vi "Lab Panel V2.9.vi"() -> ()   [LabVIEW 2013]
uses:
  <vilib>/Platform/TimedLoop/XDataNode/timing_clust.ctl
  <vilib>/Platform/TimedLoop/XDataNode/nitl_modes.ctl
  <vilib>/Platform/TimedLoop/XDataNode/wakeup.ctl
  <vilib>/platform/TimedLoop/XDataNode/XDataNode.xnode
  <vilib>/Platform/TimedLoop/XDataNode/XDNodeRunTimeDep.lvlib
panel:
  out "TEMP update":bool
  out "AI update":bool
  in  "stop":bool
  in  "Tab Control 2":T1(tab)
  out "LAB05-2 (SIG)":T2 {"PF" format="%.2f"; "AMPS" format="%.1f"}
  out "LAB05-1 (SIG)":T2 {"PF" format="%.2f"; "AMPS" format="%.1f"}
  out "LAB04-2 (SIG)":T2 {"PF" format="%.2f"; "AMPS" format="%.1f"}
  out "LAB04-1 (SIG)":T2 {"PF" format="%.2f"; "AMPS" format="%.1f"}
  out "LAB03-2 (SIG)":T2 {"PF" format="%.2f"; "AMPS" format="%.1f"}
  out "LAB03-1 (SIG)":T2 {"PF" format="%.2f"; "AMPS" format="%.1f"}
  out "LAB02-2 (SIG)":T2 {"PF" format="%.2f"; "AMPS" format="%.1f"}
  in  "LAB01-1RUN":bool
  in  "LAB05-1 (O/I)":bool
  in  "LAB05-2 (O/I)":bool
  in  "LAB04-1 (O/I)":bool
  in  "LAB04-2 (O/I)":bool
  in  "LAB02-1 (O/I)":bool
  in  "LAB02-2 (O/I)":bool
  in  "LAB01-2 (O/I)":bool
  in  "LAB01-1 (O/I)":bool
  in  "LAB03-1 (O/I)":bool
  in  "LAB05-2 RUN":bool
  in  "LAB05-1 RUN":bool
  in  "LAB04-2 RUN":bool
  in  "LAB04-1 RUN":bool
  in  "LAB03-2 RUN":bool
  in  "LAB03-1 RUN":bool
  in  "LAB02-2 RUN":bool
  in  "LAB02-1 RUN":bool
  in  "LAB01-2 RUN":bool
  in  "LAB05-2 SELECT":T3(radio)
  in  "LAB05-1 SELECT":T3(radio)
  in  "LAB04-2 SELECT":T3(radio)
  in  "LAB04-1 SELECT":T3(radio)
  in  "LAB03-2 SELECT":T3(radio)
  in  "LAB03-1 SELECT":T3(radio)
  in  "LAB02-2 SELECT":T3(radio)
  in  "LAB02-1 SELECT":T3(radio)
  in  "LAB01-2 SELECT":T3(radio)
  in  "LAB01-1 SELECT":T3(radio)
  in  "LAB03-2 (O/I)":bool
  out "LAB01-1 (SIG)":T2 {"PF" format="%.2f"; "AMPS" format="%.1f"}
  out "LAB01-2 (SIG)":T2 {"PF" format="%.2f"; "AMPS" format="%.1f"}
  out "LAB02-1 (SIG)":T2 {"PF" format="%.2f"; "AMPS" format="%.1f"}
  out "LAB05-2 (DISP)":T4 {"MINS" format="%.2g"}
  out "LAB05-1 (DISP)":T4 {"MINS" format="%.2g"}
  out "LAB04-2 (DISP)":T4 {"MINS" format="%.2g"}
  out "LAB04-1 (DISP)":T4 {"MINS" format="%.2g"}
  out "LAB03-2 (DISP)":T4 {"MINS" format="%.2g"}
  out "LAB03-1 (DISP)":T4 {"MINS" format="%.2g"}
  in  "LAB05-2 (SET)":T5
  in  "LAB05-1 (SET)":T5
  in  "LAB04-2 (SET)":T5
  in  "LAB04-1 (SET)":T5
  in  "LAB03-2 (SET)":T5
  in  "LAB03-1 (SET)":T5
  out "LAB02-2 (DISP)":T4 {"MINS" format="%.2g"}
  out "LAB02-1 (DISP)":T4 {"MINS" format="%.2g"}
  in  "LAB02-2 (SET)":T5
  in  "LAB02-1 (SET)":T5
  out "LAB05-2 (RESULT)":bool
  out "LAB05-1 (RESULT)":bool
  out "LAB04-2 (RESULT)":bool
  out "LAB04-1 (RESULT)":bool
  out "LAB03-2 (RESULT)":bool
  out "LAB03-1 (RESULT)":bool
  out "LAB02-2 (RESULT)":bool
  out "LAB02-1 (RESULT)":bool
  out "LAB01-2 (RESULT)":bool
  out "LAB01-1 (RESULT)":bool
  in  "LAB01-1 (SET)":T5
  in  "LAB01-2(SET)":T5
  out "LAB01-1 (DISP)":T4 {"MINS" format="%.2g"}
  out "LAB01-2 (DISP)":T4 {"MINS" format="%.2f"}
  out "LAB05-2 (FAIL)":cluster{"LO":dbl, "HI":dbl}
  out "LAB05-1 (FAIL)":cluster{"LO":dbl, "HI":dbl}
  out "LAB04-2 (FAIL)":cluster{"LO":dbl, "HI":dbl}
  out "LAB04-1 (FAIL)":cluster{"LO":dbl, "HI":dbl}
  out "LAB03-2 (FAIL)":cluster{"LO":dbl, "HI":dbl}
  out "LAB03-1 (FAIL)":cluster{"LO":dbl, "HI":dbl}
  out "LAB02-2 (FAIL)":cluster{"LO":dbl, "HI":dbl}
  out "LAB02-1 (FAIL)":cluster{"LO":dbl, "HI":dbl}
  out "LAB01-2 (FAIL)":cluster{"LO":dbl, "HI":dbl}
  out "LAB01-1 (FAIL)":cluster{"LO":dbl, "HI":dbl}
  out "LAB05-2 (TEMP START)":cluster{"TL":dbl, "TN":dbl}
  out "LAB04-2 (TEMP START)":cluster{"TL":dbl, "TN":dbl}
  out "LAB03-2 (TEMP START)":cluster{"TL":dbl, "TN":dbl}
  out "LAB02-2 (TEMP START)":cluster{"TL":dbl, "TN":dbl}
  out "LAB01-2 (TEMP START)":cluster{"TL":dbl, "TN":dbl}
  out "LAB05-1 (TEMP START)":cluster{"TL":dbl, "TN":dbl}
  out "LAB04-1 (TEMP START)":cluster{"TL":dbl, "TN":dbl}
  out "LAB03-1 (TEMP START)":cluster{"TL":dbl, "TN":dbl}
  out "LAB02-1 (TEMP START)":cluster{"TL":dbl, "TN":dbl}
  out "LAB01-1 (TEMP START)":cluster{"TL":dbl, "TN":dbl}
  in  "JIG ON TIME (S)":dbl=1.0 min=1.0 max=10.0 step=0.5 format="%.1g"
  in  "JIG OFF TIME (S)":dbl=2.0 min=2.0 max=10.0 step=0.5 format="%.1g"
  out "LAB01-1 (JIG)":bool
  out "LAB01-2 (JIG)":bool
  out "LAB02-1 (JIG)":bool
  out "LAB02-2 (JIG)":bool
  out "LAB03-1 (JIG)":bool
  out "LAB03-2 (JIG)":bool
  out "LAB04-1 (JIG)":bool
  out "LAB04-2 (JIG)":bool
  out "LAB05-1 (JIG)":bool
  out "LAB05-2 (JIG)":bool
  out "LAB01 (CAL)":T6 {"2 (TN) cal" min=0.0 step=0.01 format="%.2f"; "2 (TL) cal" min=0.0 step=0.01 format="%.2f"; "2 (PF) cal" min=0.0 step=0.01 format="%.2f"; "2 (V) cal" min=0.0 step=0.01 format="%.2f"; "2 (A) cal" min=0.0 step=0.01 format="%.2f"; "1 (TN) cal" min=0.0 step=0.01 format="%.2f"; "1 (TL) cal" min=0.0 step=0.01 format="%.2f"; "1 (PF) cal" min=0.0 step=0.01 format="%.2f"; "1 (V) cal" min=0.0 step=0.01 format="%.2f"; "1  (A) cal" min=0.0 step=0.01 format="%.2f"}
  out "LAB03 (CAL)":T6 {"2 (TN) cal" min=0.0 step=0.01 format="%.2f"; "2 (TL) cal" min=0.0 step=0.01 format="%.2f"; "2 (PF) cal" min=0.0 step=0.01 format="%.2f"; "2 (V) cal" min=0.0 step=0.01 format="%.2f"; "2 (A) cal" min=0.0 step=0.01 format="%.2f"; "1 (TN) cal" min=0.0 step=0.01 format="%.2f"; "1 (TL) cal" min=0.0 step=0.01 format="%.2f"; "1 (PF) cal" min=0.0 step=0.01 format="%.2f"; "1 (V) cal" min=0.0 step=0.01 format="%.2f"; "1  (A) cal" min=0.0 step=0.01 format="%.2f"}
  out "LAB02 (CAL)":T7 {"2 (TN) cal" min=0.0 step=0.01 format="%.2f"; "2 (TL) cal" min=0.0 step=0.01 format="%.2f"; "2 (PF) cal" min=0.0 step=0.01 format="%.2f"; "2 (V) cal" min=0.0 step=0.01 format="%.2f"; "2 (A) cal" min=0.0 step=0.01 format="%.2f"; "1 (TN) cal" min=0.0 step=0.01 format="%.2f"; "1 (TL) cal" min=0.0 step=0.01 format="%.2f"; "1 (PF) cal" min=0.0 step=0.01 format="%.2f"; "1 (V) cal" min=0.0 step=0.01 format="%.2f"; "1 (A) cal" min=0.0 step=0.01 format="%.2f"}
  out "LAB05 (CAL)":T6 {"2 (TN) cal" min=0.0 step=0.01 format="%.2f"; "2 (TL) cal" min=0.0 step=0.01 format="%.2f"; "2 (PF) cal" min=0.0 step=0.01 format="%.2f"; "2 (V) cal" min=0.0 step=0.01 format="%.2f"; "2 (A) cal" min=0.0 step=0.01 format="%.2f"; "1 (TN) cal" min=0.0 step=0.01 format="%.2f"; "1 (TL) cal" min=0.0 step=0.01 format="%.2f"; "1 (PF) cal" min=0.0 step=0.01 format="%.2f"; "1 (V) cal" min=0.0 step=0.01 format="%.2f"; "1  (A) cal" min=0.0 step=0.01 format="%.2f"}
  out "LAB04 (CAL)":T6 {"2 (TN) cal" min=0.0 step=0.01 format="%.2f"; "2 (TL) cal" min=0.0 step=0.01 format="%.2f"; "2 (PF) cal" min=0.0 step=0.01 format="%.2f"; "2 (V) cal" min=0.0 step=0.01 format="%.2f"; "2 (A) cal" min=0.0 step=0.01 format="%.2f"; "1 (TN) cal" min=0.0 step=0.01 format="%.2f"; "1 (TL) cal" min=0.0 step=0.01 format="%.2f"; "1 (PF) cal" min=0.0 step=0.01 format="%.2f"; "1 (V) cal" min=0.0 step=0.01 format="%.2f"; "1  (A) cal" min=0.0 step=0.01 format="%.2f"}
  out "calibration file error out":errorcluster
  in  "CALIBRATE":bool
  in  "Tab Control":T8(tab)
  out "LAB01-2 (GRAPH)":dynamicdata(graph)
  out "LAB01-1 (GRAPH)":dynamicdata(graph)
  out "LAB02-2 (GRAPH)":dynamicdata(graph)
  out "LAB02-1 (GRAPH)":dynamicdata(graph)
  out "LAB03-2 (GRAPH)":dynamicdata(graph)
  out "LAB03-1 (GRAPH)":dynamicdata(graph)
  out "LAB04-2 (GRAPH)":dynamicdata(graph)
  out "LAB04-1 (GRAPH)":dynamicdata(graph)
  out "LAB05-2 (GRAPH)":dynamicdata(graph)
  out "LAB05-1 (GRAPH)":dynamicdata(graph)
  out "LAB05 TEMP":T9
  out "LAB04 TEMP":T9
  out "LAB02 TEMP":T9
  out "LAB01 TEMP":T9
  out "LAB03 TEMP":T9
  out "Analog Error Array":errorcluster[](array[cluster])
  out "AI loop time":dbl format="%.6g"
  out "loops":dbl
  in  "loop  delay(mS)":dbl
  out "on loops":dbl
  out "off loops":dbl
  out "jig cycle":dbl
  out "LAB01-1 (TDMS)":refnum<k34>
  out "data file error":errorcluster
  out "LAB02-1 (TDMS)":refnum<k34>
  out "LAB01-2 (TDMS)":refnum<k34>
  out "LAB02-2 (TDMS)":refnum<k34>
  out "LAB03-1 (TDMS)":refnum<k34>
  out "LAB03-2 (TDMS)":refnum<k34>
  out "LAB04-1 (TDMS)":refnum<k34>
  out "LAB04-2 (TDMS)":refnum<k34>
  out "LAB05-1 (TDMS)":refnum<k34>
  out "LAB05-2 (TDMS)":refnum<k34>
  # "LAB01"
  # "LAB02"
  # "LAB05"
  # "LAB03"
  # "LAB04"
  # "LAB01"
  # "LAB02"
  # "LAB03"
  # "LAB04"
  # "LAB05"
  # "JIG SET"
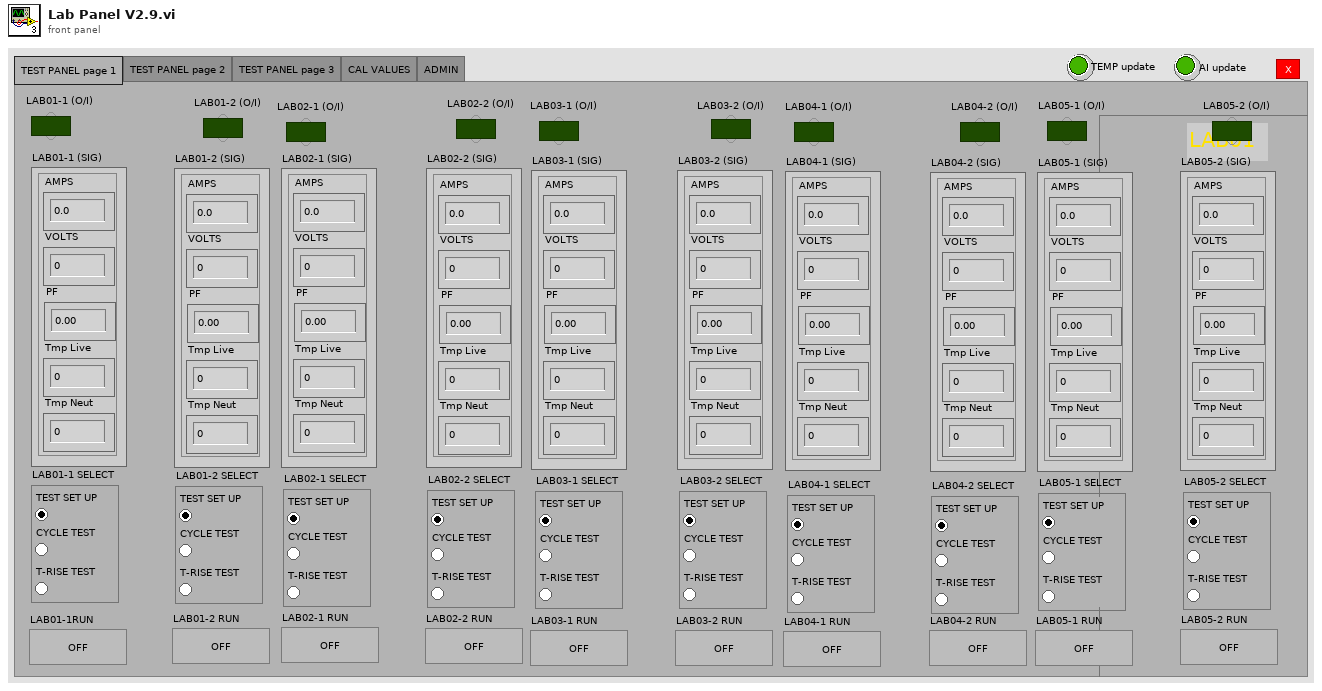
[diagram p1: front panel]
types:
  T1 = enum32{"TEST PANEL page 1", "TEST PANEL page 2", "TEST PANEL page 3", "CAL VALUES", "ADMIN"}
  T2 = cluster{"AMPS":dbl, "VOLTS":dbl, "PF":dbl, "Tmp Live":dbl, "Tmp Neut":dbl}
  T3 = enum32{"TEST SET UP", "CYCLE TEST", "T-RISE TEST"}
  T4 = cluster{"CYCLE":dbl, "MINS":dbl, "STATUS":string}
  T5 = cluster{"NAME":string, "DESCRIPTION":string, "CYCLES":dbl, "T-RISE mins":dbl, "T-RISE deg C":dbl}
  T6 = cluster{"1  (A) cal":dbl, "1 (V) cal":dbl, "1 (PF) cal":dbl, "1 (TL) cal":dbl, "1 (TN) cal":dbl, "2 (A) cal":dbl, "2 (V) cal":dbl, "2 (PF) cal":dbl, "2 (TL) cal":dbl, "2 (TN) cal":dbl}
  T7 = cluster{"1 (A) cal":dbl, "1 (V) cal":dbl, "1 (PF) cal":dbl, "1 (TL) cal":dbl, "1 (TN) cal":dbl, "2 (A) cal":dbl, "2 (V) cal":dbl, "2 (PF) cal":dbl, "2 (TL) cal":dbl, "2 (TN) cal":dbl}
  T8 = enum32{"LAB01", "LAB02", "LAB03", "LAB04", "LAB05", "TEMPERATURE", "ERROR"}
  T9 = cluster{"T1 Live":dbl, "T1 Neut":dbl, "T2 Live":dbl, "T2 Neut":dbl, "ID":dbl, "ER":dbl}
  T10 = enum8{"Enabled", "Disabled", "Disabled and Grayed Out"}
  T11 = typedef "XDNodeRunTimeDep.lvlib/timing_clust.ctl" = cluster{"Expected End [f-1]":u64, "Actual End [f-1]":u64, "Finished Late? [f-1]":bool, "Expected End [i-1]":u64, "Actual End [i-1]":u64, "Finished Late? [i-1]":bool, "Expected Start [i]":u64, "Actual Start [i]":u64, "Expected Start [f]":u64, "Actual Start [f]":u64, "Source Name":string, "Structure Name":string, "Period":i64, "Deadline":i64, "Offset":i64, "Start":i64, "Priority":i32, "Timeout":i32, "Mode":T12, "Wakeup Reason":T13, "Error":errorcluster, "Source Type":string, "Secondary Source Type":string, "Global End Time":u64, "Global Start Time":u64, "Frame Duration":u64, "Iteration Duration":u64, "Assigned CPU":i32, "I/O Scan Engine Mode":u32}
  T12 = typedef "XDNodeRunTimeDep.lvlib/nitl_modes.ctl" = enum32{"No Change", "Process missed periods, maintain original phase", "Discard missed periods, maintain original phase", "Process missed periods, ignore original phase", "Discard missed periods, ignore original phase"}
  T13 = typedef "XDNodeRunTimeDep.lvlib/wakeup.ctl" = enum32{"Normal", "Aborted", "Asynchronous wakeup", "Timing source error", "Timed loop error", "Timeout"}
  T14 = enum16{"open", "open or create", "create or replace", "create", "open (read-only)"}
  T15 = cluster{"T1":dbl, "T2":dbl, "T3":dbl, "T4":dbl, "ID":dbl, "ER":dbl}
  T16 = cluster{"LAB01-1 (A)":dbl, "LAB01-1 (V)":dbl, "LAB01-1 (PF)":dbl, "LAB01-2 (A)":dbl, "LAB01-2 (V)":dbl, "LAB01-2 (PF)":dbl}
  T17 = cluster{"LAB02-1 (A)":dbl, "LAB02-1 (V)":dbl, "LAB02-1 (PF)":dbl, "LAB02-2 (A)":dbl, "LAB02-2 (V)":dbl, "LAB02-2 (PF)":dbl}
  T18 = cluster{"LAB03-1 (A)":dbl, "LAB03-1 (V)":dbl, "LAB03-1 (PF)":dbl, "LAB03-2 (A)":dbl, "LAB03-2 (V)":dbl, "LAB03-2 (PF)":dbl}
  T19 = cluster{"LAB04-1 (A)":dbl, "LAB04-1 (V)":dbl, "LAB04-1 (PF)":dbl, "LAB04-2 (A)":dbl, "LAB04-2 (V)":dbl, "LAB04-2 (PF)":dbl}
  T20 = cluster{"LAB05-1 (A)":dbl, "LAB05-1 (V)":dbl, "LAB05-1 (PF)":dbl, "LAB05-2 (A)":dbl, "LAB05-2 (V)":dbl, "LAB05-2 (PF)":dbl}
  T21 = cluster{"LAB01-1 (FAIL)":cluster{"LO":dbl, "HI":dbl}, "LAB01-1 (SIG)":cluster{"AMPS":dbl, "VOLTS":dbl, "PF":dbl, "Tmp Live":dbl, "Tmp Neut":dbl}, "LAB01-1 (TEMP START)":cluster{"TL":dbl, "TN":dbl}, "LAB01-1 (DISP)":cluster{"CYCLE":dbl, "MINS":dbl, "STATUS":string}, "LAB01-1 (SET)":cluster{"NAME":string, "DESCRIPTION":string, "CYCLES":dbl, "T-RISE mins":dbl, "T-RISE deg C":dbl}, "LAB01-1 (TDMS)":refnum<k34>}
  T22 = cluster{"LAB01-2 (FAIL)":cluster{"LO":dbl, "HI":dbl}, "LAB01-2 (SIG)":cluster{"AMPS":dbl, "VOLTS":dbl, "PF":dbl, "Tmp Live":dbl, "Tmp Neut":dbl}, "LAB01-2 (TEMP START)":cluster{"TL":dbl, "TN":dbl}, "LAB01-2 (DISP)":cluster{"CYCLE":dbl, "MINS":dbl, "STATUS":string}, "LAB01-2(SET)":cluster{"NAME":string, "DESCRIPTION":string, "CYCLES":dbl, "T-RISE mins":dbl, "T-RISE deg C":dbl}, "LAB01-2 (TDMS)":refnum<k34>}
  T23 = cluster{"LAB02-1 (FAIL)":cluster{"LO":dbl, "HI":dbl}, "LAB02-1 (SIG)":cluster{"AMPS":dbl, "VOLTS":dbl, "PF":dbl, "Tmp Live":dbl, "Tmp Neut":dbl}, "LAB02-1 (TEMP START)":cluster{"TL":dbl, "TN":dbl}, "LAB02-1 (DISP)":cluster{"CYCLE":dbl, "MINS":dbl, "STATUS":string}, "LAB02-1 (SET)":cluster{"NAME":string, "DESCRIPTION":string, "CYCLES":dbl, "T-RISE mins":dbl, "T-RISE deg C":dbl}, "LAB02-1 (TDMS)":refnum<k34>}
  T24 = cluster{"LAB02-2 (FAIL)":cluster{"LO":dbl, "HI":dbl}, "LAB02-2 (SIG)":cluster{"AMPS":dbl, "VOLTS":dbl, "PF":dbl, "Tmp Live":dbl, "Tmp Neut":dbl}, "LAB02-2 (TEMP START)":cluster{"TL":dbl, "TN":dbl}, "LAB02-2 (DISP)":cluster{"CYCLE":dbl, "MINS":dbl, "STATUS":string}, "LAB02-2 (SET)":cluster{"NAME":string, "DESCRIPTION":string, "CYCLES":dbl, "T-RISE mins":dbl, "T-RISE deg C":dbl}, "LAB02-2 (TDMS)":refnum<k34>}
  T25 = cluster{"LAB03-1 (FAIL)":cluster{"LO":dbl, "HI":dbl}, "LAB03-1 (SIG)":cluster{"AMPS":dbl, "VOLTS":dbl, "PF":dbl, "Tmp Live":dbl, "Tmp Neut":dbl}, "LAB03-1 (TEMP START)":cluster{"TL":dbl, "TN":dbl}, "LAB03-1 (DISP)":cluster{"CYCLE":dbl, "MINS":dbl, "STATUS":string}, "LAB03-1 (SET)":cluster{"NAME":string, "DESCRIPTION":string, "CYCLES":dbl, "T-RISE mins":dbl, "T-RISE deg C":dbl}, "LAB03-1 (TDMS)":refnum<k34>}
  T26 = cluster{"LAB03-2 (FAIL)":cluster{"LO":dbl, "HI":dbl}, "LAB03-2 (SIG)":cluster{"AMPS":dbl, "VOLTS":dbl, "PF":dbl, "Tmp Live":dbl, "Tmp Neut":dbl}, "LAB03-2 (TEMP START)":cluster{"TL":dbl, "TN":dbl}, "LAB03-2 (DISP)":cluster{"CYCLE":dbl, "MINS":dbl, "STATUS":string}, "LAB03-2 (SET)":cluster{"NAME":string, "DESCRIPTION":string, "CYCLES":dbl, "T-RISE mins":dbl, "T-RISE deg C":dbl}, "LAB03-2 (TDMS)":refnum<k34>}
  T27 = cluster{"LAB04-1 (FAIL)":cluster{"LO":dbl, "HI":dbl}, "LAB04-1 (SIG)":cluster{"AMPS":dbl, "VOLTS":dbl, "PF":dbl, "Tmp Live":dbl, "Tmp Neut":dbl}, "LAB04-1 (TEMP START)":cluster{"TL":dbl, "TN":dbl}, "LAB04-1 (DISP)":cluster{"CYCLE":dbl, "MINS":dbl, "STATUS":string}, "LAB04-1 (SET)":cluster{"NAME":string, "DESCRIPTION":string, "CYCLES":dbl, "T-RISE mins":dbl, "T-RISE deg C":dbl}, "LAB04-1 (TDMS)":refnum<k34>}
  T28 = cluster{"LAB04-2 (FAIL)":cluster{"LO":dbl, "HI":dbl}, "LAB04-2 (SIG)":cluster{"AMPS":dbl, "VOLTS":dbl, "PF":dbl, "Tmp Live":dbl, "Tmp Neut":dbl}, "LAB04-2 (TEMP START)":cluster{"TL":dbl, "TN":dbl}, "LAB04-2 (DISP)":cluster{"CYCLE":dbl, "MINS":dbl, "STATUS":string}, "LAB04-2 (SET)":cluster{"NAME":string, "DESCRIPTION":string, "CYCLES":dbl, "T-RISE mins":dbl, "T-RISE deg C":dbl}, "LAB04-2 (TDMS)":refnum<k34>}
  T29 = cluster{"LAB05-1 (FAIL)":cluster{"LO":dbl, "HI":dbl}, "LAB05-1 (SIG)":cluster{"AMPS":dbl, "VOLTS":dbl, "PF":dbl, "Tmp Live":dbl, "Tmp Neut":dbl}, "LAB05-1 (TEMP START)":cluster{"TL":dbl, "TN":dbl}, "LAB05-1 (DISP)":cluster{"CYCLE":dbl, "MINS":dbl, "STATUS":string}, "LAB05-1 (SET)":cluster{"NAME":string, "DESCRIPTION":string, "CYCLES":dbl, "T-RISE mins":dbl, "T-RISE deg C":dbl}, "LAB05-1 (TDMS)":refnum<k34>}
  T30 = cluster{"LAB05-2 (FAIL)":cluster{"LO":dbl, "HI":dbl}, "LAB05-2 (SIG)":cluster{"AMPS":dbl, "VOLTS":dbl, "PF":dbl, "Tmp Live":dbl, "Tmp Neut":dbl}, "LAB05-2 (TEMP START)":cluster{"TL":dbl, "TN":dbl}, "LAB05-2 (DISP)":cluster{"CYCLE":dbl, "MINS":dbl, "STATUS":string}, "LAB05-2 (SET)":cluster{"NAME":string, "DESCRIPTION":string, "CYCLES":dbl, "T-RISE mins":dbl, "T-RISE deg C":dbl}, "LAB05-2 (TDMS)":refnum<k34>}
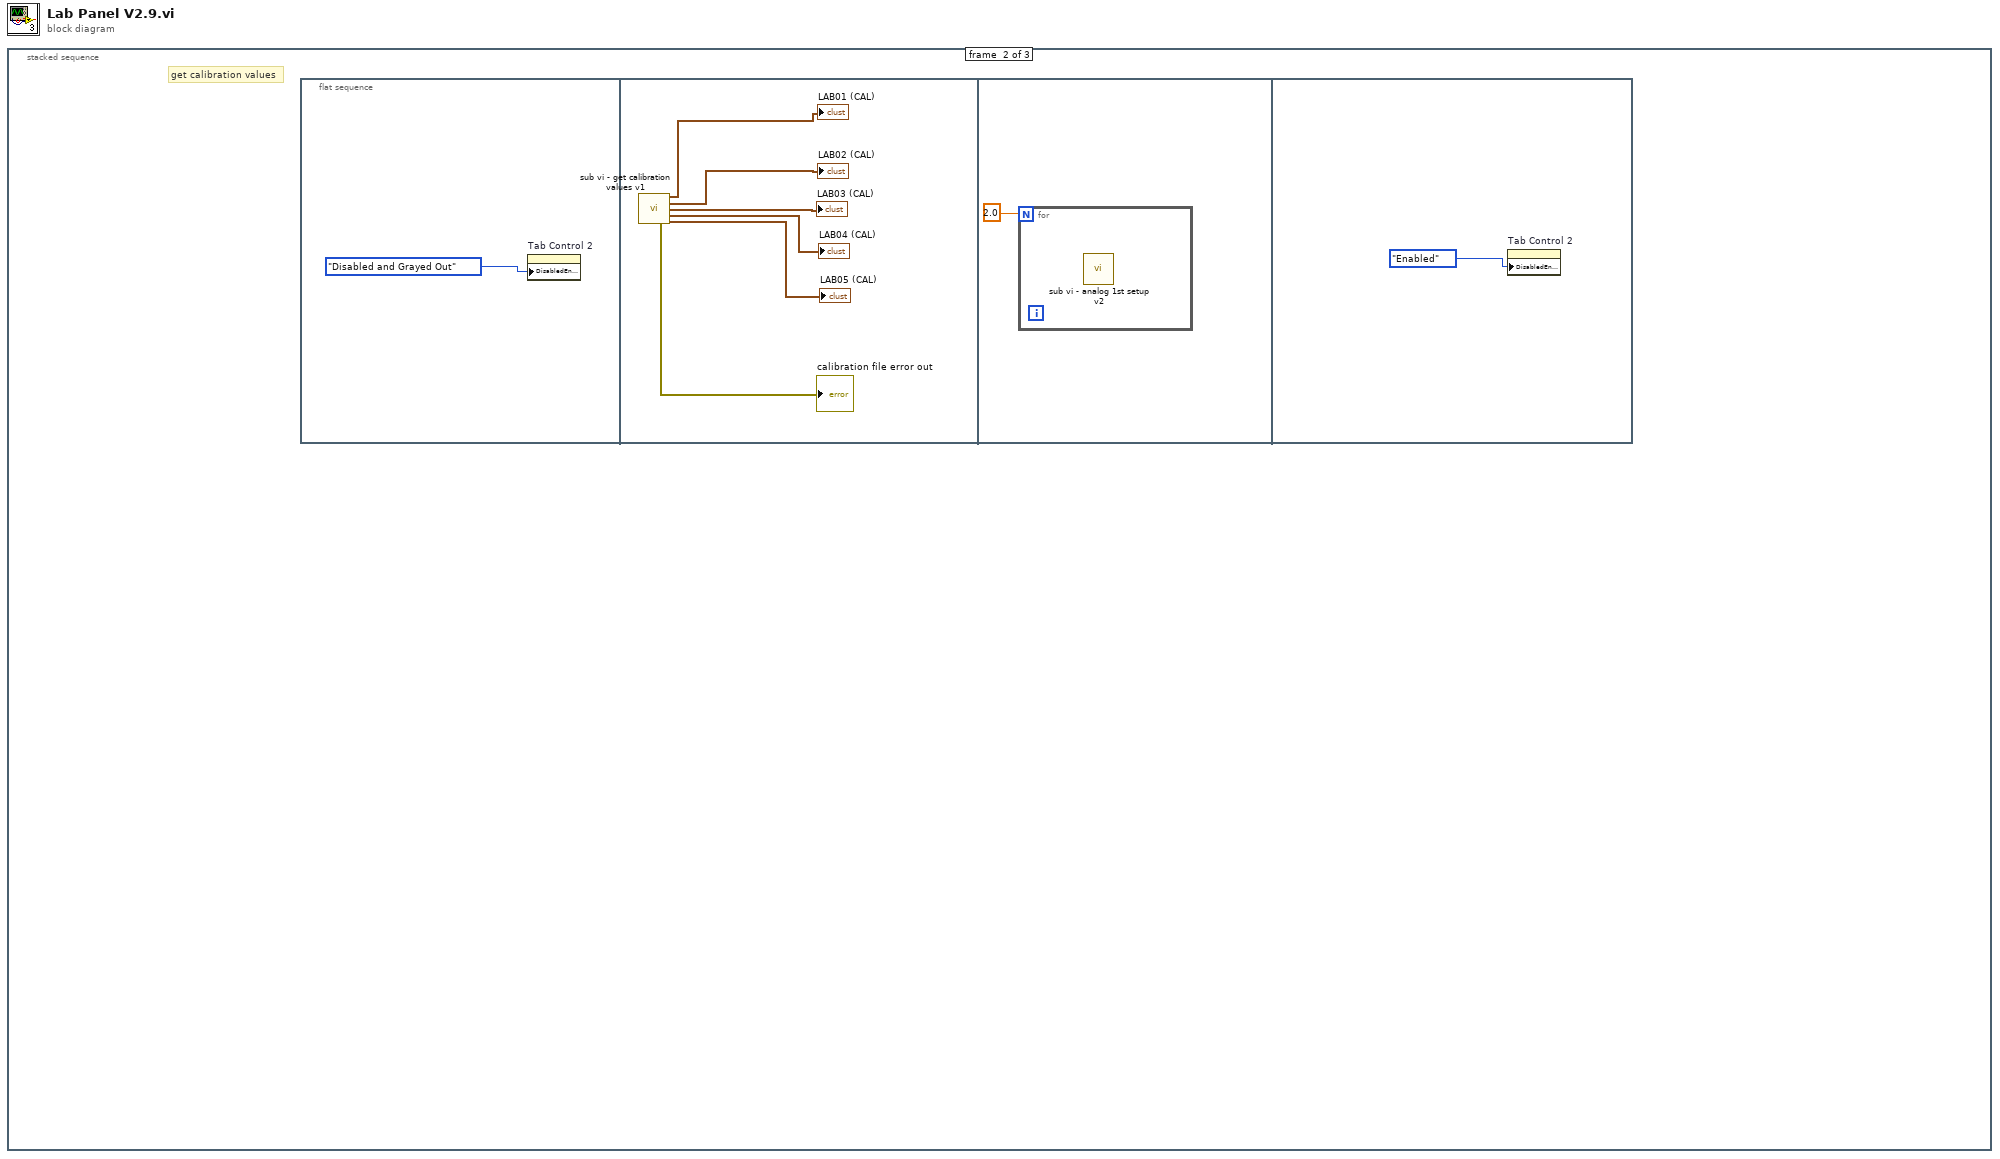
[diagram p0: block diagram]
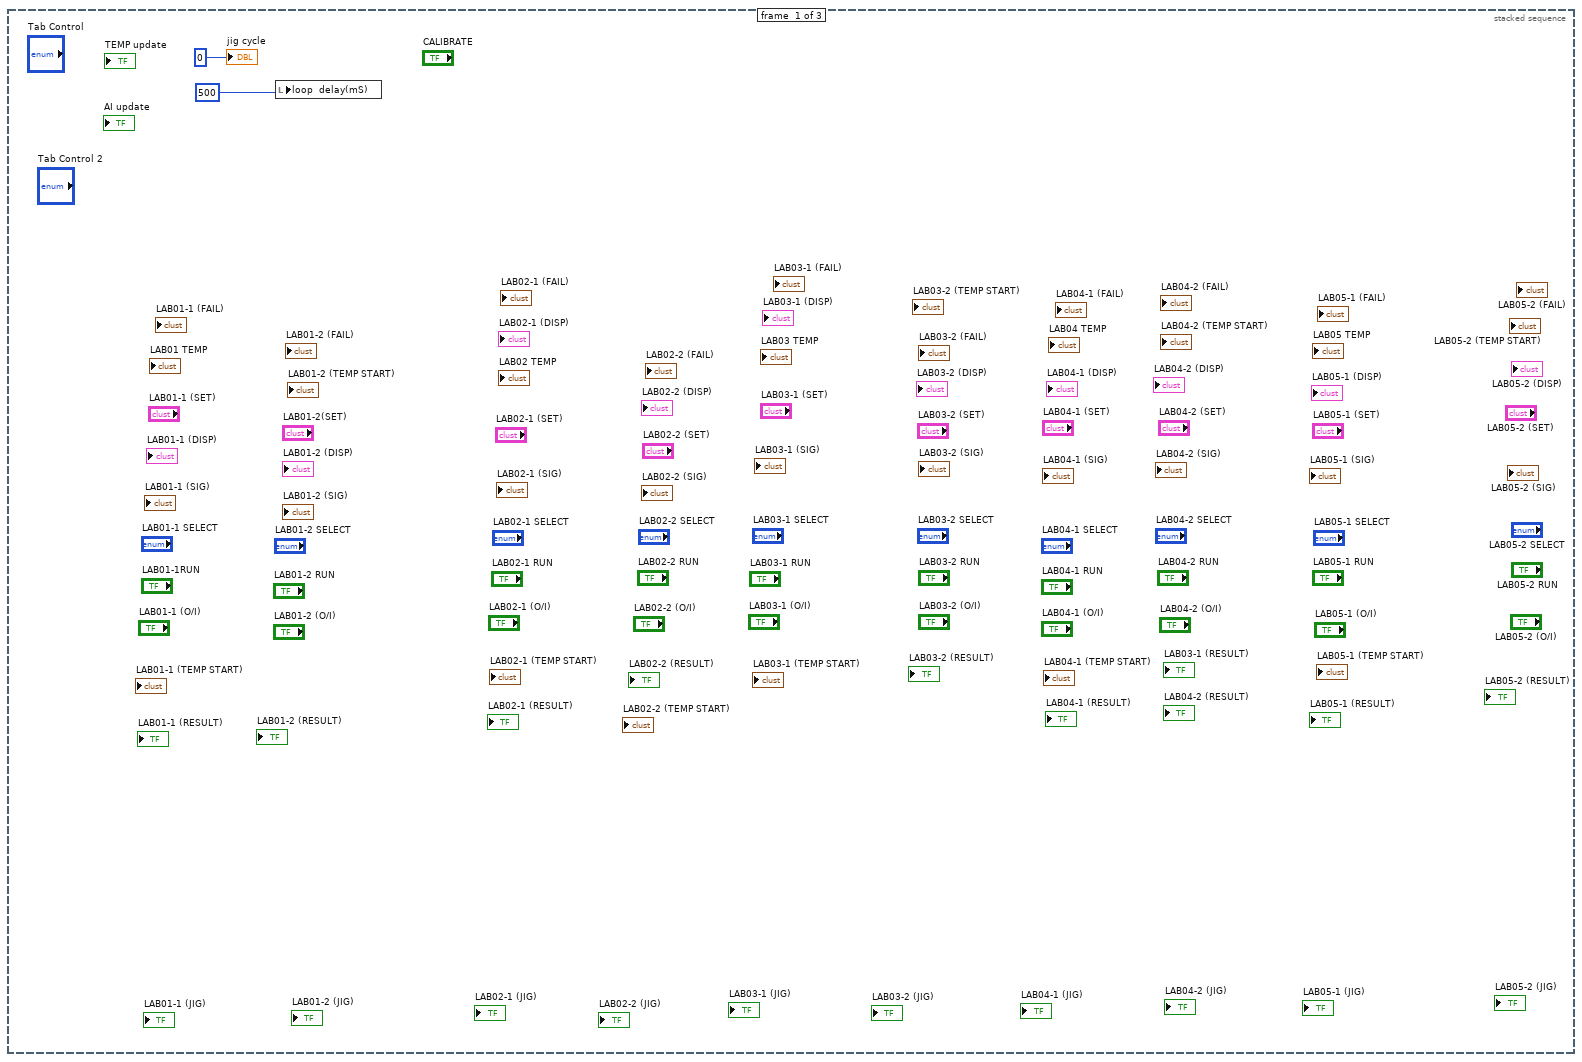
[diagram p2: hidden frame]
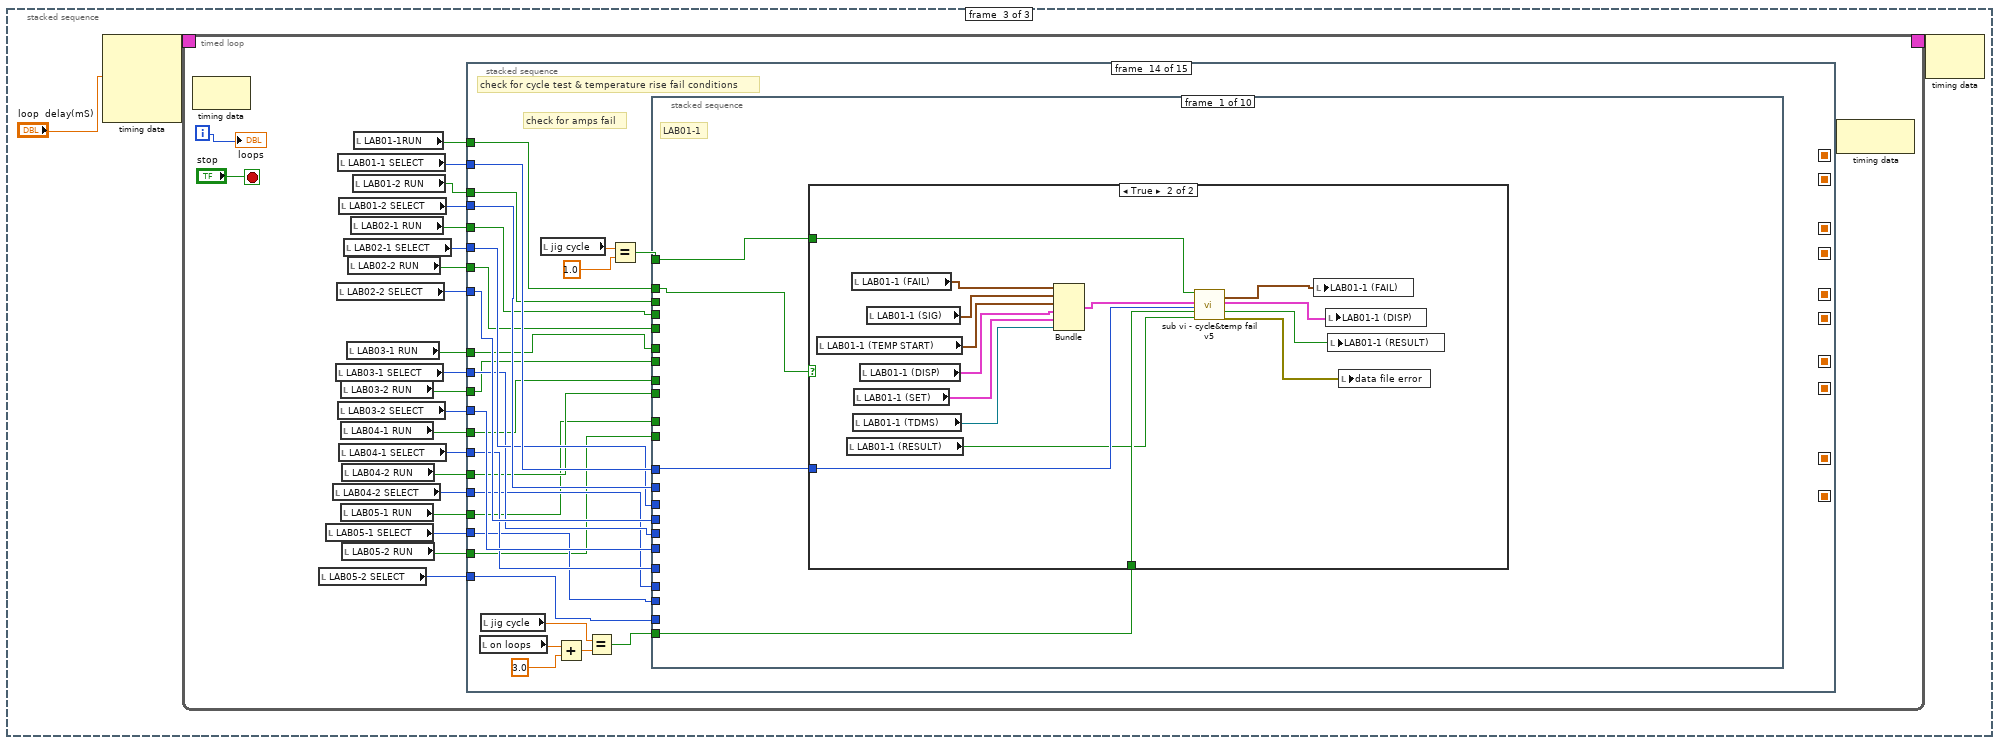
[diagram p3: hidden frame]
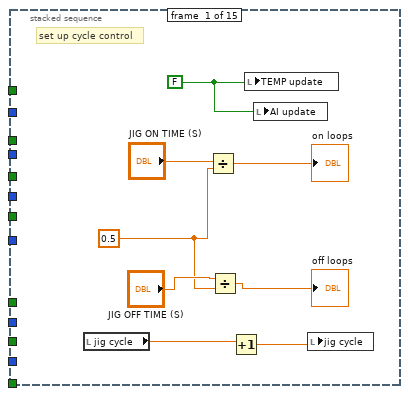
[diagram p4: hidden frame]
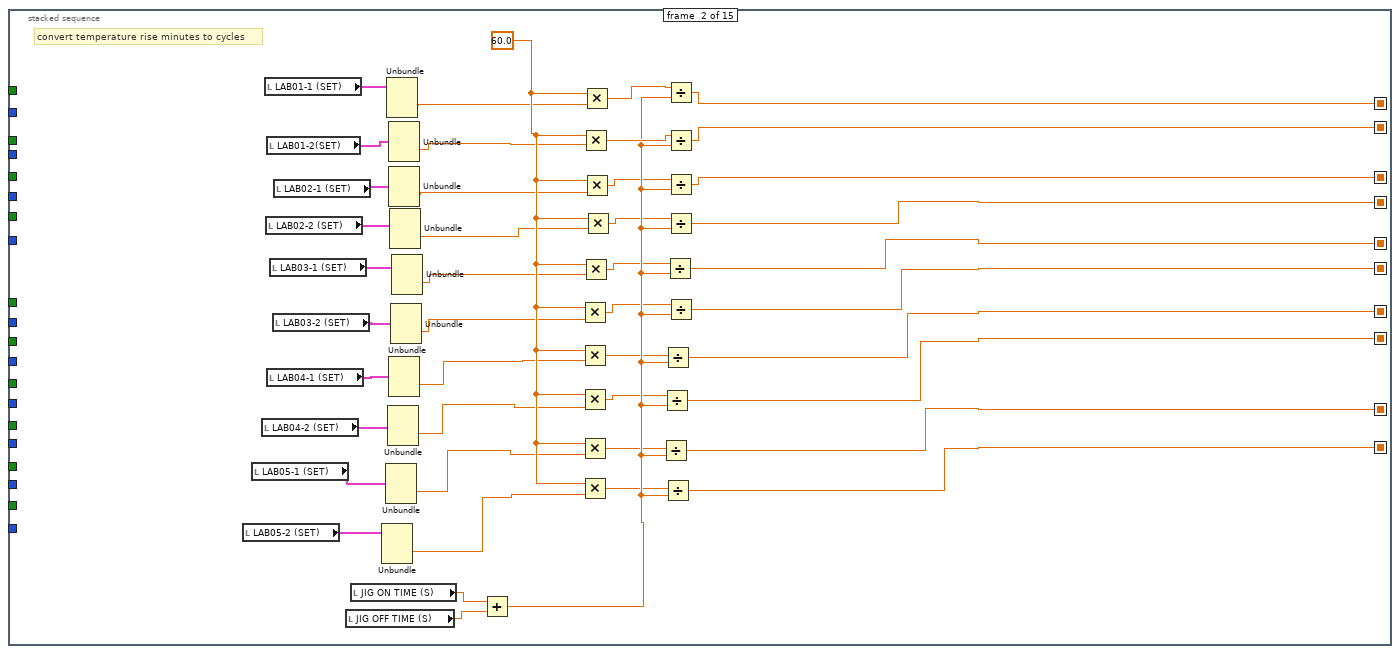
[diagram p5: hidden frame]
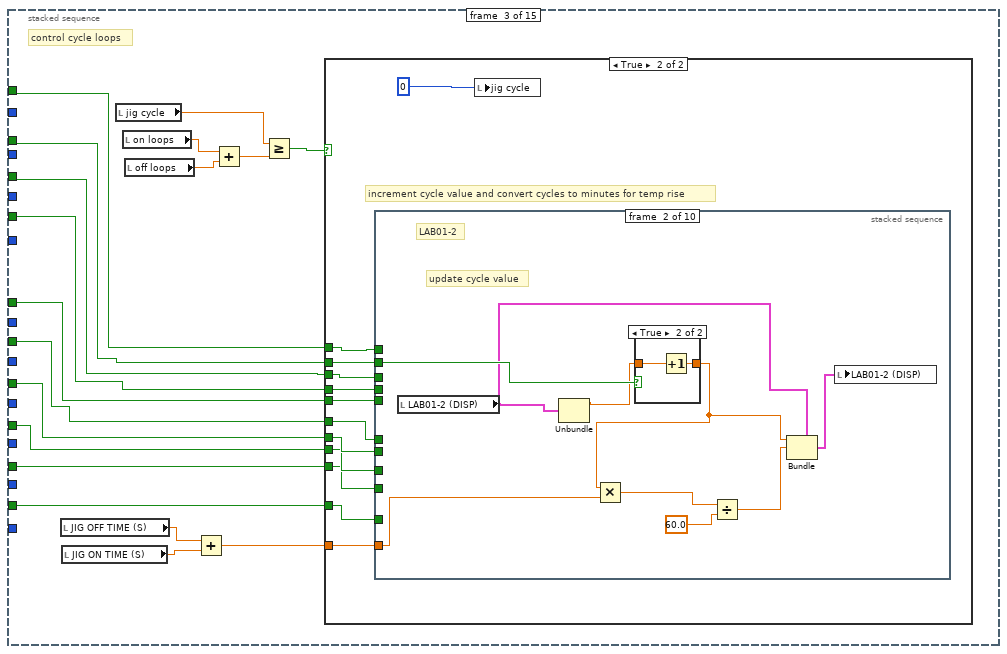
[diagram p6: hidden frame]
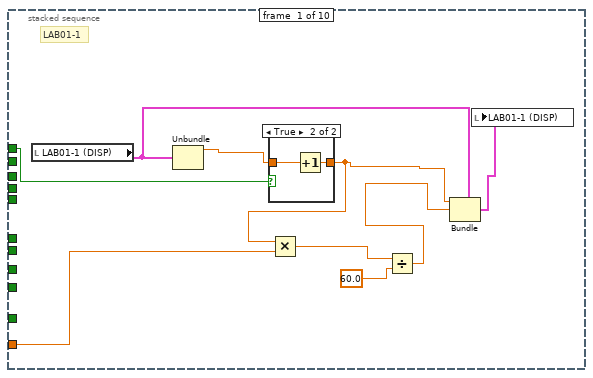
[diagram p8: hidden frame]
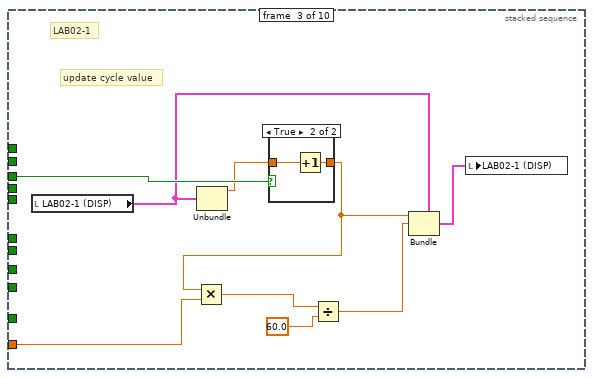
[diagram p11: hidden frame]
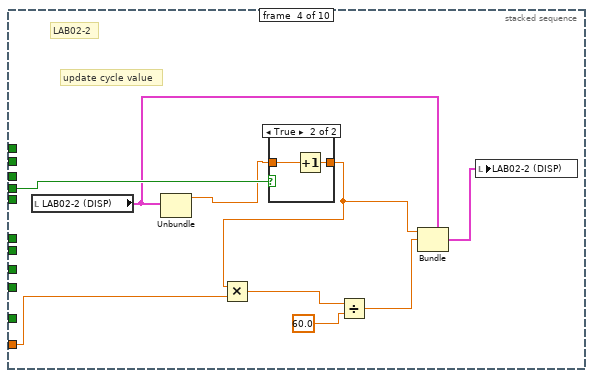
[diagram p13: hidden frame]
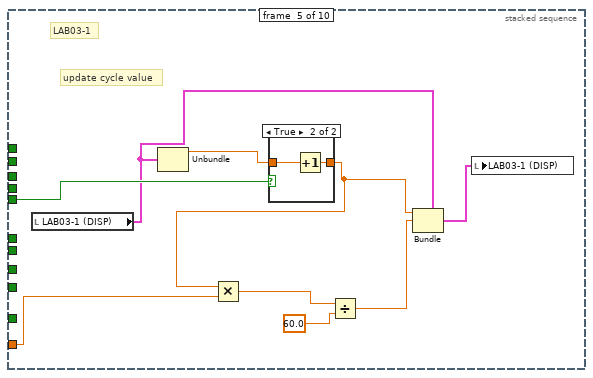
[diagram p15: hidden frame]
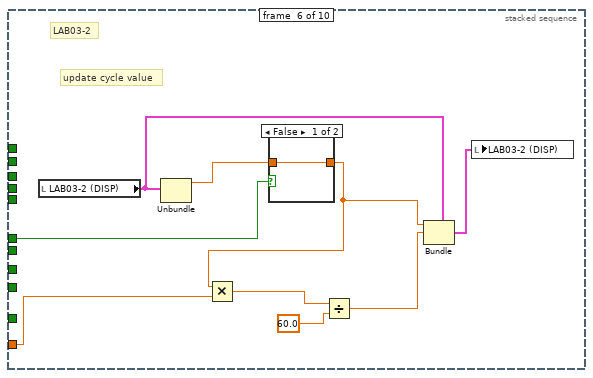
[diagram p17: hidden frame]
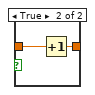
[diagram p18: hidden frame]
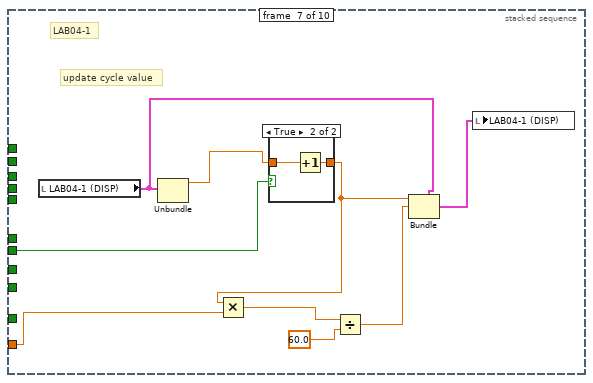
[diagram p19: hidden frame]
diagram:
  n1 = stacked-sequence {
    frame #0 {
      n2 = local write "loop  delay(mS)"(500) -> ()
      "jig cycle" <- 0
    }
    frame #1 {
      # "get calibration values"
      n3 = flat-sequence {
        frame #0 {
          n4 = property on="Tab Control 2" class="TabCtl (strict)"("DisabledEnum"=T10."Disabled and Grayed Out" ("Disabled")) -> ()  [unwired: 2 in, 2 out]
        }
        frame #1 {
          n5 = call "sub vi - get calibration values v1.vi"() -> ("LAB01 (CAL)"=→"LAB01 (CAL)":T6, "LAB02 (CAL)"=→"LAB02 (CAL)":T7, "LAB03 (CAL)"=→"LAB03 (CAL)":T6, "LAB04 (CAL)"=→"LAB04 (CAL)":T6, "calibration file error out"=→"calibration file error out":errorcluster, "LAB05 (CAL)"=→"LAB05 (CAL)":T6)  [unwired: 10 in]
        }
        frame #2 {
          n6 = for {
            N: 2.0 -> [_]
            n7 = call "sub vi - analog 1st setup v2.vi"() -> ()  [unwired: 14 in, 2 out]
          }
        }
        frame #3 {
          n8 = property on="Tab Control 2" class="TabCtl (strict)"("DisabledEnum"=T10."Enabled" ("Disabled")) -> ()  [unwired: 2 in, 2 out]
        }
      }
    }
    frame #2 {
      n9 = node-c288("loop  delay(mS)") -> (w14:T11)  [unwired: 3 in]
      n10 = timed-loop {
        timing: w14 -> [_]
        timing-out: [_] -> w13
        i -> [w36]
        stop <- "stop" stop-if-true
        n11 = node-c288() -> ()  [unwired: 1 in, 1 out]
        n12 = local read "LAB05-2 SELECT"() -> (w15:T3)
        n13 = local read "LAB05-1 SELECT"() -> (w16:T3)
        n14 = local read "LAB04-2 SELECT"() -> (w17:T3)
        n15 = local read "LAB03-1 SELECT"() -> (w20:T3)
        n16 = local read "LAB02-2 SELECT"() -> (w21:T3)
        n17 = local read "LAB01-1 SELECT"() -> (w24:T3)
        n18 = local read "LAB03-2 SELECT"() -> (w19:T3)
        n19 = local read "LAB01-2 SELECT"() -> (w23:T3)
        n20 = local read "LAB04-1 SELECT"() -> (w18:T3)
        n21 = local read "LAB03-2 RUN"() -> (w29:bool)
        n22 = local read "LAB04-1 RUN"() -> (w28:bool)
        n23 = local read "LAB05-1 RUN"() -> (w26:bool)
        n24 = local read "LAB04-2 RUN"() -> (w27:bool)
        n25 = local read "LAB05-2 RUN"() -> (w25:bool)
        n26 = local read "LAB02-1 SELECT"() -> (w22:T3)
        n27 = local read "LAB03-1 RUN"() -> (w30:bool)
        n28 = local read "LAB02-2 RUN"() -> (w31:bool)
        n29 = local read "LAB02-1 RUN"() -> (w32:bool)
        n30 = local read "LAB01-2 RUN"() -> (w33:bool)
        n31 = local read "LAB01-1RUN"() -> (w34:bool)
        n32 = stacked-sequence {
          seq-local: [_ w88 _ _ _ _ _ _ _ _ _ _ _ _ _] -> [_ _ _ _ _ w1467 _ _ _ _ _ _ _ _ _]
          seq-local: [_ w87 _ _ _ _ _ _ _ _ _ _ _ _ _] -> [_ _ _ _ _ _ _ _ _ _ _ _ _ _ _]
          seq-local: [_ w74 _ _ _ _ _ _ _ _ _ _ _ _ _] -> [_ _ _ _ _ _ _ _ _ _ _ _ _ _ _]
          seq-local: [_ w73 _ _ _ _ _ _ _ _ _ _ _ _ _] -> [_ _ _ _ _ _ _ _ _ _ _ _ _ _ _]
          seq-local: [_ w72 _ _ _ _ _ _ _ _ _ _ _ _ _] -> [_ _ _ _ _ _ _ _ _ _ _ _ _ _ _]
          seq-local: [_ w71 _ _ _ _ _ _ _ _ _ _ _ _ _] -> [_ _ _ _ _ _ _ _ _ _ _ _ _ _ _]
          seq-local: [_ w70 _ _ _ _ _ _ _ _ _ _ _ _ _] -> [_ _ _ _ _ _ _ _ _ _ _ _ _ _ _]
          seq-local: [_ w69 _ _ _ _ _ _ _ _ _ _ _ _ _] -> [_ _ _ _ _ _ _ _ _ _ _ _ _ _ _]
          seq-local: [_ w68 _ _ _ _ _ _ _ _ _ _ _ _ _] -> [_ _ _ _ _ _ _ _ _ _ _ _ _ _ _]
          seq-local: [_ w67 _ _ _ _ _ _ _ _ _ _ _ _ _] -> [_ _ _ _ _ _ _ _ _ _ _ _ _ _ _]
          tunnel: w34 -> [_ _ w104 w260 w1067 w1478 w1788 w1859 _ _ _ _ w2363 w2851 _]
          tunnel: w33 -> [_ _ w103 w258 w1066 w1477 w1787 w1860 _ _ _ _ w2362 w2849 _]
          tunnel: w32 -> [_ _ w102 w256 w1065 w1476 w1786 w1858 _ _ _ _ w2361 w2847 _]
          tunnel: w31 -> [_ _ w101 w254 w1064 w1475 w1785 w1857 _ _ _ _ w2360 w2845 _]
          tunnel: w30 -> [_ _ w100 w252 w1063 w1474 w1784 w1856 _ _ _ _ w2359 w2843 _]
          tunnel: w29 -> [_ _ w99 w250 w1062 w1473 w1783 w1855 _ _ _ _ w2358 w2841 _]
          tunnel: w28 -> [_ _ w98 w248 w1061 w1472 w1782 w1854 _ _ _ _ w2357 w2839 _]
          tunnel: w27 -> [_ _ w97 w246 w1060 w1471 w1781 w1853 _ _ _ _ w2356 w2837 _]
          tunnel: w26 -> [_ _ w96 w244 w1059 w1470 w1780 w1852 _ _ _ _ w2355 w2835 _]
          tunnel: w25 -> [_ _ w95 w242 w1058 w1469 w1779 w1851 _ _ _ _ w2354 w2833 _]
          tunnel: w24 -> [_ _ _ w259 w1057 w1468 _ _ _ _ _ _ _ w2853 _]
          tunnel: w23 -> [_ _ _ w257 w1056 w1466 _ _ _ _ _ _ _ w2848 _]
          tunnel: w22 -> [_ _ _ w255 w1055 w1465 _ _ _ _ _ _ _ w2846 _]
          tunnel: w21 -> [_ _ _ w253 w1054 w1464 _ _ _ _ _ _ _ w2844 _]
          tunnel: w20 -> [_ _ _ w251 w1053 w1463 _ _ _ _ _ _ _ w2842 _]
          tunnel: w19 -> [_ _ _ w249 w1052 w1462 _ _ _ _ _ _ _ w2840 _]
          tunnel: w18 -> [_ _ _ w247 w1051 w1461 _ _ _ _ _ _ _ w2838 _]
          tunnel: w17 -> [_ _ _ w245 w1050 w1460 _ _ _ _ _ _ _ w2836 _]
          tunnel: w16 -> [_ _ _ w243 w1049 w1459 _ _ _ _ _ _ _ w2834 _]
          tunnel: w15 -> [_ _ _ w241 w1048 w1458 _ _ _ _ _ _ _ w2832 _]
          frame #0 {
            w39 = FALSE
            w44 = 0.5
            # "set up cycle control"
            n33 = local read "jig cycle"() -> (w43:dbl)
            n34 = Divide(x="JIG ON TIME (S)", y=w44) -> (x/y=→"on loops":dbl)
            n35 = Divide(x="JIG OFF TIME (S)", y=w44) -> (x/y=→"off loops":dbl)
            n36 = Increment(x=w43) -> (x+1=w42:dbl)
            n37 = local write "TEMP update"(w39) -> ()
            n38 = local write "AI update"(w39) -> ()
            n39 = local write "jig cycle"(w42) -> ()
          }
          frame #1 {
            w84 = 60.0
            # "convert temperature rise minutes to cycles"
            n40 = local read "LAB05-2 (SET)"() -> (w48:T5)
            n41 = local read "LAB05-1 (SET)"() -> (w50:T5)
            n42 = local read "LAB04-2 (SET)"() -> (w52:T5)
            n43 = local read "LAB01-1 (SET)"() -> (w66:T5)
            n44 = local read "LAB02-2 (SET)"() -> (w60:T5)
            n45 = local read "LAB01-2(SET)"() -> (w64:T5)
            n46 = local read "LAB04-1 (SET)"() -> (w54:T5)
            n47 = local read "LAB03-1 (SET)"() -> (w58:T5)
            n48 = local read "LAB03-2 (SET)"() -> (w56:T5)
            n49 = local read "LAB02-1 (SET)"() -> (w62:T5)
            n50 = local read "JIG OFF TIME (S)"() -> (w89:dbl)
            n51 = local read "JIG ON TIME (S)"() -> (w90:dbl)
            n52 = Unbundle(w48) -> ("T-RISE mins"=w47:dbl)  [unwired: 4 out]
            n53 = Unbundle(w50) -> ("T-RISE mins"=w49:dbl)  [unwired: 4 out]
            n54 = Unbundle(w66) -> ("T-RISE mins"=w65:dbl)  [unwired: 4 out]
            n55 = Unbundle(w52) -> ("T-RISE mins"=w51:dbl)  [unwired: 4 out]
            n56 = Unbundle(w64) -> ("T-RISE mins"=w63:dbl)  [unwired: 4 out]
            n57 = Unbundle(w62) -> ("T-RISE mins"=w61:dbl)  [unwired: 4 out]
            n58 = Unbundle(w54) -> ("T-RISE mins"=w53:dbl)  [unwired: 4 out]
            n59 = Unbundle(w60) -> ("T-RISE mins"=w59:dbl)  [unwired: 4 out]
            n60 = Unbundle(w56) -> ("T-RISE mins"=w55:dbl)  [unwired: 4 out]
            n61 = Unbundle(w58) -> ("T-RISE mins"=w57:dbl)  [unwired: 4 out]
            n62 = Add(x=w90, y=w89) -> (x+y=w83:dbl)
            n63 = Multiply(x=w84, y=w55) -> (x*y=w79:dbl)
            n64 = Multiply(x=w84, y=w53) -> (x*y=w78:dbl)
            n65 = Multiply(x=w84, y=w51) -> (x*y=w77:dbl)
            n66 = Multiply(x=w84, y=w49) -> (x*y=w76:dbl)
            n67 = Multiply(x=w84, y=w47) -> (x*y=w75:dbl)
            n68 = Multiply(x=w84, y=w63) -> (x*y=w85:dbl)
            n69 = Multiply(x=w84, y=w57) -> (x*y=w80:dbl)
            n70 = Multiply(x=w84, y=w65) -> (x*y=w86:dbl)
            n71 = Multiply(x=w84, y=w61) -> (x*y=w82:dbl)
            n72 = Multiply(x=w84, y=w59) -> (x*y=w81:dbl)
            n73 = Divide(x=w76, y=w83) -> (x/y=w68:dbl)
            n74 = Divide(x=w77, y=w83) -> (x/y=w69:dbl)
            n75 = Divide(x=w78, y=w83) -> (x/y=w70:dbl)
            n76 = Divide(x=w75, y=w83) -> (x/y=w67:dbl)
            n77 = Divide(x=w80, y=w83) -> (x/y=w72:dbl)
            n78 = Divide(x=w86, y=w83) -> (x/y=w88:dbl)
            n79 = Divide(x=w85, y=w83) -> (x/y=w87:dbl)
            n80 = Divide(x=w82, y=w83) -> (x/y=w74:dbl)
            n81 = Divide(x=w81, y=w83) -> (x/y=w73:dbl)
            n82 = Divide(x=w79, y=w83) -> (x/y=w71:dbl)
          }
          frame #2 {
            # "control cycle loops"
            n83 = local read "JIG OFF TIME (S)"() -> (w93:dbl)
            n84 = local read "JIG ON TIME (S)"() -> (w92:dbl)
            n85 = local read "jig cycle"() -> (w106:dbl)
            n86 = local read "on loops"() -> (w108:dbl)
            n87 = local read "off loops"() -> (w107:dbl)
            n88 = Add(x=w93, y=w92) -> (x+y=w91:dbl)
            n89 = Add(x=w108, y=w107) -> (x+y=w94:dbl)
            n90 = Greater Or Equal?(x=w106, y=w94) -> (x >= y?=w105:bool)
            n91 = case shown="True" w105 {
              tunnel: w104 -> [_ w119]
              tunnel: w103 -> [_ w118]
              tunnel: w102 -> [_ w117]
              tunnel: w101 -> [_ w116]
              tunnel: w100 -> [_ w115]
              tunnel: w99 -> [_ w114]
              tunnel: w98 -> [_ w113]
              tunnel: w97 -> [_ w112]
              tunnel: w96 -> [_ w111]
              tunnel: w95 -> [_ w110]
              tunnel: w91 -> [_ w109]
              frame False {
              }
              frame True {
                # "increment cycle value and convert cycles to minutes for temp rise"
                n92 = stacked-sequence {
                  tunnel: w119 -> [w129 _ _ _ _ _ _ _ _ _]
                  tunnel: w118 -> [_ w141 _ _ _ _ _ _ _ _]
                  tunnel: w117 -> [_ _ w153 _ _ _ _ _ _ _]
                  tunnel: w116 -> [_ _ _ w165 _ _ _ _ _ _]
                  tunnel: w115 -> [_ _ _ _ w177 _ _ _ _ _]
                  tunnel: w114 -> [_ _ _ _ _ w189 _ _ _ _]
                  tunnel: w113 -> [_ _ _ _ _ _ w201 _ _ _]
                  tunnel: w112 -> [_ _ _ _ _ _ _ w213 _ _]
                  tunnel: w111 -> [_ _ _ _ _ _ _ _ w225 _]
                  tunnel: w110 -> [_ _ _ _ _ _ _ _ _ w237]
                  tunnel: w109 -> [w126 w138 w150 w162 w174 w186 w198 w210 w222 w234]
                  frame #0 {
                    # "LAB01-1"
                    n93 = local read "LAB01-1 (DISP)"() -> (w124:T4)
                    n94 = Unbundle(w124) -> ("CYCLE"=w125:dbl)  [unwired: 2 out]
                    n95 = case shown="True" w129 {
                      tunnel: w125 -> [w130 w132]
                      tunnel: [w130 w131] -> w123
                      frame False {
                      }
                      frame True {
                        n96 = Increment(x=w132) -> (x+1=w131:dbl)
                      }
                    }
                    n97 = Multiply(x=w123, y=w126) -> (x*y=w127:dbl)
                    n98 = Divide(x=w127, y=60.0) -> (x/y=w122:dbl)
                    n99 = Bundle(cluster=w124, "CYCLE"=w123, "MINS"=w122) -> (w121:T4)  [unwired: 1 in]
                    n100 = local write "LAB01-1 (DISP)"(w121) -> ()
                  }
                  frame #1 {
                    # "update cycle value"
                    # "LAB01-2"
                    n101 = local read "LAB01-2 (DISP)"() -> (w136:T4)
                    n102 = Unbundle(w136) -> ("CYCLE"=w137:dbl)  [unwired: 2 out]
                    n103 = case shown="True" w141 {
                      tunnel: w137 -> [w142 w144]
                      tunnel: [w142 w143] -> w134
                      frame False {
                      }
                      frame True {
                        n104 = Increment(x=w144) -> (x+1=w143:dbl)
                      }
                    }
                    n105 = Multiply(x=w134, y=w138) -> (x*y=w139:dbl)
                    n106 = Divide(x=w139, y=60.0) -> (x/y=w133:dbl)
                    n107 = Bundle(cluster=w136, "CYCLE"=w134, "MINS"=w133) -> (w135:T4)  [unwired: 1 in]
                    n108 = local write "LAB01-2 (DISP)"(w135) -> ()
                  }
                  frame #2 {
                    # "update cycle value"
                    # "LAB02-1"
                    n109 = local read "LAB02-1 (DISP)"() -> (w148:T4)
                    n110 = Unbundle(w148) -> ("CYCLE"=w149:dbl)  [unwired: 2 out]
                    n111 = case shown="True" w153 {
                      tunnel: [w154 w156] -> w146
                      tunnel: w149 -> [w154 w155]
                      frame False {
                      }
                      frame True {
                        n112 = Increment(x=w155) -> (x+1=w156:dbl)
                      }
                    }
                    n113 = Multiply(x=w146, y=w150) -> (x*y=w151:dbl)
                    n114 = Divide(x=w151, y=60.0) -> (x/y=w145:dbl)
                    n115 = Bundle(cluster=w148, "CYCLE"=w146, "MINS"=w145) -> (w147:T4)  [unwired: 1 in]
                    n116 = local write "LAB02-1 (DISP)"(w147) -> ()
                  }
                  frame #3 {
                    # "update cycle value"
                    # "LAB02-2"
                    n117 = local read "LAB02-2 (DISP)"() -> (w160:T4)
                    n118 = Unbundle(w160) -> ("CYCLE"=w161:dbl)  [unwired: 2 out]
                    n119 = case shown="True" w165 {
                      tunnel: [w166 w168] -> w159
                      tunnel: w161 -> [w166 w167]
                      frame False {
                      }
                      frame True {
                        n120 = Increment(x=w167) -> (x+1=w168:dbl)
                      }
                    }
                    n121 = Multiply(x=w159, y=w162) -> (x*y=w163:dbl)
                    n122 = Divide(x=w163, y=60.0) -> (x/y=w158:dbl)
                    n123 = Bundle(cluster=w160, "CYCLE"=w159, "MINS"=w158) -> (w157:T4)  [unwired: 1 in]
                    n124 = local write "LAB02-2 (DISP)"(w157) -> ()
                  }
                  frame #4 {
                    # "update cycle value"
                    # "LAB03-1"
                    n125 = local read "LAB03-1 (DISP)"() -> (w172:T4)
                    n126 = Unbundle(w172) -> ("CYCLE"=w173:dbl)  [unwired: 2 out]
                    n127 = case shown="True" w177 {
                      tunnel: [w178 w180] -> w169
                      tunnel: w173 -> [w178 w179]
                      frame False {
                      }
                      frame True {
                        n128 = Increment(x=w179) -> (x+1=w180:dbl)
                      }
                    }
                    n129 = Multiply(x=w169, y=w174) -> (x*y=w175:dbl)
                    n130 = Divide(x=w175, y=60.0) -> (x/y=w170:dbl)
                    n131 = Bundle(cluster=w172, "CYCLE"=w169, "MINS"=w170) -> (w171:T4)  [unwired: 1 in]
                    n132 = local write "LAB03-1 (DISP)"(w171) -> ()
                  }
                  frame #5 {
                    # "update cycle value"
                    # "LAB03-2"
                    n133 = local read "LAB03-2 (DISP)"() -> (w184:T4)
                    n134 = Unbundle(w184) -> ("CYCLE"=w185:dbl)  [unwired: 2 out]
                    n135 = case shown="False" w189 {
                      tunnel: [w190 w192] -> w183
                      tunnel: w185 -> [w190 w191]
                      frame False {
                      }
                      frame True {
                        n136 = Increment(x=w191) -> (x+1=w192:dbl)
                      }
                    }
                    n137 = Multiply(x=w183, y=w186) -> (x*y=w187:dbl)
                    n138 = Divide(x=w187, y=60.0) -> (x/y=w182:dbl)
                    n139 = Bundle(cluster=w184, "CYCLE"=w183, "MINS"=w182) -> (w181:T4)  [unwired: 1 in]
                    n140 = local write "LAB03-2 (DISP)"(w181) -> ()
                  }
                  frame #6 {
                    # "update cycle value"
                    # "LAB04-1"
                    n141 = local read "LAB04-1 (DISP)"() -> (w196:T4)
                    n142 = Unbundle(w196) -> ("CYCLE"=w197:dbl)  [unwired: 2 out]
                    n143 = case shown="True" w201 {
                      tunnel: [w202 w204] -> w194
                      tunnel: w197 -> [w202 w203]
                      frame False {
                      }
                      frame True {
                        n144 = Increment(x=w203) -> (x+1=w204:dbl)
                      }
                    }
                    n145 = Multiply(x=w194, y=w198) -> (x*y=w199:dbl)
                    n146 = Divide(x=w199, y=60.0) -> (x/y=w193:dbl)
                    n147 = Bundle(cluster=w196, "CYCLE"=w194, "MINS"=w193) -> (w195:T4)  [unwired: 1 in]
                    n148 = local write "LAB04-1 (DISP)"(w195) -> ()
                  }
                  frame #7 {
                    # "update cycle value"
                    # "LAB04-2"
                    n149 = local read "LAB04-2 (DISP)"() -> (w208:T4)
                    n150 = Unbundle(w208) -> ("CYCLE"=w209:dbl)  [unwired: 2 out]
                    n151 = case shown="True" w213 {
                      tunnel: [w214 w216] -> w206
                      tunnel: w209 -> [w214 w215]
                      frame False {
                      }
                      frame True {
                        n152 = Increment(x=w215) -> (x+1=w216:dbl)
                      }
                    }
                    n153 = Multiply(x=w206, y=w210) -> (x*y=w212:dbl)
                    n154 = Divide(x=w212, y=60.0) -> (x/y=w205:dbl)
                    n155 = Bundle(cluster=w208, "CYCLE"=w206, "MINS"=w205) -> (w207:T4)  [unwired: 1 in]
                    n156 = local write "LAB04-2 (DISP)"(w207) -> ()
                  }
                  frame #8 {
                    # "update cycle value"
                    # "LAB05-1"
                    n157 = local read "LAB05-1 (DISP)"() -> (w220:T4)
                    n158 = Unbundle(w220) -> ("CYCLE"=w221:dbl)  [unwired: 2 out]
                    n159 = case shown="True" w225 {
                      tunnel: [w226 w228] -> w218
                      tunnel: w221 -> [w226 w227]
                      frame False {
                      }
                      frame True {
                        n160 = Increment(x=w227) -> (x+1=w228:dbl)
                      }
                    }
                    n161 = Multiply(x=w218, y=w222) -> (x*y=w223:dbl)
                    n162 = Divide(x=w223, y=60.0) -> (x/y=w217:dbl)
                    n163 = Bundle(cluster=w220, "CYCLE"=w218, "MINS"=w217) -> (w219:T4)  [unwired: 1 in]
                    n164 = local write "LAB05-1 (DISP)"(w219) -> ()
                  }
                  frame #9 {
                    # "update cycle value"
                    # "LAB05-2"
                    n165 = local read "LAB05-2 (DISP)"() -> (w233:T4)
                    n166 = Unbundle(w233) -> ("CYCLE"=w232:dbl)  [unwired: 2 out]
                    n167 = case shown="True" w237 {
                      tunnel: [w238 w240] -> w231
                      tunnel: w232 -> [w238 w239]
                      frame False {
                      }
                      frame True {
                        n168 = Increment(x=w239) -> (x+1=w240:dbl)
                      }
                    }
                    n169 = Multiply(x=w231, y=w234) -> (x*y=w235:dbl)
                    n170 = Divide(x=w235, y=60.0) -> (x/y=w230:dbl)
                    n171 = Bundle(cluster=w233, "CYCLE"=w231, "MINS"=w230) -> (w229:T4)  [unwired: 1 in]
                    n172 = local write "LAB05-2 (DISP)"(w229) -> ()
                  }
                }
                n173 = local write "jig cycle"(0) -> ()
              }
            }
          }
          frame #3 {
            # "START & STOP test RUN switch change, start test if true and stop test if false"
            n174 = Get Date/Time In Seconds() -> (seconds since 1Jan1904=w263:timestamp)
            n175 = Format Date/Time String(time format string (%c)="%Y%m%d", seconds (now)=w263) -> (date/time string=w264:string)  [unwired: 1 in]
            n176 = Format Date/Time String(time format string (%c)="%H%M", seconds (now)=w263) -> (date/time string=w261:string)  [unwired: 1 in]
            n177 = event shown="[1] \"LAB01-1RUN\": Value Change" {
              selector: _ -> [_ _ _ _ _ _ _ _ _ _ _]
              dyn-events: _ -> [_ _ _ _ _ _ _ _ _ _ _]
              timeout: 10 -> [_ _ _ _ _ _ _ _ _ _ _]
              tunnel: "c:\\crabtree\\Test Data\\" -> [_ w272 w350 w428 w506 w584 w662 w740 w818 w896 w974]
              tunnel: w264 -> [_ w271 w349 w427 w505 w583 w661 w739 w817 w895 w973]
              tunnel: w261 -> [_ w269 w348 w426 w504 w582 w660 w738 w816 w894 w972]
              tunnel: w259 -> [_ w270 _ _ _ _ _ _ _ _ _]
              tunnel: w260 -> [_ _ _ _ _ _ _ _ _ _ _]
              tunnel: w258 -> [_ _ _ _ _ _ _ _ _ _ _]
              tunnel: w257 -> [_ _ w347 _ _ _ _ _ _ _ _]
              tunnel: w256 -> [_ _ _ _ _ _ _ _ _ _ _]
              tunnel: w255 -> [_ _ _ w425 _ _ _ _ _ _ _]
              tunnel: w254 -> [_ _ _ _ _ _ _ _ _ _ _]
              tunnel: w253 -> [_ _ _ _ w503 _ _ _ _ _ _]
              tunnel: w252 -> [_ _ _ _ _ _ _ _ _ _ _]
              tunnel: w251 -> [_ _ _ _ _ w581 _ _ _ _ _]
              tunnel: w250 -> [_ _ _ _ _ _ _ _ _ _ _]
              tunnel: w249 -> [_ _ _ _ _ _ w659 _ _ _ _]
              tunnel: w248 -> [_ _ _ _ _ _ _ _ _ _ _]
              tunnel: w247 -> [_ _ _ _ _ _ _ w737 _ _ _]
              tunnel: w246 -> [_ _ _ _ _ _ _ _ _ _ _]
              tunnel: w245 -> [_ _ _ _ _ _ _ _ w815 _ _]
              tunnel: w244 -> [_ _ _ _ _ _ _ _ _ _ _]
              tunnel: w243 -> [_ _ _ _ _ _ _ _ _ w893 _]
              tunnel: w242 -> [_ _ _ _ _ _ _ _ _ _ _]
              tunnel: w241 -> [_ _ _ _ _ _ _ _ _ _ w971]
              event Timeout {
                n178 = event-data() -> ()  [unwired: 1 in, 3 out]
              }
              event "LAB01-1RUN": Value Change {
                n179 = event-data() -> ("NewVal"=w268:bool)  [unwired: 1 in, 5 out]
                n180 = case shown="True" w268 {
                  tunnel: w272 -> [_ w294]
                  tunnel: w271 -> [_ w293]
                  tunnel: w270 -> [w273 w292]
                  tunnel: w269 -> [_ w291]
                  frame False {
                    # "stop test"
                    n181 = stacked-sequence {
                      tunnel: w273 -> [w279 _]
                      frame #0 {
                        n182 = local read "LAB01-1 (DISP)"() -> (w278:T4)
                        n183 = Unbundle(w278) -> ("CYCLE"=w276:dbl, "MINS"=w277:dbl)  [unwired: 1 out]
                        n184 = case shown="\"CYCLE TEST\"" w279 {
                          tunnel: w277 -> [_ _ w286]
                          tunnel: w276 -> [w284 w285 _]
                          tunnel: [w284 w285 w286] -> w275
                          frame "TEST SET UP", Default {
                          }
                          frame "CYCLE TEST" {
                          }
                          frame "T-RISE TEST" {
                          }
                        }
                        n185 = local read "LAB01-1 (TDMS)"() -> (w283:refnum<k34>)
                        n186 = Build Array("STOPPED") -> (w280:string[])
                        n187 = Build Array(w275) -> (w274:dbl[])
                        n188 = TDMS Write(0:w283, 5:"TEST RESULT", 7:w280, 9:w274) -> ()  [unwired: 2 in, 4 out]
                      }
                      frame #1 {
                        n189 = local read "LAB01-1 (DISP)"() -> (w290:T4)
                        n190 = Bundle(cluster=w290, "STATUS"="STOP") -> (w288:T4)  [unwired: 2 in]
                        n191 = local write "LAB01-1 (RESULT)"(FALSE) -> ()
                        n192 = local write "LAB01-1 (DISP)"(w288) -> ()
                      }
                    }
                  }
                  frame True {
                    # "start new test and create test file"
                    n193 = stacked-sequence {
                      seq-local: [w300 _ _ _ _] -> [_ w319 _ _ _]
                      tunnel: w294 -> [w309 _ _ _ _]
                      tunnel: w293 -> [w307 _ _ _ _]
                      tunnel: w292 -> [w306 _ _ _ _]
                      tunnel: w291 -> [w297 _ _ _ _]
                      frame #0 {
                        n194 = local read "LAB01-1 (SET)"() -> (w299:T5)
                        n195 = case shown="\"TEST SET UP\", Default" w306 {
                          tunnel: ["TEST SET UP-" "CYCLE TEST-" "T-RISE TEST-"] -> w302
                          frame "TEST SET UP", Default {
                          }
                          frame "CYCLE TEST" {
                          }
                          frame "T-RISE TEST" {
                          }
                        }
                        n196 = Unbundle(w299) -> ("DESCRIPTION"=w298:string)  [unwired: 4 out]
                        n197 = Concatenate Strings(w309, "LAB01-1\\", w307, "\\") -> (w303:string)
                        n198 = String To Path(string=w303) -> (path=w305:path)
                        n199 = Concatenate Strings(w303, w302, w298, "-", w297, ".tdms") -> (w300:string)
                        n200 = Create Folder(path (use dialog)=w305) -> (error out=w304:errorcluster)  [unwired: 2 in, 2 out]
                        n201 = call <vilib>:"Clear Errors.vi"("error in (no error)"=w304) -> ()  [unwired: 6 in, 1 out]
                      }
                      frame #1 {
                        n202 = String To Path(string=w319) -> (path=w313:path)
                        n203 = TDMS Open(5:FALSE, 6:FALSE, 10:T14."create or replace" ("operation (0:open)"), 11:w313) -> (0:w315:errorcluster, 3:→"LAB01-1 (TDMS)":refnum<k34>)  [unwired: 3 in]
                        n204 = local write "data file error"(w315) -> ()
                      }
                      frame #2 {
                        n205 = local read "LAB01-1 (SET)"() -> (w325:T5)
                        n206 = local read "LAB01-1 (TDMS)"() -> (w336:refnum<k34>)
                        n207 = Build Array("Testers Name", "Description", "Set Test Cycles", "T-Rise minutes", "T-Rise Deg C") -> (w326:string[])
                        n208 = Unbundle(w325) -> ("NAME"=w324:string, "DESCRIPTION"=w323:string, "CYCLES"=w322:dbl, "T-RISE mins"=w321:dbl, "T-RISE deg C"=w320:dbl)
                        n209 = Number To Decimal String(number=w322) -> (decimal integer string=w335:string)  [unwired: 1 in]
                        n210 = Number To Decimal String(number=w321) -> (decimal integer string=w334:string)  [unwired: 1 in]
                        n211 = Number To Decimal String(number=w320) -> (decimal integer string=w333:string)  [unwired: 1 in]
                        n212 = Build Array(w324, w323, w335, w334, w333) -> (w332:string[])
                        n213 = TDMS Set Properties(5:w332, 7:w326, 11:w336) -> ()  [unwired: 3 in, 4 out]
                      }
                      frame #3 {
                        w337 = 0.0
                        n214 = local read "LAB01-1 (DISP)"() -> (w340:T4)
                        n215 = Bundle(cluster=w340, "CYCLE"=w337, "MINS"=w337, "STATUS"="RUN") -> (w339:T4)
                        n216 = local write "LAB01-1 (DISP)"(w339) -> ()
                      }
                      frame #4 {
                        n217 = local read "LAB01-1 (SIG)"() -> (w343:T2)
                        n218 = local read "LAB01-1 (TEMP START)"() -> (w345:cluster{"TL":dbl, "TN":dbl})
                        n219 = Unbundle(w343) -> ("Tmp Live"=w342:dbl, "Tmp Neut"=w341:dbl)  [unwired: 3 out]
                        n220 = Bundle(cluster=w345, "TL"=w342, "TN"=w341) -> (w344:cluster{"TL":dbl, "TN":dbl})
                        n221 = local write "LAB01-1 (TEMP START)"(w344) -> ()
                      }
                    }
                  }
                }
              }
              event "LAB01-2 RUN": Value Change {
                n222 = event-data() -> ("NewVal"=w346:bool)  [unwired: 1 in, 5 out]
                n223 = case shown="True" w346 {
                  tunnel: w350 -> [_ w372]
                  tunnel: w349 -> [_ w371]
                  tunnel: w347 -> [w351 w370]
                  tunnel: w348 -> [_ w369]
                  frame False {
                    # "stop test"
                    n224 = stacked-sequence {
                      tunnel: w351 -> [w357 _]
                      frame #0 {
                        n225 = local read "LAB01-2 (DISP)"() -> (w356:T4)
                        n226 = Unbundle(w356) -> ("CYCLE"=w354:dbl, "MINS"=w355:dbl)  [unwired: 1 out]
                        n227 = case shown="\"CYCLE TEST\"" w357 {
                          tunnel: w355 -> [_ _ w364]
                          tunnel: w354 -> [w362 w363 _]
                          tunnel: [w362 w363 w364] -> w353
                          frame "TEST SET UP", Default {
                          }
                          frame "CYCLE TEST" {
                          }
                          frame "T-RISE TEST" {
                          }
                        }
                        n228 = local read "LAB01-2 (TDMS)"() -> (w361:refnum<k34>)
                        n229 = Build Array("STOPPED") -> (w358:string[])
                        n230 = Build Array(w353) -> (w352:dbl[])
                        n231 = TDMS Write(0:w361, 5:"TEST RESULT", 7:w358, 9:w352) -> ()  [unwired: 2 in, 4 out]
                      }
                      frame #1 {
                        n232 = local read "LAB01-2 (DISP)"() -> (w368:T4)
                        n233 = Bundle(cluster=w368, "STATUS"="STOP") -> (w366:T4)  [unwired: 2 in]
                        n234 = local write "LAB01-2 (RESULT)"(FALSE) -> ()
                        n235 = local write "LAB01-2 (DISP)"(w366) -> ()
                      }
                    }
                  }
                  frame True {
                    # "start new test and create test file"
                    n236 = stacked-sequence {
                      seq-local: [w378 _ _ _ _] -> [_ w397 _ _ _]
                      tunnel: w372 -> [w387 _ _ _ _]
                      tunnel: w371 -> [w385 _ _ _ _]
                      tunnel: w370 -> [w384 _ _ _ _]
                      tunnel: w369 -> [w375 _ _ _ _]
                      frame #0 {
                        n237 = local read "LAB01-2(SET)"() -> (w377:T5)
                        n238 = case shown="\"TEST SET UP\", Default" w384 {
                          tunnel: ["TEST SET UP-" "CYCLE TEST-" "T-RISE TEST-"] -> w380
                          frame "TEST SET UP", Default {
                          }
                          frame "CYCLE TEST" {
                          }
                          frame "T-RISE TEST" {
                          }
                        }
                        n239 = Unbundle(w377) -> ("DESCRIPTION"=w376:string)  [unwired: 4 out]
                        n240 = Concatenate Strings(w387, "LAB01-2\\", w385, "\\") -> (w381:string)
                        n241 = String To Path(string=w381) -> (path=w383:path)
                        n242 = Concatenate Strings(w381, w380, w376, "-", w375, ".tdms") -> (w378:string)
                        n243 = Create Folder(path (use dialog)=w383) -> (error out=w382:errorcluster)  [unwired: 2 in, 2 out]
                        n244 = call <vilib>:"Clear Errors.vi"("error in (no error)"=w382) -> ()  [unwired: 6 in, 1 out]
                      }
                      frame #1 {
                        n245 = String To Path(string=w397) -> (path=w391:path)
                        n246 = TDMS Open(5:FALSE, 6:FALSE, 10:T14."create or replace" ("operation (0:open)"), 11:w391) -> (0:w393:errorcluster, 3:→"LAB01-2 (TDMS)":refnum<k34>)  [unwired: 3 in]
                        n247 = local write "data file error"(w393) -> ()
                      }
                      frame #2 {
                        n248 = local read "LAB01-2(SET)"() -> (w403:T5)
                        n249 = local read "LAB01-2 (TDMS)"() -> (w414:refnum<k34>)
                        n250 = Build Array("Testers Name", "Description", "Set Test Cycles", "T-Rise minutes", "T-Rise Deg C") -> (w404:string[])
                        n251 = Unbundle(w403) -> ("NAME"=w402:string, "DESCRIPTION"=w401:string, "CYCLES"=w400:dbl, "T-RISE mins"=w399:dbl, "T-RISE deg C"=w398:dbl)
                        n252 = Number To Decimal String(number=w400) -> (decimal integer string=w413:string)  [unwired: 1 in]
                        n253 = Number To Decimal String(number=w399) -> (decimal integer string=w412:string)  [unwired: 1 in]
                        n254 = Number To Decimal String(number=w398) -> (decimal integer string=w411:string)  [unwired: 1 in]
                        n255 = Build Array(w402, w401, w413, w412, w411) -> (w410:string[])
                        n256 = TDMS Set Properties(5:w410, 7:w404, 11:w414) -> ()  [unwired: 3 in, 4 out]
                      }
                      frame #3 {
                        w416 = 0.0
                        n257 = local read "LAB01-2 (DISP)"() -> (w418:T4)
                        n258 = Bundle(cluster=w418, "CYCLE"=w416, "MINS"=w416, "STATUS"="RUN") -> (w417:T4)
                        n259 = local write "LAB01-2 (DISP)"(w417) -> ()
                      }
                      frame #4 {
                        n260 = local read "LAB01-2 (SIG)"() -> (w421:T2)
                        n261 = local read "LAB01-2 (TEMP START)"() -> (w423:cluster{"TL":dbl, "TN":dbl})
                        n262 = Unbundle(w421) -> ("Tmp Live"=w420:dbl, "Tmp Neut"=w419:dbl)  [unwired: 3 out]
                        n263 = Bundle(cluster=w423, "TL"=w420, "TN"=w419) -> (w422:cluster{"TL":dbl, "TN":dbl})
                        n264 = local write "LAB01-2 (TEMP START)"(w422) -> ()
                      }
                    }
                  }
                }
              }
              event "LAB02-1 RUN": Value Change {
                n265 = event-data() -> ("NewVal"=w424:bool)  [unwired: 1 in, 5 out]
                n266 = case shown="True" w424 {
                  tunnel: w428 -> [_ w450]
                  tunnel: w427 -> [_ w449]
                  tunnel: w425 -> [w429 w448]
                  tunnel: w426 -> [_ w447]
                  frame False {
                    # "stop test"
                    n267 = stacked-sequence {
                      tunnel: w429 -> [w435 _]
                      frame #0 {
                        n268 = local read "LAB02-1 (DISP)"() -> (w434:T4)
                        n269 = Unbundle(w434) -> ("CYCLE"=w432:dbl, "MINS"=w433:dbl)  [unwired: 1 out]
                        n270 = case shown="\"CYCLE TEST\"" w435 {
                          tunnel: w433 -> [_ _ w442]
                          tunnel: w432 -> [w440 w441 _]
                          tunnel: [w440 w441 w442] -> w431
                          frame "TEST SET UP", Default {
                          }
                          frame "CYCLE TEST" {
                          }
                          frame "T-RISE TEST" {
                          }
                        }
                        n271 = local read "LAB02-1 (TDMS)"() -> (w439:refnum<k34>)
                        n272 = Build Array("STOPPED") -> (w436:string[])
                        n273 = Build Array(w431) -> (w430:dbl[])
                        n274 = TDMS Write(0:w439, 5:"TEST RESULT", 7:w436, 9:w430) -> ()  [unwired: 2 in, 4 out]
                      }
                      frame #1 {
                        n275 = local read "LAB02-1 (DISP)"() -> (w446:T4)
                        n276 = Bundle(cluster=w446, "STATUS"="STOPPED") -> (w444:T4)  [unwired: 2 in]
                        n277 = local write "LAB02-1 (RESULT)"(FALSE) -> ()
                        n278 = local write "LAB02-1 (DISP)"(w444) -> ()
                      }
                    }
                  }
                  frame True {
                    # "start new test and create test file"
                    n279 = stacked-sequence {
                      seq-local: [w456 _ _ _ _] -> [_ w475 _ _ _]
                      tunnel: w450 -> [w465 _ _ _ _]
                      tunnel: w449 -> [w463 _ _ _ _]
                      tunnel: w448 -> [w462 _ _ _ _]
                      tunnel: w447 -> [w453 _ _ _ _]
                      frame #0 {
                        n280 = local read "LAB02-1 (SET)"() -> (w455:T5)
                        n281 = case shown="\"TEST SET UP\", Default" w462 {
                          tunnel: ["TEST SET UP-" "CYCLE TEST-" "T-RISE TEST-"] -> w458
                          frame "TEST SET UP", Default {
                          }
                          frame "CYCLE TEST" {
                          }
                          frame "T-RISE TEST" {
                          }
                        }
                        n282 = Unbundle(w455) -> ("DESCRIPTION"=w454:string)  [unwired: 4 out]
                        n283 = Concatenate Strings(w465, "LAB02-1\\", w463, "\\") -> (w459:string)
                        n284 = String To Path(string=w459) -> (path=w461:path)
                        n285 = Concatenate Strings(w459, w458, w454, "-", w453, ".tdms") -> (w456:string)
                        n286 = Create Folder(path (use dialog)=w461) -> (error out=w460:errorcluster)  [unwired: 2 in, 2 out]
                        n287 = call <vilib>:"Clear Errors.vi"("error in (no error)"=w460) -> ()  [unwired: 6 in, 1 out]
                      }
                      frame #1 {
                        n288 = String To Path(string=w475) -> (path=w469:path)
                        n289 = TDMS Open(5:FALSE, 6:FALSE, 10:T14."create or replace" ("operation (0:open)"), 11:w469) -> (0:w471:errorcluster, 3:→"LAB02-1 (TDMS)":refnum<k34>)  [unwired: 3 in]
                        n290 = local write "data file error"(w471) -> ()
                      }
                      frame #2 {
                        n291 = local read "LAB02-1 (SET)"() -> (w481:T5)
                        n292 = local read "LAB02-1 (TDMS)"() -> (w492:refnum<k34>)
                        n293 = Build Array("Testers Name", "Description", "Set Test Cycles", "T-Rise minutes", "T-Rise Deg C") -> (w482:string[])
                        n294 = Unbundle(w481) -> ("NAME"=w480:string, "DESCRIPTION"=w479:string, "CYCLES"=w478:dbl, "T-RISE mins"=w477:dbl, "T-RISE deg C"=w476:dbl)
                        n295 = Number To Decimal String(number=w478) -> (decimal integer string=w491:string)  [unwired: 1 in]
                        n296 = Number To Decimal String(number=w477) -> (decimal integer string=w490:string)  [unwired: 1 in]
                        n297 = Number To Decimal String(number=w476) -> (decimal integer string=w489:string)  [unwired: 1 in]
                        n298 = Build Array(w480, w479, w491, w490, w489) -> (w488:string[])
                        n299 = TDMS Set Properties(5:w488, 7:w482, 11:w492) -> ()  [unwired: 3 in, 4 out]
                      }
                      frame #3 {
                        w494 = 0.0
                        n300 = local read "LAB02-1 (DISP)"() -> (w496:T4)
                        n301 = Bundle(cluster=w496, "CYCLE"=w494, "MINS"=w494, "STATUS"="RUN") -> (w495:T4)
                        n302 = local write "LAB02-1 (DISP)"(w495) -> ()
                      }
                      frame #4 {
                        n303 = local read "LAB02-1 (SIG)"() -> (w499:T2)
                        n304 = local read "LAB02-1 (TEMP START)"() -> (w501:cluster{"TL":dbl, "TN":dbl})
                        n305 = Unbundle(w499) -> ("Tmp Live"=w498:dbl, "Tmp Neut"=w497:dbl)  [unwired: 3 out]
                        n306 = Bundle(cluster=w501, "TL"=w498, "TN"=w497) -> (w500:cluster{"TL":dbl, "TN":dbl})
                        n307 = local write "LAB02-1 (TEMP START)"(w500) -> ()
                      }
                    }
                  }
                }
              }
              event "LAB02-2 RUN": Value Change {
                n308 = event-data() -> ("NewVal"=w502:bool)  [unwired: 1 in, 5 out]
                n309 = case shown="True" w502 {
                  tunnel: w506 -> [_ w528]
                  tunnel: w505 -> [_ w527]
                  tunnel: w503 -> [w507 w526]
                  tunnel: w504 -> [_ w525]
                  frame False {
                    # "stop test"
                    n310 = stacked-sequence {
                      tunnel: w507 -> [w513 _]
                      frame #0 {
                        n311 = local read "LAB02-2 (DISP)"() -> (w512:T4)
                        n312 = Unbundle(w512) -> ("CYCLE"=w510:dbl, "MINS"=w511:dbl)  [unwired: 1 out]
                        n313 = case shown="\"CYCLE TEST\"" w513 {
                          tunnel: w511 -> [_ _ w520]
                          tunnel: w510 -> [w518 w519 _]
                          tunnel: [w518 w519 w520] -> w509
                          frame "TEST SET UP", Default {
                          }
                          frame "CYCLE TEST" {
                          }
                          frame "T-RISE TEST" {
                          }
                        }
                        n314 = local read "LAB02-2 (TDMS)"() -> (w517:refnum<k34>)
                        n315 = Build Array("STOPPED") -> (w514:string[])
                        n316 = Build Array(w509) -> (w508:dbl[])
                        n317 = TDMS Write(0:w517, 5:"TEST RESULT", 7:w514, 9:w508) -> ()  [unwired: 2 in, 4 out]
                      }
                      frame #1 {
                        n318 = local read "LAB02-2 (DISP)"() -> (w524:T4)
                        n319 = Bundle(cluster=w524, "STATUS"="STOP") -> (w522:T4)  [unwired: 2 in]
                        n320 = local write "LAB02-2 (RESULT)"(FALSE) -> ()
                        n321 = local write "LAB02-2 (DISP)"(w522) -> ()
                      }
                    }
                  }
                  frame True {
                    # "start new test and create test file"
                    n322 = stacked-sequence {
                      seq-local: [w534 _ _ _ _] -> [_ w553 _ _ _]
                      tunnel: w528 -> [w543 _ _ _ _]
                      tunnel: w527 -> [w541 _ _ _ _]
                      tunnel: w526 -> [w540 _ _ _ _]
                      tunnel: w525 -> [w531 _ _ _ _]
                      frame #0 {
                        n323 = local read "LAB02-2 (SET)"() -> (w533:T5)
                        n324 = case shown="\"TEST SET UP\", Default" w540 {
                          tunnel: ["TEST SET UP-" "CYCLE TEST-" "T-RISE TEST-"] -> w536
                          frame "TEST SET UP", Default {
                          }
                          frame "CYCLE TEST" {
                          }
                          frame "T-RISE TEST" {
                          }
                        }
                        n325 = Unbundle(w533) -> ("DESCRIPTION"=w532:string)  [unwired: 4 out]
                        n326 = Concatenate Strings(w543, "LAB02-2\\", w541, "\\") -> (w537:string)
                        n327 = String To Path(string=w537) -> (path=w539:path)
                        n328 = Concatenate Strings(w537, w536, w532, "-", w531, ".tdms") -> (w534:string)
                        n329 = Create Folder(path (use dialog)=w539) -> (error out=w538:errorcluster)  [unwired: 2 in, 2 out]
                        n330 = call <vilib>:"Clear Errors.vi"("error in (no error)"=w538) -> ()  [unwired: 6 in, 1 out]
                      }
                      frame #1 {
                        n331 = String To Path(string=w553) -> (path=w547:path)
                        n332 = TDMS Open(5:FALSE, 6:FALSE, 10:T14."create or replace" ("operation (0:open)"), 11:w547) -> (0:w549:errorcluster, 3:→"LAB02-2 (TDMS)":refnum<k34>)  [unwired: 3 in]
                        n333 = local write "data file error"(w549) -> ()
                      }
                      frame #2 {
                        n334 = local read "LAB02-2 (SET)"() -> (w559:T5)
                        n335 = local read "LAB02-2 (TDMS)"() -> (w570:refnum<k34>)
                        n336 = Build Array("Testers Name", "Description", "Set Test Cycles", "T-Rise minutes", "T-Rise Deg C") -> (w560:string[])
                        n337 = Unbundle(w559) -> ("NAME"=w558:string, "DESCRIPTION"=w557:string, "CYCLES"=w556:dbl, "T-RISE mins"=w555:dbl, "T-RISE deg C"=w554:dbl)
                        n338 = Number To Decimal String(number=w556) -> (decimal integer string=w569:string)  [unwired: 1 in]
                        n339 = Number To Decimal String(number=w555) -> (decimal integer string=w568:string)  [unwired: 1 in]
                        n340 = Number To Decimal String(number=w554) -> (decimal integer string=w567:string)  [unwired: 1 in]
                        n341 = Build Array(w558, w557, w569, w568, w567) -> (w566:string[])
                        n342 = TDMS Set Properties(5:w566, 7:w560, 11:w570) -> ()  [unwired: 3 in, 4 out]
                      }
                      frame #3 {
                        w572 = 0.0
                        n343 = local read "LAB02-2 (DISP)"() -> (w574:T4)
                        n344 = Bundle(cluster=w574, "CYCLE"=w572, "MINS"=w572, "STATUS"="RUN") -> (w573:T4)
                        n345 = local write "LAB02-2 (DISP)"(w573) -> ()
                      }
                      frame #4 {
                        n346 = local read "LAB02-2 (SIG)"() -> (w577:T2)
                        n347 = local read "LAB02-2 (TEMP START)"() -> (w579:cluster{"TL":dbl, "TN":dbl})
                        n348 = Unbundle(w577) -> ("Tmp Live"=w576:dbl, "Tmp Neut"=w575:dbl)  [unwired: 3 out]
                        n349 = Bundle(cluster=w579, "TL"=w576, "TN"=w575) -> (w578:cluster{"TL":dbl, "TN":dbl})
                        n350 = local write "LAB02-2 (TEMP START)"(w578) -> ()
                      }
                    }
                  }
                }
              }
              event "LAB03-1 RUN": Value Change {
                n351 = event-data() -> ("NewVal"=w580:bool)  [unwired: 1 in, 5 out]
                n352 = case shown="True" w580 {
                  tunnel: w584 -> [_ w606]
                  tunnel: w583 -> [_ w605]
                  tunnel: w581 -> [w585 w604]
                  tunnel: w582 -> [_ w603]
                  frame False {
                    # "stop test"
                    n353 = stacked-sequence {
                      tunnel: w585 -> [w591 _]
                      frame #0 {
                        n354 = local read "LAB03-1 (DISP)"() -> (w590:T4)
                        n355 = Unbundle(w590) -> ("CYCLE"=w588:dbl, "MINS"=w589:dbl)  [unwired: 1 out]
                        n356 = case shown="\"CYCLE TEST\"" w591 {
                          tunnel: w589 -> [_ _ w598]
                          tunnel: w588 -> [w596 w597 _]
                          tunnel: [w596 w597 w598] -> w587
                          frame "TEST SET UP", Default {
                          }
                          frame "CYCLE TEST" {
                          }
                          frame "T-RISE TEST" {
                          }
                        }
                        n357 = local read "LAB03-1 (TDMS)"() -> (w595:refnum<k34>)
                        n358 = Build Array("STOPPED") -> (w592:string[])
                        n359 = Build Array(w587) -> (w586:dbl[])
                        n360 = TDMS Write(0:w595, 5:"TEST RESULT", 7:w592, 9:w586) -> ()  [unwired: 2 in, 4 out]
                      }
                      frame #1 {
                        n361 = local read "LAB03-1 (DISP)"() -> (w602:T4)
                        n362 = Bundle(cluster=w602, "STATUS"="STOP") -> (w600:T4)  [unwired: 2 in]
                        n363 = local write "LAB03-1 (RESULT)"(FALSE) -> ()
                        n364 = local write "LAB03-1 (DISP)"(w600) -> ()
                      }
                    }
                  }
                  frame True {
                    # "start new test and create test file"
                    n365 = stacked-sequence {
                      seq-local: [w612 _ _ _ _] -> [_ w631 _ _ _]
                      tunnel: w606 -> [w621 _ _ _ _]
                      tunnel: w605 -> [w619 _ _ _ _]
                      tunnel: w604 -> [w618 _ _ _ _]
                      tunnel: w603 -> [w609 _ _ _ _]
                      frame #0 {
                        n366 = local read "LAB03-1 (SET)"() -> (w611:T5)
                        n367 = case shown="\"TEST SET UP\", Default" w618 {
                          tunnel: ["TEST SET UP-" "CYCLE TEST-" "T-RISE TEST-"] -> w614
                          frame "TEST SET UP", Default {
                          }
                          frame "CYCLE TEST" {
                          }
                          frame "T-RISE TEST" {
                          }
                        }
                        n368 = Unbundle(w611) -> ("DESCRIPTION"=w610:string)  [unwired: 4 out]
                        n369 = Concatenate Strings(w621, "LAB03-1\\", w619, "\\") -> (w615:string)
                        n370 = String To Path(string=w615) -> (path=w617:path)
                        n371 = Concatenate Strings(w615, w614, w610, "-", w609, ".tdms") -> (w612:string)
                        n372 = Create Folder(path (use dialog)=w617) -> (error out=w616:errorcluster)  [unwired: 2 in, 2 out]
                        n373 = call <vilib>:"Clear Errors.vi"("error in (no error)"=w616) -> ()  [unwired: 6 in, 1 out]
                      }
                      frame #1 {
                        n374 = String To Path(string=w631) -> (path=w625:path)
                        n375 = TDMS Open(5:FALSE, 6:FALSE, 10:T14."create or replace" ("operation (0:open)"), 11:w625) -> (0:w627:errorcluster, 3:→"LAB03-1 (TDMS)":refnum<k34>)  [unwired: 3 in]
                        n376 = local write "data file error"(w627) -> ()
                      }
                      frame #2 {
                        n377 = local read "LAB03-1 (SET)"() -> (w637:T5)
                        n378 = local read "LAB03-1 (TDMS)"() -> (w648:refnum<k34>)
                        n379 = Build Array("Testers Name", "Description", "Set Test Cycles", "T-Rise minutes", "T-Rise Deg C") -> (w638:string[])
                        n380 = Unbundle(w637) -> ("NAME"=w636:string, "DESCRIPTION"=w635:string, "CYCLES"=w634:dbl, "T-RISE mins"=w633:dbl, "T-RISE deg C"=w632:dbl)
                        n381 = Number To Decimal String(number=w634) -> (decimal integer string=w647:string)  [unwired: 1 in]
                        n382 = Number To Decimal String(number=w633) -> (decimal integer string=w646:string)  [unwired: 1 in]
                        n383 = Number To Decimal String(number=w632) -> (decimal integer string=w645:string)  [unwired: 1 in]
                        n384 = Build Array(w636, w635, w647, w646, w645) -> (w644:string[])
                        n385 = TDMS Set Properties(5:w644, 7:w638, 11:w648) -> ()  [unwired: 3 in, 4 out]
                      }
                      frame #3 {
                        w650 = 0.0
                        n386 = local read "LAB03-1 (DISP)"() -> (w652:T4)
                        n387 = Bundle(cluster=w652, "CYCLE"=w650, "MINS"=w650, "STATUS"="RUN") -> (w651:T4)
                        n388 = local write "LAB03-1 (DISP)"(w651) -> ()
                      }
                      frame #4 {
                        n389 = local read "LAB03-1 (SIG)"() -> (w655:T2)
                        n390 = local read "LAB03-1 (TEMP START)"() -> (w657:cluster{"TL":dbl, "TN":dbl})
                        n391 = Unbundle(w655) -> ("Tmp Live"=w654:dbl, "Tmp Neut"=w653:dbl)  [unwired: 3 out]
                        n392 = Bundle(cluster=w657, "TL"=w654, "TN"=w653) -> (w656:cluster{"TL":dbl, "TN":dbl})
                        n393 = local write "LAB03-1 (TEMP START)"(w656) -> ()
                      }
                    }
                  }
                }
              }
              event "LAB03-2 RUN": Value Change {
                n394 = event-data() -> ("NewVal"=w658:bool)  [unwired: 1 in, 5 out]
                n395 = case shown="True" w658 {
                  tunnel: w662 -> [_ w684]
                  tunnel: w661 -> [_ w683]
                  tunnel: w659 -> [w663 w682]
                  tunnel: w660 -> [_ w681]
                  frame False {
                    # "stop test"
                    n396 = stacked-sequence {
                      tunnel: w663 -> [w669 _]
                      frame #0 {
                        n397 = local read "LAB03-2 (DISP)"() -> (w668:T4)
                        n398 = Unbundle(w668) -> ("CYCLE"=w666:dbl, "MINS"=w667:dbl)  [unwired: 1 out]
                        n399 = case shown="\"CYCLE TEST\"" w669 {
                          tunnel: w667 -> [_ _ w676]
                          tunnel: w666 -> [w674 w675 _]
                          tunnel: [w674 w675 w676] -> w665
                          frame "TEST SET UP", Default {
                          }
                          frame "CYCLE TEST" {
                          }
                          frame "T-RISE TEST" {
                          }
                        }
                        n400 = local read "LAB03-2 (TDMS)"() -> (w673:refnum<k34>)
                        n401 = Build Array("STOPPED") -> (w670:string[])
                        n402 = Build Array(w665) -> (w664:dbl[])
                        n403 = TDMS Write(0:w673, 5:"TEST RESULT", 7:w670, 9:w664) -> ()  [unwired: 2 in, 4 out]
                      }
                      frame #1 {
                        n404 = local read "LAB03-2 (DISP)"() -> (w680:T4)
                        n405 = Bundle(cluster=w680, "STATUS"="STOP") -> (w678:T4)  [unwired: 2 in]
                        n406 = local write "LAB03-2 (RESULT)"(FALSE) -> ()
                        n407 = local write "LAB03-2 (DISP)"(w678) -> ()
                      }
                    }
                  }
                  frame True {
                    # "start new test and create test file"
                    n408 = stacked-sequence {
                      seq-local: [w690 _ _ _ _] -> [_ w709 _ _ _]
                      tunnel: w684 -> [w699 _ _ _ _]
                      tunnel: w683 -> [w697 _ _ _ _]
                      tunnel: w682 -> [w696 _ _ _ _]
                      tunnel: w681 -> [w687 _ _ _ _]
                      frame #0 {
                        n409 = local read "LAB03-2 (SET)"() -> (w689:T5)
                        n410 = case shown="\"TEST SET UP\", Default" w696 {
                          tunnel: ["TEST SET UP-" "CYCLE TEST-" "T-RISE TEST-"] -> w692
                          frame "TEST SET UP", Default {
                          }
                          frame "CYCLE TEST" {
                          }
                          frame "T-RISE TEST" {
                          }
                        }
                        n411 = Unbundle(w689) -> ("DESCRIPTION"=w688:string)  [unwired: 4 out]
                        n412 = Concatenate Strings(w699, "LAB03-2\\", w697, "\\") -> (w693:string)
                        n413 = String To Path(string=w693) -> (path=w695:path)
                        n414 = Concatenate Strings(w693, w692, w688, "-", w687, ".tdms") -> (w690:string)
                        n415 = Create Folder(path (use dialog)=w695) -> (error out=w694:errorcluster)  [unwired: 2 in, 2 out]
                        n416 = call <vilib>:"Clear Errors.vi"("error in (no error)"=w694) -> ()  [unwired: 6 in, 1 out]
                      }
                      frame #1 {
                        n417 = String To Path(string=w709) -> (path=w703:path)
                        n418 = TDMS Open(5:FALSE, 6:FALSE, 10:T14."create or replace" ("operation (0:open)"), 11:w703) -> (0:w705:errorcluster, 3:→"LAB03-2 (TDMS)":refnum<k34>)  [unwired: 3 in]
                        n419 = local write "data file error"(w705) -> ()
                      }
                      frame #2 {
                        n420 = local read "LAB03-2 (SET)"() -> (w715:T5)
                        n421 = local read "LAB03-2 (TDMS)"() -> (w726:refnum<k34>)
                        n422 = Build Array("Testers Name", "Description", "Set Test Cycles", "T-Rise minutes", "T-Rise Deg C") -> (w716:string[])
                        n423 = Unbundle(w715) -> ("NAME"=w714:string, "DESCRIPTION"=w713:string, "CYCLES"=w712:dbl, "T-RISE mins"=w711:dbl, "T-RISE deg C"=w710:dbl)
                        n424 = Number To Decimal String(number=w712) -> (decimal integer string=w725:string)  [unwired: 1 in]
                        n425 = Number To Decimal String(number=w711) -> (decimal integer string=w724:string)  [unwired: 1 in]
                        n426 = Number To Decimal String(number=w710) -> (decimal integer string=w723:string)  [unwired: 1 in]
                        n427 = Build Array(w714, w713, w725, w724, w723) -> (w722:string[])
                        n428 = TDMS Set Properties(5:w722, 7:w716, 11:w726) -> ()  [unwired: 3 in, 4 out]
                      }
                      frame #3 {
                        w728 = 0.0
                        n429 = local read "LAB03-2 (DISP)"() -> (w730:T4)
                        n430 = Bundle(cluster=w730, "CYCLE"=w728, "MINS"=w728, "STATUS"="RUN") -> (w729:T4)
                        n431 = local write "LAB03-2 (DISP)"(w729) -> ()
                      }
                      frame #4 {
                        n432 = local read "LAB03-2 (SIG)"() -> (w733:T2)
                        n433 = local read "LAB03-2 (TEMP START)"() -> (w735:cluster{"TL":dbl, "TN":dbl})
                        n434 = Unbundle(w733) -> ("Tmp Live"=w732:dbl, "Tmp Neut"=w731:dbl)  [unwired: 3 out]
                        n435 = Bundle(cluster=w735, "TL"=w732, "TN"=w731) -> (w734:cluster{"TL":dbl, "TN":dbl})
                        n436 = local write "LAB03-2 (TEMP START)"(w734) -> ()
                      }
                    }
                  }
                }
              }
              event "LAB04-1 RUN": Value Change {
                n437 = event-data() -> ("NewVal"=w736:bool)  [unwired: 1 in, 5 out]
                n438 = case shown="True" w736 {
                  tunnel: w740 -> [_ w762]
                  tunnel: w739 -> [_ w761]
                  tunnel: w737 -> [w741 w760]
                  tunnel: w738 -> [_ w759]
                  frame False {
                    # "stop test"
                    n439 = stacked-sequence {
                      tunnel: w741 -> [w747 _]
                      frame #0 {
                        n440 = local read "LAB04-1 (DISP)"() -> (w746:T4)
                        n441 = Unbundle(w746) -> ("CYCLE"=w744:dbl, "MINS"=w745:dbl)  [unwired: 1 out]
                        n442 = case shown="\"CYCLE TEST\"" w747 {
                          tunnel: w745 -> [_ _ w754]
                          tunnel: w744 -> [w752 w753 _]
                          tunnel: [w752 w753 w754] -> w743
                          frame "TEST SET UP", Default {
                          }
                          frame "CYCLE TEST" {
                          }
                          frame "T-RISE TEST" {
                          }
                        }
                        n443 = local read "LAB04-1 (TDMS)"() -> (w751:refnum<k34>)
                        n444 = Build Array("STOPPED") -> (w748:string[])
                        n445 = Build Array(w743) -> (w742:dbl[])
                        n446 = TDMS Write(0:w751, 5:"TEST RESULT", 7:w748, 9:w742) -> ()  [unwired: 2 in, 4 out]
                      }
                      frame #1 {
                        n447 = local read "LAB04-1 (DISP)"() -> (w758:T4)
                        n448 = Bundle(cluster=w758, "STATUS"="STOP") -> (w756:T4)  [unwired: 2 in]
                        n449 = local write "LAB04-1 (RESULT)"(FALSE) -> ()
                        n450 = local write "LAB04-1 (DISP)"(w756) -> ()
                      }
                    }
                  }
                  frame True {
                    # "start new test and create test file"
                    n451 = stacked-sequence {
                      seq-local: [w768 _ _ _ _] -> [_ w787 _ _ _]
                      tunnel: w762 -> [w777 _ _ _ _]
                      tunnel: w761 -> [w775 _ _ _ _]
                      tunnel: w760 -> [w774 _ _ _ _]
                      tunnel: w759 -> [w765 _ _ _ _]
                      frame #0 {
                        n452 = local read "LAB04-1 (SET)"() -> (w767:T5)
                        n453 = case shown="\"TEST SET UP\", Default" w774 {
                          tunnel: ["TEST SET UP-" "CYCLE TEST-" "T-RISE TEST-"] -> w770
                          frame "TEST SET UP", Default {
                          }
                          frame "CYCLE TEST" {
                          }
                          frame "T-RISE TEST" {
                          }
                        }
                        n454 = Unbundle(w767) -> ("DESCRIPTION"=w766:string)  [unwired: 4 out]
                        n455 = Concatenate Strings(w777, "LAB04-1\\", w775, "\\") -> (w771:string)
                        n456 = String To Path(string=w771) -> (path=w773:path)
                        n457 = Concatenate Strings(w771, w770, w766, "-", w765, ".tdms") -> (w768:string)
                        n458 = Create Folder(path (use dialog)=w773) -> (error out=w772:errorcluster)  [unwired: 2 in, 2 out]
                        n459 = call <vilib>:"Clear Errors.vi"("error in (no error)"=w772) -> ()  [unwired: 6 in, 1 out]
                      }
                      frame #1 {
                        n460 = String To Path(string=w787) -> (path=w781:path)
                        n461 = TDMS Open(5:FALSE, 6:FALSE, 10:T14."create or replace" ("operation (0:open)"), 11:w781) -> (0:w783:errorcluster, 3:→"LAB04-1 (TDMS)":refnum<k34>)  [unwired: 3 in]
                        n462 = local write "data file error"(w783) -> ()
                      }
                      frame #2 {
                        n463 = local read "LAB04-1 (SET)"() -> (w793:T5)
                        n464 = local read "LAB04-1 (TDMS)"() -> (w804:refnum<k34>)
                        n465 = Build Array("Testers Name", "Description", "Set Test Cycles", "T-Rise minutes", "T-Rise Deg C") -> (w794:string[])
                        n466 = Unbundle(w793) -> ("NAME"=w792:string, "DESCRIPTION"=w791:string, "CYCLES"=w790:dbl, "T-RISE mins"=w789:dbl, "T-RISE deg C"=w788:dbl)
                        n467 = Number To Decimal String(number=w790) -> (decimal integer string=w803:string)  [unwired: 1 in]
                        n468 = Number To Decimal String(number=w789) -> (decimal integer string=w802:string)  [unwired: 1 in]
                        n469 = Number To Decimal String(number=w788) -> (decimal integer string=w801:string)  [unwired: 1 in]
                        n470 = Build Array(w792, w791, w803, w802, w801) -> (w800:string[])
                        n471 = TDMS Set Properties(5:w800, 7:w794, 11:w804) -> ()  [unwired: 3 in, 4 out]
                      }
                      frame #3 {
                        w806 = 0.0
                        n472 = local read "LAB04-1 (DISP)"() -> (w808:T4)
                        n473 = Bundle(cluster=w808, "CYCLE"=w806, "MINS"=w806, "STATUS"="RUN") -> (w807:T4)
                        n474 = local write "LAB04-1 (DISP)"(w807) -> ()
                      }
                      frame #4 {
                        n475 = local read "LAB04-1 (SIG)"() -> (w811:T2)
                        n476 = local read "LAB04-1 (TEMP START)"() -> (w813:cluster{"TL":dbl, "TN":dbl})
                        n477 = Unbundle(w811) -> ("Tmp Live"=w810:dbl, "Tmp Neut"=w809:dbl)  [unwired: 3 out]
                        n478 = Bundle(cluster=w813, "TL"=w810, "TN"=w809) -> (w812:cluster{"TL":dbl, "TN":dbl})
                        n479 = local write "LAB04-1 (TEMP START)"(w812) -> ()
                      }
                    }
                  }
                }
              }
              event "LAB04-2 RUN": Value Change {
                n480 = event-data() -> ("NewVal"=w814:bool)  [unwired: 1 in, 5 out]
                n481 = case shown="True" w814 {
                  tunnel: w818 -> [_ w840]
                  tunnel: w817 -> [_ w839]
                  tunnel: w815 -> [w819 w838]
                  tunnel: w816 -> [_ w837]
                  frame False {
                    # "stop test"
                    n482 = stacked-sequence {
                      tunnel: w819 -> [w825 _]
                      frame #0 {
                        n483 = local read "LAB04-2 (DISP)"() -> (w824:T4)
                        n484 = Unbundle(w824) -> ("CYCLE"=w822:dbl, "MINS"=w823:dbl)  [unwired: 1 out]
                        n485 = case shown="\"CYCLE TEST\"" w825 {
                          tunnel: w823 -> [_ _ w832]
                          tunnel: w822 -> [w830 w831 _]
                          tunnel: [w830 w831 w832] -> w821
                          frame "TEST SET UP", Default {
                          }
                          frame "CYCLE TEST" {
                          }
                          frame "T-RISE TEST" {
                          }
                        }
                        n486 = local read "LAB04-2 (TDMS)"() -> (w829:refnum<k34>)
                        n487 = Build Array("STOPPED") -> (w826:string[])
                        n488 = Build Array(w821) -> (w820:dbl[])
                        n489 = TDMS Write(0:w829, 5:"TEST RESULT", 7:w826, 9:w820) -> ()  [unwired: 2 in, 4 out]
                      }
                      frame #1 {
                        n490 = local read "LAB04-2 (DISP)"() -> (w836:T4)
                        n491 = Bundle(cluster=w836, "STATUS"="STOP") -> (w834:T4)  [unwired: 2 in]
                        n492 = local write "LAB04-2 (RESULT)"(FALSE) -> ()
                        n493 = local write "LAB04-2 (DISP)"(w834) -> ()
                      }
                    }
                  }
                  frame True {
                    # "start new test and create test file"
                    n494 = stacked-sequence {
                      seq-local: [w846 _ _ _ _] -> [_ w865 _ _ _]
                      tunnel: w840 -> [w855 _ _ _ _]
                      tunnel: w839 -> [w853 _ _ _ _]
                      tunnel: w838 -> [w852 _ _ _ _]
                      tunnel: w837 -> [w843 _ _ _ _]
                      frame #0 {
                        n495 = local read "LAB04-2 (SET)"() -> (w845:T5)
                        n496 = case shown="\"TEST SET UP\", Default" w852 {
                          tunnel: ["TEST SET UP-" "CYCLE TEST-" "T-RISE TEST-"] -> w848
                          frame "TEST SET UP", Default {
                          }
                          frame "CYCLE TEST" {
                          }
                          frame "T-RISE TEST" {
                          }
                        }
                        n497 = Unbundle(w845) -> ("DESCRIPTION"=w844:string)  [unwired: 4 out]
                        n498 = Concatenate Strings(w855, "LAB04-2\\", w853, "\\") -> (w849:string)
                        n499 = String To Path(string=w849) -> (path=w851:path)
                        n500 = Concatenate Strings(w849, w848, w844, "-", w843, ".tdms") -> (w846:string)
                        n501 = Create Folder(path (use dialog)=w851) -> (error out=w850:errorcluster)  [unwired: 2 in, 2 out]
                        n502 = call <vilib>:"Clear Errors.vi"("error in (no error)"=w850) -> ()  [unwired: 6 in, 1 out]
                      }
                      frame #1 {
                        n503 = String To Path(string=w865) -> (path=w859:path)
                        n504 = TDMS Open(5:FALSE, 6:FALSE, 10:T14."create or replace" ("operation (0:open)"), 11:w859) -> (0:w861:errorcluster, 3:→"LAB04-2 (TDMS)":refnum<k34>)  [unwired: 3 in]
                        n505 = local write "data file error"(w861) -> ()
                      }
                      frame #2 {
                        n506 = local read "LAB04-2 (SET)"() -> (w871:T5)
                        n507 = local read "LAB04-2 (TDMS)"() -> (w882:refnum<k34>)
                        n508 = Build Array("Testers Name", "Description", "Set Test Cycles", "T-Rise minutes", "T-Rise Deg C") -> (w872:string[])
                        n509 = Unbundle(w871) -> ("NAME"=w870:string, "DESCRIPTION"=w869:string, "CYCLES"=w868:dbl, "T-RISE mins"=w867:dbl, "T-RISE deg C"=w866:dbl)
                        n510 = Number To Decimal String(number=w868) -> (decimal integer string=w881:string)  [unwired: 1 in]
                        n511 = Number To Decimal String(number=w867) -> (decimal integer string=w880:string)  [unwired: 1 in]
                        n512 = Number To Decimal String(number=w866) -> (decimal integer string=w879:string)  [unwired: 1 in]
                        n513 = Build Array(w870, w869, w881, w880, w879) -> (w878:string[])
                        n514 = TDMS Set Properties(5:w878, 7:w872, 11:w882) -> ()  [unwired: 3 in, 4 out]
                      }
                      frame #3 {
                        w884 = 0.0
                        n515 = local read "LAB04-2 (DISP)"() -> (w886:T4)
                        n516 = Bundle(cluster=w886, "CYCLE"=w884, "MINS"=w884, "STATUS"="RUN") -> (w885:T4)
                        n517 = local write "LAB04-2 (DISP)"(w885) -> ()
                      }
                      frame #4 {
                        n518 = local read "LAB04-2 (SIG)"() -> (w889:T2)
                        n519 = local read "LAB04-2 (TEMP START)"() -> (w891:cluster{"TL":dbl, "TN":dbl})
                        n520 = Unbundle(w889) -> ("Tmp Live"=w888:dbl, "Tmp Neut"=w887:dbl)  [unwired: 3 out]
                        n521 = Bundle(cluster=w891, "TL"=w888, "TN"=w887) -> (w890:cluster{"TL":dbl, "TN":dbl})
                        n522 = local write "LAB04-2 (TEMP START)"(w890) -> ()
                      }
                    }
                  }
                }
              }
              event "LAB05-1 RUN": Value Change {
                n523 = event-data() -> ("NewVal"=w892:bool)  [unwired: 1 in, 5 out]
                n524 = case shown="True" w892 {
                  tunnel: w896 -> [_ w918]
                  tunnel: w895 -> [_ w917]
                  tunnel: w893 -> [w897 w916]
                  tunnel: w894 -> [_ w915]
                  frame False {
                    # "stop test"
                    n525 = stacked-sequence {
                      tunnel: w897 -> [w903 _]
                      frame #0 {
                        n526 = local read "LAB05-1 (DISP)"() -> (w902:T4)
                        n527 = Unbundle(w902) -> ("CYCLE"=w900:dbl, "MINS"=w901:dbl)  [unwired: 1 out]
                        n528 = case shown="\"CYCLE TEST\"" w903 {
                          tunnel: w901 -> [_ _ w910]
                          tunnel: w900 -> [w908 w909 _]
                          tunnel: [w908 w909 w910] -> w899
                          frame "TEST SET UP", Default {
                          }
                          frame "CYCLE TEST" {
                          }
                          frame "T-RISE TEST" {
                          }
                        }
                        n529 = local read "LAB05-1 (TDMS)"() -> (w907:refnum<k34>)
                        n530 = Build Array("STOPPED") -> (w904:string[])
                        n531 = Build Array(w899) -> (w898:dbl[])
                        n532 = TDMS Write(0:w907, 5:"TEST RESULT", 7:w904, 9:w898) -> ()  [unwired: 2 in, 4 out]
                      }
                      frame #1 {
                        n533 = local read "LAB05-1 (DISP)"() -> (w914:T4)
                        n534 = Bundle(cluster=w914, "STATUS"="STOP") -> (w912:T4)  [unwired: 2 in]
                        n535 = local write "LAB05-1 (RESULT)"(FALSE) -> ()
                        n536 = local write "LAB05-1 (DISP)"(w912) -> ()
                      }
                    }
                  }
                  frame True {
                    # "start new test and create test file"
                    n537 = stacked-sequence {
                      seq-local: [w924 _ _ _ _] -> [_ w943 _ _ _]
                      tunnel: w918 -> [w933 _ _ _ _]
                      tunnel: w917 -> [w931 _ _ _ _]
                      tunnel: w916 -> [w930 _ _ _ _]
                      tunnel: w915 -> [w921 _ _ _ _]
                      frame #0 {
                        n538 = local read "LAB05-1 (SET)"() -> (w923:T5)
                        n539 = case shown="\"TEST SET UP\", Default" w930 {
                          tunnel: ["TEST SET UP-" "CYCLE TEST-" "T-RISE TEST-"] -> w926
                          frame "TEST SET UP", Default {
                          }
                          frame "CYCLE TEST" {
                          }
                          frame "T-RISE TEST" {
                          }
                        }
                        n540 = Unbundle(w923) -> ("DESCRIPTION"=w922:string)  [unwired: 4 out]
                        n541 = Concatenate Strings(w933, "LAB05-1\\", w931, "\\") -> (w927:string)
                        n542 = String To Path(string=w927) -> (path=w929:path)
                        n543 = Concatenate Strings(w927, w926, w922, "-", w921, ".tdms") -> (w924:string)
                        n544 = Create Folder(path (use dialog)=w929) -> (error out=w928:errorcluster)  [unwired: 2 in, 2 out]
                        n545 = call <vilib>:"Clear Errors.vi"("error in (no error)"=w928) -> ()  [unwired: 6 in, 1 out]
                      }
                      frame #1 {
                        n546 = String To Path(string=w943) -> (path=w937:path)
                        n547 = TDMS Open(5:FALSE, 6:FALSE, 10:T14."create or replace" ("operation (0:open)"), 11:w937) -> (0:w939:errorcluster, 3:→"LAB05-1 (TDMS)":refnum<k34>)  [unwired: 3 in]
                        n548 = local write "data file error"(w939) -> ()
                      }
                      frame #2 {
                        n549 = local read "LAB05-1 (SET)"() -> (w949:T5)
                        n550 = local read "LAB05-1 (TDMS)"() -> (w960:refnum<k34>)
                        n551 = Build Array("Testers Name", "Description", "Set Test Cycles", "T-Rise minutes", "T-Rise Deg C") -> (w950:string[])
                        n552 = Unbundle(w949) -> ("NAME"=w948:string, "DESCRIPTION"=w947:string, "CYCLES"=w946:dbl, "T-RISE mins"=w945:dbl, "T-RISE deg C"=w944:dbl)
                        n553 = Number To Decimal String(number=w946) -> (decimal integer string=w959:string)  [unwired: 1 in]
                        n554 = Number To Decimal String(number=w945) -> (decimal integer string=w958:string)  [unwired: 1 in]
                        n555 = Number To Decimal String(number=w944) -> (decimal integer string=w957:string)  [unwired: 1 in]
                        n556 = Build Array(w948, w947, w959, w958, w957) -> (w956:string[])
                        n557 = TDMS Set Properties(5:w956, 7:w950, 11:w960) -> ()  [unwired: 3 in, 4 out]
                      }
                      frame #3 {
                        w962 = 0.0
                        n558 = local read "LAB05-1 (DISP)"() -> (w964:T4)
                        n559 = Bundle(cluster=w964, "CYCLE"=w962, "MINS"=w962, "STATUS"="RUN") -> (w963:T4)
                        n560 = local write "LAB05-1 (DISP)"(w963) -> ()
                      }
                      frame #4 {
                        n561 = local read "LAB05-1 (SIG)"() -> (w967:T2)
                        n562 = local read "LAB05-1 (TEMP START)"() -> (w969:cluster{"TL":dbl, "TN":dbl})
                        n563 = Unbundle(w967) -> ("Tmp Live"=w966:dbl, "Tmp Neut"=w965:dbl)  [unwired: 3 out]
                        n564 = Bundle(cluster=w969, "TL"=w966, "TN"=w965) -> (w968:cluster{"TL":dbl, "TN":dbl})
                        n565 = local write "LAB05-1 (TEMP START)"(w968) -> ()
                      }
                    }
                  }
                }
              }
              event "LAB05-2 RUN": Value Change {
                n566 = event-data() -> ("NewVal"=w970:bool)  [unwired: 1 in, 5 out]
                n567 = case shown="True" w970 {
                  tunnel: w974 -> [_ w996]
                  tunnel: w973 -> [_ w995]
                  tunnel: w971 -> [w975 w994]
                  tunnel: w972 -> [_ w993]
                  frame False {
                    # "stop test"
                    n568 = stacked-sequence {
                      tunnel: w975 -> [w981 _]
                      frame #0 {
                        n569 = local read "LAB05-2 (DISP)"() -> (w980:T4)
                        n570 = Unbundle(w980) -> ("CYCLE"=w978:dbl, "MINS"=w979:dbl)  [unwired: 1 out]
                        n571 = case shown="\"CYCLE TEST\"" w981 {
                          tunnel: w979 -> [_ _ w988]
                          tunnel: w978 -> [w986 w987 _]
                          tunnel: [w986 w987 w988] -> w977
                          frame "TEST SET UP", Default {
                          }
                          frame "CYCLE TEST" {
                          }
                          frame "T-RISE TEST" {
                          }
                        }
                        n572 = local read "LAB05-2 (TDMS)"() -> (w985:refnum<k34>)
                        n573 = Build Array("STOPPED") -> (w982:string[])
                        n574 = Build Array(w977) -> (w976:dbl[])
                        n575 = TDMS Write(0:w985, 5:"TEST RESULT", 7:w982, 9:w976) -> ()  [unwired: 2 in, 4 out]
                      }
                      frame #1 {
                        n576 = local read "LAB05-2 (DISP)"() -> (w992:T4)
                        n577 = Bundle(cluster=w992, "STATUS"="STOP") -> (w990:T4)  [unwired: 2 in]
                        n578 = local write "LAB05-2 (RESULT)"(FALSE) -> ()
                        n579 = local write "LAB05-2 (DISP)"(w990) -> ()
                      }
                    }
                  }
                  frame True {
                    # "start new test and create test file"
                    n580 = stacked-sequence {
                      seq-local: [w1002 _ _ _ _] -> [_ w1021 _ _ _]
                      tunnel: w996 -> [w1011 _ _ _ _]
                      tunnel: w995 -> [w1009 _ _ _ _]
                      tunnel: w994 -> [w1008 _ _ _ _]
                      tunnel: w993 -> [w999 _ _ _ _]
                      frame #0 {
                        n581 = local read "LAB05-2 (SET)"() -> (w1001:T5)
                        n582 = case shown="\"TEST SET UP\", Default" w1008 {
                          tunnel: ["TEST SET UP-" "CYCLE TEST-" "T-RISE TEST-"] -> w1004
                          frame "TEST SET UP", Default {
                          }
                          frame "CYCLE TEST" {
                          }
                          frame "T-RISE TEST" {
                          }
                        }
                        n583 = Unbundle(w1001) -> ("DESCRIPTION"=w1000:string)  [unwired: 4 out]
                        n584 = Concatenate Strings(w1011, "LAB05-2\\", w1009, "\\") -> (w1005:string)
                        n585 = String To Path(string=w1005) -> (path=w1007:path)
                        n586 = Concatenate Strings(w1005, w1004, w1000, "-", w999, ".tdms") -> (w1002:string)
                        n587 = Create Folder(path (use dialog)=w1007) -> (error out=w1006:errorcluster)  [unwired: 2 in, 2 out]
                        n588 = call <vilib>:"Clear Errors.vi"("error in (no error)"=w1006) -> ()  [unwired: 6 in, 1 out]
                      }
                      frame #1 {
                        n589 = String To Path(string=w1021) -> (path=w1015:path)
                        n590 = TDMS Open(5:FALSE, 6:FALSE, 10:T14."create or replace" ("operation (0:open)"), 11:w1015) -> (0:w1017:errorcluster, 3:→"LAB05-2 (TDMS)":refnum<k34>)  [unwired: 3 in]
                        n591 = local write "data file error"(w1017) -> ()
                      }
                      frame #2 {
                        n592 = local read "LAB05-2 (SET)"() -> (w1027:T5)
                        n593 = local read "LAB05-2 (TDMS)"() -> (w1038:refnum<k34>)
                        n594 = Build Array("Testers Name", "Description", "Set Test Cycles", "T-Rise minutes", "T-Rise Deg C") -> (w1028:string[])
                        n595 = Unbundle(w1027) -> ("NAME"=w1026:string, "DESCRIPTION"=w1025:string, "CYCLES"=w1024:dbl, "T-RISE mins"=w1023:dbl, "T-RISE deg C"=w1022:dbl)
                        n596 = Number To Decimal String(number=w1024) -> (decimal integer string=w1037:string)  [unwired: 1 in]
                        n597 = Number To Decimal String(number=w1023) -> (decimal integer string=w1036:string)  [unwired: 1 in]
                        n598 = Number To Decimal String(number=w1022) -> (decimal integer string=w1035:string)  [unwired: 1 in]
                        n599 = Build Array(w1026, w1025, w1037, w1036, w1035) -> (w1034:string[])
                        n600 = TDMS Set Properties(5:w1034, 7:w1028, 11:w1038) -> ()  [unwired: 3 in, 4 out]
                      }
                      frame #3 {
                        w1040 = 0.0
                        n601 = local read "LAB05-2 (DISP)"() -> (w1042:T4)
                        n602 = Bundle(cluster=w1042, "CYCLE"=w1040, "MINS"=w1040, "STATUS"="RUN") -> (w1041:T4)
                        n603 = local write "LAB05-2 (DISP)"(w1041) -> ()
                      }
                      frame #4 {
                        n604 = local read "LAB05-2 (SIG)"() -> (w1045:T2)
                        n605 = local read "LAB05-2 (TEMP START)"() -> (w1047:cluster{"TL":dbl, "TN":dbl})
                        n606 = Unbundle(w1045) -> ("Tmp Live"=w1044:dbl, "Tmp Neut"=w1043:dbl)  [unwired: 3 out]
                        n607 = Bundle(cluster=w1047, "TL"=w1044, "TN"=w1043) -> (w1046:cluster{"TL":dbl, "TN":dbl})
                        n608 = local write "LAB05-2 (TEMP START)"(w1046) -> ()
                      }
                    }
                  }
                }
              }
            }
          }
          frame #4 {
            # "check if test cycles reached for cycle tests, if so then test pass"
            n609 = stacked-sequence {
              tunnel: w1067 -> [_ _ _ _ _ _ _ _ _ _]
              tunnel: w1066 -> [_ _ _ _ _ _ _ _ _ _]
              tunnel: w1065 -> [_ _ _ _ _ _ _ _ _ _]
              tunnel: w1064 -> [_ _ _ _ _ _ _ _ _ _]
              tunnel: w1063 -> [_ _ _ _ _ _ _ _ _ _]
              tunnel: w1062 -> [_ _ _ _ _ _ _ _ _ _]
              tunnel: w1061 -> [_ _ _ _ _ _ _ _ _ _]
              tunnel: w1060 -> [_ _ _ _ _ _ _ _ _ _]
              tunnel: w1059 -> [_ _ _ _ _ _ _ _ _ _]
              tunnel: w1058 -> [_ _ _ _ _ _ _ _ _ _]
              tunnel: w1057 -> [w1072 _ _ _ _ _ _ _ _ _]
              tunnel: w1056 -> [_ w1107 _ _ _ _ _ _ _ _]
              tunnel: w1055 -> [_ _ w1146 _ _ _ _ _ _ _]
              tunnel: w1054 -> [_ _ _ w1185 _ _ _ _ _ _]
              tunnel: w1053 -> [_ _ _ _ w1224 _ _ _ _ _]
              tunnel: w1052 -> [_ _ _ _ _ w1263 _ _ _ _]
              tunnel: w1051 -> [_ _ _ _ _ _ w1302 _ _ _]
              tunnel: w1050 -> [_ _ _ _ _ _ _ w1341 _ _]
              tunnel: w1049 -> [_ _ _ _ _ _ _ _ w1380 _]
              tunnel: w1048 -> [_ _ _ _ _ _ _ _ _ w1419]
              frame #0 {
                # "LAB01-1"
                n610 = Less?(x=w1072, y=2) -> (x < y?=w1070:bool)
                n611 = local read "LAB01-1 (DISP)"() -> (w1073:T4)
                n612 = Unbundle(w1073) -> ("STATUS"=w1074:string)  [unwired: 2 out]
                n613 = Equal?(x=w1074, y="RUN") -> (x = y?=w1069:bool)
                n614 = And(x=w1069, y=w1070) -> (x .and. y?=w1068:bool)
                n615 = case shown="True" w1068 {
                  tunnel: w1073 -> [_ w1077]
                  tunnel: w1072 -> [_ w1082]
                  frame False {
                  }
                  frame True {
                    n616 = local read "LAB01-1 (SET)"() -> (w1084:T5)
                    n617 = local read "LAB01-1 (TDMS)"() -> (w1076:refnum<k34>)
                    n618 = Unbundle(w1077) -> ("CYCLE"=w1083:dbl)  [unwired: 2 out]
                    n619 = Unbundle(w1084) -> ("CYCLES"=w1079:dbl, "T-RISE mins"=w1081:dbl)  [unwired: 3 out]
                    n620 = case shown="\"TEST SET UP\", Default" w1082 {
                      tunnel: w1081 -> [_ _ w1091]
                      tunnel: [w1086 w1088 w1091] -> w1080
                      tunnel: w1079 -> [w1086 w1088 _]
                      tunnel: ["TEST SET UP CYCLES" "CYCLES" "T-RISE TEST"] -> w1078
                      frame "TEST SET UP", Default {
                      }
                      frame "CYCLE TEST" {
                      }
                      frame "T-RISE TEST" {
                      }
                    }
                    n621 = Greater Or Equal?(x=w1083, y=w1079) -> (x >= y?=w1085:bool)
                    n622 = case shown="True" w1085 {
                      tunnel: w1080 -> [w1095 _]
                      tunnel: w1078 -> [w1094 _]
                      tunnel: w1077 -> [w1093 _]
                      tunnel: w1076 -> [w1092 _]
                      frame True {
                        n623 = stacked-sequence {
                          tunnel: w1095 -> [w1099 _]
                          tunnel: w1094 -> [w1097 _]
                          tunnel: w1093 -> [_ w1105]
                          tunnel: w1092 -> [w1096 _]
                          frame #0 {
                            n624 = Build Array(w1097) -> (w1100:string[])
                            n625 = Build Array(w1099) -> (w1098:dbl[])
                            n626 = TDMS Write(0:w1096, 5:"TEST PASS", 7:w1100, 9:w1098) -> (15:w1102:errorcluster)  [unwired: 2 in, 3 out]
                            n627 = local write "data file error"(w1102) -> ()
                          }
                          frame #1 {
                            n628 = Bundle(cluster=w1105, "STATUS"="CYCLE PASS") -> (w1103:T4)  [unwired: 2 in]
                            n629 = local write "LAB01-1 (RESULT)"(TRUE) -> ()
                            n630 = local write "LAB01-1 (DISP)"(w1103) -> ()
                          }
                        }
                      }
                      frame False {
                      }
                    }
                  }
                }
              }
              frame #1 {
                # "LAB01-2"
                n631 = Less?(x=w1107, y=2) -> (x < y?=w1110:bool)
                n632 = local read "LAB01-2 (DISP)"() -> (w1112:T4)
                n633 = Unbundle(w1112) -> ("STATUS"=w1113:string)  [unwired: 2 out]
                n634 = Equal?(x=w1113, y="RUN") -> (x = y?=w1109:bool)
                n635 = And(x=w1109, y=w1110) -> (x .and. y?=w1108:bool)
                n636 = case shown="True" w1108 {
                  tunnel: w1112 -> [_ w1116]
                  tunnel: w1107 -> [_ w1121]
                  frame False {
                  }
                  frame True {
                    n637 = local read "LAB01-2 (TDMS)"() -> (w1115:refnum<k34>)
                    n638 = local read "LAB01-2(SET)"() -> (w1123:T5)
                    n639 = Unbundle(w1116) -> ("CYCLE"=w1122:dbl)  [unwired: 2 out]
                    n640 = Unbundle(w1123) -> ("CYCLES"=w1118:dbl, "T-RISE mins"=w1120:dbl)  [unwired: 3 out]
                    n641 = case shown="\"TEST SET UP\", Default" w1121 {
                      tunnel: w1120 -> [_ _ w1130]
                      tunnel: [w1125 w1127 w1130] -> w1119
                      tunnel: w1118 -> [w1125 w1127 _]
                      tunnel: ["TEST SET UP CYCLES" "CYCLES" "T-RISE TEST"] -> w1117
                      frame "TEST SET UP", Default {
                      }
                      frame "CYCLE TEST" {
                      }
                      frame "T-RISE TEST" {
                      }
                    }
                    n642 = Greater Or Equal?(x=w1122, y=w1118) -> (x >= y?=w1124:bool)
                    n643 = case shown="True" w1124 {
                      tunnel: w1119 -> [w1134 _]
                      tunnel: w1117 -> [w1133 _]
                      tunnel: w1116 -> [w1132 _]
                      tunnel: w1115 -> [w1131 _]
                      frame True {
                        n644 = stacked-sequence {
                          tunnel: w1134 -> [w1138 _]
                          tunnel: w1133 -> [w1136 _]
                          tunnel: w1132 -> [_ w1144]
                          tunnel: w1131 -> [w1135 _]
                          frame #0 {
                            n645 = Build Array(w1136) -> (w1139:string[])
                            n646 = Build Array(w1138) -> (w1137:dbl[])
                            n647 = TDMS Write(0:w1135, 5:"TEST PASS", 7:w1139, 9:w1137) -> (15:w1141:errorcluster)  [unwired: 2 in, 3 out]
                            n648 = local write "data file error"(w1141) -> ()
                          }
                          frame #1 {
                            n649 = Bundle(cluster=w1144, "STATUS"="CYCLE PASS") -> (w1142:T4)  [unwired: 2 in]
                            n650 = local write "LAB01-2 (RESULT)"(TRUE) -> ()
                            n651 = local write "LAB01-2 (DISP)"(w1142) -> ()
                          }
                        }
                      }
                      frame False {
                      }
                    }
                  }
                }
              }
              frame #2 {
                # "LAB02-1"
                n652 = Less?(x=w1146, y=2) -> (x < y?=w1149:bool)
                n653 = local read "LAB02-1 (DISP)"() -> (w1151:T4)
                n654 = Unbundle(w1151) -> ("STATUS"=w1152:string)  [unwired: 2 out]
                n655 = Equal?(x=w1152, y="RUN") -> (x = y?=w1148:bool)
                n656 = And(x=w1148, y=w1149) -> (x .and. y?=w1147:bool)
                n657 = case shown="True" w1147 {
                  tunnel: w1151 -> [_ w1155]
                  tunnel: w1146 -> [_ w1160]
                  frame False {
                  }
                  frame True {
                    n658 = local read "LAB02-1 (SET)"() -> (w1162:T5)
                    n659 = local read "LAB02-1 (TDMS)"() -> (w1154:refnum<k34>)
                    n660 = Unbundle(w1155) -> ("CYCLE"=w1161:dbl)  [unwired: 2 out]
                    n661 = Unbundle(w1162) -> ("CYCLES"=w1157:dbl, "T-RISE mins"=w1159:dbl)  [unwired: 3 out]
                    n662 = case shown="\"TEST SET UP\", Default" w1160 {
                      tunnel: w1159 -> [_ _ w1169]
                      tunnel: [w1164 w1166 w1169] -> w1158
                      tunnel: w1157 -> [w1164 w1166 _]
                      tunnel: ["TEST SET UP CYCLES" "CYCLES" "T-RISE TEST"] -> w1156
                      frame "TEST SET UP", Default {
                      }
                      frame "CYCLE TEST" {
                      }
                      frame "T-RISE TEST" {
                      }
                    }
                    n663 = Greater Or Equal?(x=w1161, y=w1157) -> (x >= y?=w1163:bool)
                    n664 = case shown="True" w1163 {
                      tunnel: w1158 -> [w1173 _]
                      tunnel: w1156 -> [w1172 _]
                      tunnel: w1155 -> [w1171 _]
                      tunnel: w1154 -> [w1170 _]
                      frame True {
                        n665 = stacked-sequence {
                          tunnel: w1173 -> [w1177 _]
                          tunnel: w1172 -> [w1175 _]
                          tunnel: w1171 -> [_ w1183]
                          tunnel: w1170 -> [w1174 _]
                          frame #0 {
                            n666 = Build Array(w1175) -> (w1178:string[])
                            n667 = Build Array(w1177) -> (w1176:dbl[])
                            n668 = TDMS Write(0:w1174, 5:"TEST PASS", 7:w1178, 9:w1176) -> (15:w1180:errorcluster)  [unwired: 2 in, 3 out]
                            n669 = local write "data file error"(w1180) -> ()
                          }
                          frame #1 {
                            n670 = Bundle(cluster=w1183, "STATUS"="CYCLE PASS") -> (w1181:T4)  [unwired: 2 in]
                            n671 = local write "LAB02-1 (RESULT)"(TRUE) -> ()
                            n672 = local write "LAB02-1 (DISP)"(w1181) -> ()
                          }
                        }
                      }
                      frame False {
                      }
                    }
                  }
                }
              }
              frame #3 {
                # "LAB02-2"
                n673 = Less?(x=w1185, y=2) -> (x < y?=w1188:bool)
                n674 = local read "LAB02-2 (DISP)"() -> (w1190:T4)
                n675 = Unbundle(w1190) -> ("STATUS"=w1191:string)  [unwired: 2 out]
                n676 = Equal?(x=w1191, y="RUN") -> (x = y?=w1187:bool)
                n677 = And(x=w1187, y=w1188) -> (x .and. y?=w1186:bool)
                n678 = case shown="True" w1186 {
                  tunnel: w1190 -> [_ w1194]
                  tunnel: w1185 -> [_ w1199]
                  frame False {
                  }
                  frame True {
                    n679 = local read "LAB02-2 (SET)"() -> (w1201:T5)
                    n680 = local read "LAB02-2 (TDMS)"() -> (w1193:refnum<k34>)
                    n681 = Unbundle(w1194) -> ("CYCLE"=w1200:dbl)  [unwired: 2 out]
                    n682 = Unbundle(w1201) -> ("CYCLES"=w1196:dbl, "T-RISE mins"=w1198:dbl)  [unwired: 3 out]
                    n683 = case shown="\"TEST SET UP\", Default" w1199 {
                      tunnel: w1198 -> [_ _ w1208]
                      tunnel: [w1203 w1205 w1208] -> w1197
                      tunnel: w1196 -> [w1203 w1205 _]
                      tunnel: ["TEST SET UP CYCLES" "CYCLES" "T-RISE TEST"] -> w1195
                      frame "TEST SET UP", Default {
                      }
                      frame "CYCLE TEST" {
                      }
                      frame "T-RISE TEST" {
                      }
                    }
                    n684 = Greater Or Equal?(x=w1200, y=w1196) -> (x >= y?=w1202:bool)
                    n685 = case shown="True" w1202 {
                      tunnel: w1197 -> [w1212 _]
                      tunnel: w1195 -> [w1211 _]
                      tunnel: w1194 -> [w1210 _]
                      tunnel: w1193 -> [w1209 _]
                      frame True {
                        n686 = stacked-sequence {
                          tunnel: w1212 -> [w1216 _]
                          tunnel: w1211 -> [w1214 _]
                          tunnel: w1210 -> [_ w1222]
                          tunnel: w1209 -> [w1213 _]
                          frame #0 {
                            n687 = Build Array(w1214) -> (w1217:string[])
                            n688 = Build Array(w1216) -> (w1215:dbl[])
                            n689 = TDMS Write(0:w1213, 5:"TEST PASS", 7:w1217, 9:w1215) -> (15:w1219:errorcluster)  [unwired: 2 in, 3 out]
                            n690 = local write "data file error"(w1219) -> ()
                          }
                          frame #1 {
                            n691 = Bundle(cluster=w1222, "STATUS"="CYCLE PASS") -> (w1220:T4)  [unwired: 2 in]
                            n692 = local write "LAB02-2 (RESULT)"(TRUE) -> ()
                            n693 = local write "LAB02-2 (DISP)"(w1220) -> ()
                          }
                        }
                      }
                      frame False {
                      }
                    }
                  }
                }
              }
              frame #4 {
                # "LAB03-1"
                n694 = Less?(x=w1224, y=2) -> (x < y?=w1227:bool)
                n695 = local read "LAB03-1 (DISP)"() -> (w1229:T4)
                n696 = Unbundle(w1229) -> ("STATUS"=w1230:string)  [unwired: 2 out]
                n697 = Equal?(x=w1230, y="RUN") -> (x = y?=w1226:bool)
                n698 = And(x=w1226, y=w1227) -> (x .and. y?=w1225:bool)
                n699 = case shown="True" w1225 {
                  tunnel: w1229 -> [_ w1233]
                  tunnel: w1224 -> [_ w1238]
                  frame False {
                  }
                  frame True {
                    n700 = local read "LAB03-1 (SET)"() -> (w1240:T5)
                    n701 = local read "LAB03-1 (TDMS)"() -> (w1232:refnum<k34>)
                    n702 = Unbundle(w1233) -> ("CYCLE"=w1239:dbl)  [unwired: 2 out]
                    n703 = Unbundle(w1240) -> ("CYCLES"=w1235:dbl, "T-RISE mins"=w1237:dbl)  [unwired: 3 out]
                    n704 = case shown="\"TEST SET UP\", Default" w1238 {
                      tunnel: w1237 -> [_ _ w1247]
                      tunnel: [w1242 w1244 w1247] -> w1236
                      tunnel: w1235 -> [w1242 w1244 _]
                      tunnel: ["TEST SET UP CYCLES" "CYCLES" "T-RISE TEST"] -> w1234
                      frame "TEST SET UP", Default {
                      }
                      frame "CYCLE TEST" {
                      }
                      frame "T-RISE TEST" {
                      }
                    }
                    n705 = Greater Or Equal?(x=w1239, y=w1235) -> (x >= y?=w1241:bool)
                    n706 = case shown="True" w1241 {
                      tunnel: w1236 -> [w1251 _]
                      tunnel: w1234 -> [w1250 _]
                      tunnel: w1233 -> [w1249 _]
                      tunnel: w1232 -> [w1248 _]
                      frame True {
                        n707 = stacked-sequence {
                          tunnel: w1251 -> [w1255 _]
                          tunnel: w1250 -> [w1253 _]
                          tunnel: w1249 -> [_ w1261]
                          tunnel: w1248 -> [w1252 _]
                          frame #0 {
                            n708 = Build Array(w1253) -> (w1256:string[])
                            n709 = Build Array(w1255) -> (w1254:dbl[])
                            n710 = TDMS Write(0:w1252, 5:"TEST PASS", 7:w1256, 9:w1254) -> (15:w1258:errorcluster)  [unwired: 2 in, 3 out]
                            n711 = local write "data file error"(w1258) -> ()
                          }
                          frame #1 {
                            n712 = Bundle(cluster=w1261, "STATUS"="CYCLE PASS") -> (w1259:T4)  [unwired: 2 in]
                            n713 = local write "LAB03-1 (RESULT)"(TRUE) -> ()
                            n714 = local write "LAB03-1 (DISP)"(w1259) -> ()
                          }
                        }
                      }
                      frame False {
                      }
                    }
                  }
                }
              }
              frame #5 {
                # "LAB03-2"
                n715 = Less?(x=w1263, y=2) -> (x < y?=w1266:bool)
                n716 = local read "LAB03-2 (DISP)"() -> (w1268:T4)
                n717 = Unbundle(w1268) -> ("STATUS"=w1269:string)  [unwired: 2 out]
                n718 = Equal?(x=w1269, y="RUN") -> (x = y?=w1265:bool)
                n719 = And(x=w1265, y=w1266) -> (x .and. y?=w1264:bool)
                n720 = case shown="True" w1264 {
                  tunnel: w1268 -> [_ w1272]
                  tunnel: w1263 -> [_ w1277]
                  frame False {
                  }
                  frame True {
                    n721 = local read "LAB03-2 (SET)"() -> (w1279:T5)
                    n722 = local read "LAB03-2 (TDMS)"() -> (w1271:refnum<k34>)
                    n723 = Unbundle(w1272) -> ("CYCLE"=w1278:dbl)  [unwired: 2 out]
                    n724 = Unbundle(w1279) -> ("CYCLES"=w1274:dbl, "T-RISE mins"=w1276:dbl)  [unwired: 3 out]
                    n725 = case shown="\"TEST SET UP\", Default" w1277 {
                      tunnel: w1276 -> [_ _ w1286]
                      tunnel: [w1281 w1283 w1286] -> w1275
                      tunnel: w1274 -> [w1281 w1283 _]
                      tunnel: ["TEST SET UP CYCLES" "CYCLES" "T-RISE TEST"] -> w1273
                      frame "TEST SET UP", Default {
                      }
                      frame "CYCLE TEST" {
                      }
                      frame "T-RISE TEST" {
                      }
                    }
                    n726 = Greater Or Equal?(x=w1278, y=w1274) -> (x >= y?=w1280:bool)
                    n727 = case shown="True" w1280 {
                      tunnel: w1275 -> [w1290 _]
                      tunnel: w1273 -> [w1289 _]
                      tunnel: w1272 -> [w1288 _]
                      tunnel: w1271 -> [w1287 _]
                      frame True {
                        n728 = stacked-sequence {
                          tunnel: w1290 -> [w1294 _]
                          tunnel: w1289 -> [w1292 _]
                          tunnel: w1288 -> [_ w1300]
                          tunnel: w1287 -> [w1291 _]
                          frame #0 {
                            n729 = Build Array(w1292) -> (w1295:string[])
                            n730 = Build Array(w1294) -> (w1293:dbl[])
                            n731 = TDMS Write(0:w1291, 5:"TEST PASS", 7:w1295, 9:w1293) -> (15:w1297:errorcluster)  [unwired: 2 in, 3 out]
                            n732 = local write "data file error"(w1297) -> ()
                          }
                          frame #1 {
                            n733 = Bundle(cluster=w1300, "STATUS"="CYCLE PASS") -> (w1298:T4)  [unwired: 2 in]
                            n734 = local write "LAB03-2 (RESULT)"(TRUE) -> ()
                            n735 = local write "LAB03-2 (DISP)"(w1298) -> ()
                          }
                        }
                      }
                      frame False {
                      }
                    }
                  }
                }
              }
              frame #6 {
                # "LAB04-1"
                n736 = Less?(x=w1302, y=2) -> (x < y?=w1305:bool)
                n737 = local read "LAB04-1 (DISP)"() -> (w1307:T4)
                n738 = Unbundle(w1307) -> ("STATUS"=w1308:string)  [unwired: 2 out]
                n739 = Equal?(x=w1308, y="RUN") -> (x = y?=w1304:bool)
                n740 = And(x=w1304, y=w1305) -> (x .and. y?=w1303:bool)
                n741 = case shown="True" w1303 {
                  tunnel: w1307 -> [_ w1311]
                  tunnel: w1302 -> [_ w1316]
                  frame False {
                  }
                  frame True {
                    n742 = local read "LAB04-1 (SET)"() -> (w1318:T5)
                    n743 = local read "LAB04-1 (TDMS)"() -> (w1310:refnum<k34>)
                    n744 = Unbundle(w1311) -> ("CYCLE"=w1317:dbl)  [unwired: 2 out]
                    n745 = Unbundle(w1318) -> ("CYCLES"=w1313:dbl, "T-RISE mins"=w1315:dbl)  [unwired: 3 out]
                    n746 = case shown="\"TEST SET UP\", Default" w1316 {
                      tunnel: w1315 -> [_ _ w1325]
                      tunnel: [w1320 w1322 w1325] -> w1314
                      tunnel: w1313 -> [w1320 w1322 _]
                      tunnel: ["TEST SET UP CYCLES" "CYCLES" "T-RISE TEST"] -> w1312
                      frame "TEST SET UP", Default {
                      }
                      frame "CYCLE TEST" {
                      }
                      frame "T-RISE TEST" {
                      }
                    }
                    n747 = Greater Or Equal?(x=w1317, y=w1313) -> (x >= y?=w1319:bool)
                    n748 = case shown="True" w1319 {
                      tunnel: w1314 -> [w1329 _]
                      tunnel: w1312 -> [w1328 _]
                      tunnel: w1311 -> [w1327 _]
                      tunnel: w1310 -> [w1326 _]
                      frame True {
                        n749 = stacked-sequence {
                          tunnel: w1329 -> [w1333 _]
                          tunnel: w1328 -> [w1331 _]
                          tunnel: w1327 -> [_ w1339]
                          tunnel: w1326 -> [w1330 _]
                          frame #0 {
                            n750 = Build Array(w1331) -> (w1334:string[])
                            n751 = Build Array(w1333) -> (w1332:dbl[])
                            n752 = TDMS Write(0:w1330, 5:"TEST PASS", 7:w1334, 9:w1332) -> (15:w1336:errorcluster)  [unwired: 2 in, 3 out]
                            n753 = local write "data file error"(w1336) -> ()
                          }
                          frame #1 {
                            n754 = Bundle(cluster=w1339, "STATUS"="CYCLE PASS") -> (w1337:T4)  [unwired: 2 in]
                            n755 = local write "LAB04-1 (RESULT)"(TRUE) -> ()
                            n756 = local write "LAB04-1 (DISP)"(w1337) -> ()
                          }
                        }
                      }
                      frame False {
                      }
                    }
                  }
                }
              }
              frame #7 {
                # "LAB04-2"
                n757 = Less?(x=w1341, y=2) -> (x < y?=w1344:bool)
                n758 = local read "LAB04-2 (DISP)"() -> (w1346:T4)
                n759 = Unbundle(w1346) -> ("STATUS"=w1347:string)  [unwired: 2 out]
                n760 = Equal?(x=w1347, y="RUN") -> (x = y?=w1343:bool)
                n761 = And(x=w1343, y=w1344) -> (x .and. y?=w1342:bool)
                n762 = case shown="True" w1342 {
                  tunnel: w1346 -> [_ w1350]
                  tunnel: w1341 -> [_ w1355]
                  frame False {
                  }
                  frame True {
                    n763 = local read "LAB04-2 (SET)"() -> (w1357:T5)
                    n764 = local read "LAB04-2 (TDMS)"() -> (w1349:refnum<k34>)
                    n765 = Unbundle(w1350) -> ("CYCLE"=w1356:dbl)  [unwired: 2 out]
                    n766 = Unbundle(w1357) -> ("CYCLES"=w1352:dbl, "T-RISE mins"=w1354:dbl)  [unwired: 3 out]
                    n767 = case shown="\"TEST SET UP\", Default" w1355 {
                      tunnel: w1354 -> [_ _ w1364]
                      tunnel: [w1359 w1361 w1364] -> w1353
                      tunnel: w1352 -> [w1359 w1361 _]
                      tunnel: ["TEST SET UP CYCLES" "CYCLES" "T-RISE TEST"] -> w1351
                      frame "TEST SET UP", Default {
                      }
                      frame "CYCLE TEST" {
                      }
                      frame "T-RISE TEST" {
                      }
                    }
                    n768 = Greater Or Equal?(x=w1356, y=w1352) -> (x >= y?=w1358:bool)
                    n769 = case shown="True" w1358 {
                      tunnel: w1353 -> [w1368 _]
                      tunnel: w1351 -> [w1367 _]
                      tunnel: w1350 -> [w1366 _]
                      tunnel: w1349 -> [w1365 _]
                      frame True {
                        n770 = stacked-sequence {
                          tunnel: w1368 -> [w1372 _]
                          tunnel: w1367 -> [w1370 _]
                          tunnel: w1366 -> [_ w1378]
                          tunnel: w1365 -> [w1369 _]
                          frame #0 {
                            n771 = Build Array(w1370) -> (w1373:string[])
                            n772 = Build Array(w1372) -> (w1371:dbl[])
                            n773 = TDMS Write(0:w1369, 5:"TEST PASS", 7:w1373, 9:w1371) -> (15:w1375:errorcluster)  [unwired: 2 in, 3 out]
                            n774 = local write "data file error"(w1375) -> ()
                          }
                          frame #1 {
                            n775 = Bundle(cluster=w1378, "STATUS"="CYCLE PASS") -> (w1376:T4)  [unwired: 2 in]
                            n776 = local write "LAB04-2 (RESULT)"(TRUE) -> ()
                            n777 = local write "LAB04-2 (DISP)"(w1376) -> ()
                          }
                        }
                      }
                      frame False {
                      }
                    }
                  }
                }
              }
              frame #8 {
                # "LAB05-1"
                n778 = Less?(x=w1380, y=2) -> (x < y?=w1383:bool)
                n779 = local read "LAB05-1 (DISP)"() -> (w1385:T4)
                n780 = Unbundle(w1385) -> ("STATUS"=w1386:string)  [unwired: 2 out]
                n781 = Equal?(x=w1386, y="RUN") -> (x = y?=w1382:bool)
                n782 = And(x=w1382, y=w1383) -> (x .and. y?=w1381:bool)
                n783 = case shown="True" w1381 {
                  tunnel: w1385 -> [_ w1389]
                  tunnel: w1380 -> [_ w1394]
                  frame False {
                  }
                  frame True {
                    n784 = local read "LAB05-1 (SET)"() -> (w1396:T5)
                    n785 = local read "LAB05-1 (TDMS)"() -> (w1388:refnum<k34>)
                    n786 = Unbundle(w1389) -> ("CYCLE"=w1395:dbl)  [unwired: 2 out]
                    n787 = Unbundle(w1396) -> ("CYCLES"=w1391:dbl, "T-RISE mins"=w1393:dbl)  [unwired: 3 out]
                    n788 = case shown="\"TEST SET UP\", Default" w1394 {
                      tunnel: w1393 -> [_ _ w1403]
                      tunnel: [w1398 w1400 w1403] -> w1392
                      tunnel: w1391 -> [w1398 w1400 _]
                      tunnel: ["TEST SET UP CYCLES" "CYCLES" "T-RISE TEST"] -> w1390
                      frame "TEST SET UP", Default {
                      }
                      frame "CYCLE TEST" {
                      }
                      frame "T-RISE TEST" {
                      }
                    }
                    n789 = Greater Or Equal?(x=w1395, y=w1391) -> (x >= y?=w1397:bool)
                    n790 = case shown="True" w1397 {
                      tunnel: w1392 -> [w1407 _]
                      tunnel: w1390 -> [w1406 _]
                      tunnel: w1389 -> [w1405 _]
                      tunnel: w1388 -> [w1404 _]
                      frame True {
                        n791 = stacked-sequence {
                          tunnel: w1407 -> [w1411 _]
                          tunnel: w1406 -> [w1409 _]
                          tunnel: w1405 -> [_ w1417]
                          tunnel: w1404 -> [w1408 _]
                          frame #0 {
                            n792 = Build Array(w1409) -> (w1412:string[])
                            n793 = Build Array(w1411) -> (w1410:dbl[])
                            n794 = TDMS Write(0:w1408, 5:"TEST PASS", 7:w1412, 9:w1410) -> (15:w1414:errorcluster)  [unwired: 2 in, 3 out]
                            n795 = local write "data file error"(w1414) -> ()
                          }
                          frame #1 {
                            n796 = Bundle(cluster=w1417, "STATUS"="CYCLE PASS") -> (w1415:T4)  [unwired: 2 in]
                            n797 = local write "LAB05-1 (RESULT)"(TRUE) -> ()
                            n798 = local write "LAB05-1 (DISP)"(w1415) -> ()
                          }
                        }
                      }
                      frame False {
                      }
                    }
                  }
                }
              }
              frame #9 {
                # "LAB05-2"
                n799 = Less?(x=w1419, y=2) -> (x < y?=w1422:bool)
                n800 = local read "LAB05-2 (DISP)"() -> (w1424:T4)
                n801 = Unbundle(w1424) -> ("STATUS"=w1425:string)  [unwired: 2 out]
                n802 = Equal?(x=w1425, y="RUN") -> (x = y?=w1421:bool)
                n803 = And(x=w1421, y=w1422) -> (x .and. y?=w1420:bool)
                n804 = case shown="True" w1420 {
                  tunnel: w1424 -> [_ w1428]
                  tunnel: w1419 -> [_ w1433]
                  frame False {
                  }
                  frame True {
                    n805 = local read "LAB05-2 (SET)"() -> (w1435:T5)
                    n806 = local read "LAB05-1 (TDMS)"() -> (w1427:refnum<k34>)
                    n807 = Unbundle(w1428) -> ("CYCLE"=w1434:dbl)  [unwired: 2 out]
                    n808 = Unbundle(w1435) -> ("CYCLES"=w1430:dbl, "T-RISE mins"=w1432:dbl)  [unwired: 3 out]
                    n809 = case shown="\"TEST SET UP\", Default" w1433 {
                      tunnel: w1432 -> [_ _ w1442]
                      tunnel: [w1437 w1439 w1442] -> w1431
                      tunnel: w1430 -> [w1437 w1439 _]
                      tunnel: ["TEST SET UP CYCLES" "CYCLES" "T-RISE TEST"] -> w1429
                      frame "TEST SET UP", Default {
                      }
                      frame "CYCLE TEST" {
                      }
                      frame "T-RISE TEST" {
                      }
                    }
                    n810 = Greater Or Equal?(x=w1434, y=w1430) -> (x >= y?=w1436:bool)
                    n811 = case shown="True" w1436 {
                      tunnel: w1431 -> [w1446 _]
                      tunnel: w1429 -> [w1445 _]
                      tunnel: w1428 -> [w1444 _]
                      tunnel: w1427 -> [w1443 _]
                      frame True {
                        n812 = stacked-sequence {
                          tunnel: w1446 -> [w1450 _]
                          tunnel: w1445 -> [w1448 _]
                          tunnel: w1444 -> [_ w1456]
                          tunnel: w1443 -> [w1447 _]
                          frame #0 {
                            n813 = Build Array(w1448) -> (w1451:string[])
                            n814 = Build Array(w1450) -> (w1449:dbl[])
                            n815 = TDMS Write(0:w1447, 5:"TEST PASS", 7:w1451, 9:w1449) -> (15:w1453:errorcluster)  [unwired: 2 in, 3 out]
                            n816 = local write "data file error"(w1453) -> ()
                          }
                          frame #1 {
                            n817 = Bundle(cluster=w1456, "STATUS"="CYCLE PASS") -> (w1454:T4)  [unwired: 2 in]
                            n818 = local write "LAB05-2 (RESULT)"(TRUE) -> ()
                            n819 = local write "LAB05-2 (DISP)"(w1454) -> ()
                          }
                        }
                      }
                      frame False {
                      }
                    }
                  }
                }
              }
            }
          }
          frame #5 {
            # "check if test cycles reached for temperature rise test"
            n820 = stacked-sequence {
              tunnel: w1478 -> [_ _ _ _ _ _ _ _ _ _]
              tunnel: w1477 -> [_ _ _ _ _ _ _ _ _ _]
              tunnel: w1476 -> [_ _ _ _ _ _ _ _ _ _]
              tunnel: w1475 -> [_ _ _ _ _ _ _ _ _ _]
              tunnel: w1474 -> [_ _ _ _ _ _ _ _ _ _]
              tunnel: w1473 -> [_ _ _ _ _ _ _ _ _ _]
              tunnel: w1472 -> [_ _ _ _ _ _ _ _ _ _]
              tunnel: w1471 -> [_ _ _ _ _ _ _ _ _ _]
              tunnel: w1470 -> [_ _ _ _ _ _ _ _ _ _]
              tunnel: w1469 -> [_ _ _ _ _ _ _ _ _ _]
              tunnel: w1468 -> [w1484 _ _ _ _ _ _ _ _ _]
              tunnel: w1467 -> [w1479 w1510 w1540 w1570 w1600 w1630 w1660 w1690 w1720 w1750]
              tunnel: w1466 -> [_ w1509 _ _ _ _ _ _ _ _]
              tunnel: w1465 -> [_ _ w1539 _ _ _ _ _ _ _]
              tunnel: w1464 -> [_ _ _ w1569 _ _ _ _ _ _]
              tunnel: w1463 -> [_ _ _ _ w1599 _ _ _ _ _]
              tunnel: w1462 -> [_ _ _ _ _ w1629 _ _ _ _]
              tunnel: w1461 -> [_ _ _ _ _ _ w1659 _ _ _]
              tunnel: w1460 -> [_ _ _ _ _ _ _ w1689 _ _]
              tunnel: w1459 -> [_ _ _ _ _ _ _ _ w1719 _]
              tunnel: w1458 -> [_ _ _ _ _ _ _ _ _ w1749]
              frame #0 {
                # "LAB01-1"
                n821 = Equal?(x=w1484, y=2) -> (x = y?=w1482:bool)
                n822 = local read "LAB01-1 (DISP)"() -> (w1485:T4)
                n823 = Unbundle(w1485) -> ("STATUS"=w1486:string)  [unwired: 2 out]
                n824 = Equal?(x=w1486, y="RUN") -> (x = y?=w1481:bool)
                n825 = And(x=w1481, y=w1482) -> (x .and. y?=w1480:bool)
                n826 = case shown="True" w1480 {
                  tunnel: w1485 -> [_ w1489]
                  tunnel: w1479 -> [_ w1492]
                  frame False {
                  }
                  frame True {
                    n827 = local read "LAB01-1 (SET)"() -> (w1491:T5)
                    n828 = local read "LAB01-1 (TDMS)"() -> (w1488:refnum<k34>)
                    n829 = Unbundle(w1489) -> ("CYCLE"=w1493:dbl)  [unwired: 2 out]
                    n830 = Unbundle(w1491) -> ("T-RISE mins"=w1490:dbl)  [unwired: 4 out]
                    n831 = Greater Or Equal?(x=w1493, y=w1492) -> (x >= y?=w1494:bool)
                    n832 = case shown="True" w1494 {
                      tunnel: w1490 -> [w1497 _]
                      tunnel: w1489 -> [w1496 _]
                      tunnel: w1488 -> [w1495 _]
                      frame True {
                        n833 = stacked-sequence {
                          tunnel: w1497 -> [w1500 _]
                          tunnel: w1496 -> [_ w1505]
                          tunnel: w1495 -> [w1498 _]
                          frame #0 {
                            n834 = Build Array("T-RISE") -> (w1502:string[])
                            n835 = Build Array(w1500) -> (w1501:dbl[])
                            n836 = TDMS Write(0:w1498, 5:"TEST PASS", 7:w1502, 9:w1501) -> (15:w1504:errorcluster)  [unwired: 2 in, 3 out]
                            n837 = local write "data file error"(w1504) -> ()
                          }
                          frame #1 {
                            n838 = Bundle(cluster=w1505, "STATUS"="T-RISE PASS") -> (w1507:T4)  [unwired: 2 in]
                            n839 = local write "LAB01-1 (RESULT)"(TRUE) -> ()
                            n840 = local write "LAB01-1 (DISP)"(w1507) -> ()
                          }
                        }
                      }
                      frame False {
                      }
                    }
                  }
                }
              }
              frame #1 {
                # "LAB01-2"
                n841 = Equal?(x=w1509, y=2) -> (x = y?=w1513:bool)
                n842 = local read "LAB01-2 (DISP)"() -> (w1515:T4)
                n843 = Unbundle(w1515) -> ("STATUS"=w1516:string)  [unwired: 2 out]
                n844 = Equal?(x=w1516, y="RUN") -> (x = y?=w1512:bool)
                n845 = And(x=w1512, y=w1513) -> (x .and. y?=w1511:bool)
                n846 = case shown="True" w1511 {
                  tunnel: w1515 -> [_ w1519]
                  tunnel: w1510 -> [_ w1522]
                  frame False {
                  }
                  frame True {
                    n847 = local read "LAB01-2(SET)"() -> (w1521:T5)
                    n848 = local read "LAB01-2 (TDMS)"() -> (w1518:refnum<k34>)
                    n849 = Unbundle(w1519) -> ("CYCLE"=w1523:dbl)  [unwired: 2 out]
                    n850 = Unbundle(w1521) -> ("T-RISE mins"=w1520:dbl)  [unwired: 4 out]
                    n851 = Greater Or Equal?(x=w1523, y=w1522) -> (x >= y?=w1524:bool)
                    n852 = case shown="True" w1524 {
                      tunnel: w1520 -> [w1527 _]
                      tunnel: w1519 -> [w1526 _]
                      tunnel: w1518 -> [w1525 _]
                      frame True {
                        n853 = stacked-sequence {
                          tunnel: w1527 -> [w1530 _]
                          tunnel: w1526 -> [_ w1535]
                          tunnel: w1525 -> [w1528 _]
                          frame #0 {
                            n854 = Build Array("T-RISE") -> (w1532:string[])
                            n855 = Build Array(w1530) -> (w1531:dbl[])
                            n856 = TDMS Write(0:w1528, 5:"TEST PASS", 7:w1532, 9:w1531) -> (15:w1534:errorcluster)  [unwired: 2 in, 3 out]
                            n857 = local write "data file error"(w1534) -> ()
                          }
                          frame #1 {
                            n858 = Bundle(cluster=w1535, "STATUS"="T-RISE PASS") -> (w1537:T4)  [unwired: 2 in]
                            n859 = local write "LAB01-2 (RESULT)"(TRUE) -> ()
                            n860 = local write "LAB01-2 (DISP)"(w1537) -> ()
                          }
                        }
                      }
                      frame False {
                      }
                    }
                  }
                }
              }
              frame #2 {
                # "LAB02-1"
                n861 = Equal?(x=w1539, y=2) -> (x = y?=w1543:bool)
                n862 = local read "LAB02-1 (DISP)"() -> (w1545:T4)
                n863 = Unbundle(w1545) -> ("STATUS"=w1546:string)  [unwired: 2 out]
                n864 = Equal?(x=w1546, y="RUN") -> (x = y?=w1542:bool)
                n865 = And(x=w1542, y=w1543) -> (x .and. y?=w1541:bool)
                n866 = case shown="True" w1541 {
                  tunnel: w1545 -> [_ w1549]
                  tunnel: w1540 -> [_ w1552]
                  frame False {
                  }
                  frame True {
                    n867 = local read "LAB02-1 (SET)"() -> (w1551:T5)
                    n868 = local read "LAB02-1 (TDMS)"() -> (w1548:refnum<k34>)
                    n869 = Unbundle(w1549) -> ("CYCLE"=w1553:dbl)  [unwired: 2 out]
                    n870 = Unbundle(w1551) -> ("T-RISE mins"=w1550:dbl)  [unwired: 4 out]
                    n871 = Greater Or Equal?(x=w1553, y=w1552) -> (x >= y?=w1554:bool)
                    n872 = case shown="True" w1554 {
                      tunnel: w1550 -> [w1557 _]
                      tunnel: w1549 -> [w1556 _]
                      tunnel: w1548 -> [w1555 _]
                      frame True {
                        n873 = stacked-sequence {
                          tunnel: w1557 -> [w1560 _]
                          tunnel: w1556 -> [_ w1565]
                          tunnel: w1555 -> [w1558 _]
                          frame #0 {
                            n874 = Build Array("T-RISE") -> (w1562:string[])
                            n875 = Build Array(w1560) -> (w1561:dbl[])
                            n876 = TDMS Write(0:w1558, 5:"TEST PASS", 7:w1562, 9:w1561) -> (15:w1564:errorcluster)  [unwired: 2 in, 3 out]
                            n877 = local write "data file error"(w1564) -> ()
                          }
                          frame #1 {
                            n878 = Bundle(cluster=w1565, "STATUS"="T-RISE PASS") -> (w1567:T4)  [unwired: 2 in]
                            n879 = local write "LAB02-1 (RESULT)"(TRUE) -> ()
                            n880 = local write "LAB02-1 (DISP)"(w1567) -> ()
                          }
                        }
                      }
                      frame False {
                      }
                    }
                  }
                }
              }
              frame #3 {
                # "LAB02-2"
                n881 = Equal?(x=w1569, y=2) -> (x = y?=w1573:bool)
                n882 = local read "LAB02-2 (DISP)"() -> (w1575:T4)
                n883 = Unbundle(w1575) -> ("STATUS"=w1576:string)  [unwired: 2 out]
                n884 = Equal?(x=w1576, y="RUN") -> (x = y?=w1572:bool)
                n885 = And(x=w1572, y=w1573) -> (x .and. y?=w1571:bool)
                n886 = case shown="True" w1571 {
                  tunnel: w1575 -> [_ w1579]
                  tunnel: w1570 -> [_ w1582]
                  frame False {
                  }
                  frame True {
                    n887 = local read "LAB02-2 (SET)"() -> (w1581:T5)
                    n888 = local read "LAB02-2 (TDMS)"() -> (w1578:refnum<k34>)
                    n889 = Unbundle(w1579) -> ("CYCLE"=w1583:dbl)  [unwired: 2 out]
                    n890 = Unbundle(w1581) -> ("T-RISE mins"=w1580:dbl)  [unwired: 4 out]
                    n891 = Greater Or Equal?(x=w1583, y=w1582) -> (x >= y?=w1584:bool)
                    n892 = case shown="True" w1584 {
                      tunnel: w1580 -> [w1587 _]
                      tunnel: w1579 -> [w1586 _]
                      tunnel: w1578 -> [w1585 _]
                      frame True {
                        n893 = stacked-sequence {
                          tunnel: w1587 -> [w1590 _]
                          tunnel: w1586 -> [_ w1595]
                          tunnel: w1585 -> [w1588 _]
                          frame #0 {
                            n894 = Build Array("T-RISE") -> (w1592:string[])
                            n895 = Build Array(w1590) -> (w1591:dbl[])
                            n896 = TDMS Write(0:w1588, 5:"TEST PASS", 7:w1592, 9:w1591) -> (15:w1594:errorcluster)  [unwired: 2 in, 3 out]
                            n897 = local write "data file error"(w1594) -> ()
                          }
                          frame #1 {
                            n898 = Bundle(cluster=w1595, "STATUS"="T-RISE PASS") -> (w1597:T4)  [unwired: 2 in]
                            n899 = local write "LAB02-2 (RESULT)"(TRUE) -> ()
                            n900 = local write "LAB02-2 (DISP)"(w1597) -> ()
                          }
                        }
                      }
                      frame False {
                      }
                    }
                  }
                }
              }
              frame #4 {
                # "LAB03-1"
                n901 = Equal?(x=w1599, y=2) -> (x = y?=w1603:bool)
                n902 = local read "LAB03-1 (DISP)"() -> (w1605:T4)
                n903 = Unbundle(w1605) -> ("STATUS"=w1606:string)  [unwired: 2 out]
                n904 = Equal?(x=w1606, y="RUN") -> (x = y?=w1602:bool)
                n905 = And(x=w1602, y=w1603) -> (x .and. y?=w1601:bool)
                n906 = case shown="True" w1601 {
                  tunnel: w1605 -> [_ w1609]
                  tunnel: w1600 -> [_ w1612]
                  frame False {
                  }
                  frame True {
                    n907 = local read "LAB03-1 (SET)"() -> (w1611:T5)
                    n908 = local read "LAB03-1 (TDMS)"() -> (w1608:refnum<k34>)
                    n909 = Unbundle(w1609) -> ("CYCLE"=w1613:dbl)  [unwired: 2 out]
                    n910 = Unbundle(w1611) -> ("T-RISE mins"=w1610:dbl)  [unwired: 4 out]
                    n911 = Greater Or Equal?(x=w1613, y=w1612) -> (x >= y?=w1614:bool)
                    n912 = case shown="True" w1614 {
                      tunnel: w1610 -> [w1617 _]
                      tunnel: w1609 -> [w1616 _]
                      tunnel: w1608 -> [w1615 _]
                      frame True {
                        n913 = stacked-sequence {
                          tunnel: w1617 -> [w1620 _]
                          tunnel: w1616 -> [_ w1625]
                          tunnel: w1615 -> [w1618 _]
                          frame #0 {
                            n914 = Build Array("T-RISE") -> (w1622:string[])
                            n915 = Build Array(w1620) -> (w1621:dbl[])
                            n916 = TDMS Write(0:w1618, 5:"TEST PASS", 7:w1622, 9:w1621) -> (15:w1624:errorcluster)  [unwired: 2 in, 3 out]
                            n917 = local write "data file error"(w1624) -> ()
                          }
                          frame #1 {
                            n918 = Bundle(cluster=w1625, "STATUS"="T-RISE PASS") -> (w1627:T4)  [unwired: 2 in]
                            n919 = local write "LAB03-1 (RESULT)"(TRUE) -> ()
                            n920 = local write "LAB03-1 (DISP)"(w1627) -> ()
                          }
                        }
                      }
                      frame False {
                      }
                    }
                  }
                }
              }
              frame #5 {
                # "LAB03-2"
                n921 = Equal?(x=w1629, y=2) -> (x = y?=w1633:bool)
                n922 = local read "LAB03-2 (DISP)"() -> (w1635:T4)
                n923 = Unbundle(w1635) -> ("STATUS"=w1636:string)  [unwired: 2 out]
                n924 = Equal?(x=w1636, y="RUN") -> (x = y?=w1632:bool)
                n925 = And(x=w1632, y=w1633) -> (x .and. y?=w1631:bool)
                n926 = case shown="True" w1631 {
                  tunnel: w1635 -> [_ w1639]
                  tunnel: w1630 -> [_ w1642]
                  frame False {
                  }
                  frame True {
                    n927 = local read "LAB03-2 (SET)"() -> (w1641:T5)
                    n928 = local read "LAB03-2 (TDMS)"() -> (w1638:refnum<k34>)
                    n929 = Unbundle(w1639) -> ("CYCLE"=w1643:dbl)  [unwired: 2 out]
                    n930 = Unbundle(w1641) -> ("T-RISE mins"=w1640:dbl)  [unwired: 4 out]
                    n931 = Greater Or Equal?(x=w1643, y=w1642) -> (x >= y?=w1644:bool)
                    n932 = case shown="True" w1644 {
                      tunnel: w1640 -> [w1647 _]
                      tunnel: w1639 -> [w1646 _]
                      tunnel: w1638 -> [w1645 _]
                      frame True {
                        n933 = stacked-sequence {
                          tunnel: w1647 -> [w1650 _]
                          tunnel: w1646 -> [_ w1655]
                          tunnel: w1645 -> [w1648 _]
                          frame #0 {
                            n934 = Build Array("T-RISE") -> (w1652:string[])
                            n935 = Build Array(w1650) -> (w1651:dbl[])
                            n936 = TDMS Write(0:w1648, 5:"TEST PASS", 7:w1652, 9:w1651) -> (15:w1654:errorcluster)  [unwired: 2 in, 3 out]
                            n937 = local write "data file error"(w1654) -> ()
                          }
                          frame #1 {
                            n938 = Bundle(cluster=w1655, "STATUS"="T-RISE PASS") -> (w1657:T4)  [unwired: 2 in]
                            n939 = local write "LAB03-2 (RESULT)"(TRUE) -> ()
                            n940 = local write "LAB03-2 (DISP)"(w1657) -> ()
                          }
                        }
                      }
                      frame False {
                      }
                    }
                  }
                }
              }
              frame #6 {
                # "LAB04-1"
                n941 = Equal?(x=w1659, y=2) -> (x = y?=w1663:bool)
                n942 = local read "LAB04-1 (DISP)"() -> (w1665:T4)
                n943 = Unbundle(w1665) -> ("STATUS"=w1666:string)  [unwired: 2 out]
                n944 = Equal?(x=w1666, y="RUN") -> (x = y?=w1662:bool)
                n945 = And(x=w1662, y=w1663) -> (x .and. y?=w1661:bool)
                n946 = case shown="True" w1661 {
                  tunnel: w1665 -> [_ w1669]
                  tunnel: w1660 -> [_ w1672]
                  frame False {
                  }
                  frame True {
                    n947 = local read "LAB04-1 (SET)"() -> (w1671:T5)
                    n948 = local read "LAB04-1 (TDMS)"() -> (w1668:refnum<k34>)
                    n949 = Unbundle(w1669) -> ("CYCLE"=w1673:dbl)  [unwired: 2 out]
                    n950 = Unbundle(w1671) -> ("T-RISE mins"=w1670:dbl)  [unwired: 4 out]
                    n951 = Greater Or Equal?(x=w1673, y=w1672) -> (x >= y?=w1674:bool)
                    n952 = case shown="True" w1674 {
                      tunnel: w1670 -> [w1677 _]
                      tunnel: w1669 -> [w1676 _]
                      tunnel: w1668 -> [w1675 _]
                      frame True {
                        n953 = stacked-sequence {
                          tunnel: w1677 -> [w1680 _]
                          tunnel: w1676 -> [_ w1685]
                          tunnel: w1675 -> [w1678 _]
                          frame #0 {
                            n954 = Build Array("T-RISE") -> (w1682:string[])
                            n955 = Build Array(w1680) -> (w1681:dbl[])
                            n956 = TDMS Write(0:w1678, 5:"TEST PASS", 7:w1682, 9:w1681) -> (15:w1684:errorcluster)  [unwired: 2 in, 3 out]
                            n957 = local write "data file error"(w1684) -> ()
                          }
                          frame #1 {
                            n958 = Bundle(cluster=w1685, "STATUS"="T-RISE PASS") -> (w1687:T4)  [unwired: 2 in]
                            n959 = local write "LAB04-1 (RESULT)"(TRUE) -> ()
                            n960 = local write "LAB04-1 (DISP)"(w1687) -> ()
                          }
                        }
                      }
                      frame False {
                      }
                    }
                  }
                }
              }
              frame #7 {
                # "LAB04-2"
                n961 = Equal?(x=w1689, y=2) -> (x = y?=w1693:bool)
                n962 = local read "LAB04-2 (DISP)"() -> (w1695:T4)
                n963 = Unbundle(w1695) -> ("STATUS"=w1696:string)  [unwired: 2 out]
                n964 = Equal?(x=w1696, y="RUN") -> (x = y?=w1692:bool)
                n965 = And(x=w1692, y=w1693) -> (x .and. y?=w1691:bool)
                n966 = case shown="True" w1691 {
                  tunnel: w1695 -> [_ w1699]
                  tunnel: w1690 -> [_ w1702]
                  frame False {
                  }
                  frame True {
                    n967 = local read "LAB04-2 (SET)"() -> (w1701:T5)
                    n968 = local read "LAB04-2 (TDMS)"() -> (w1698:refnum<k34>)
                    n969 = Unbundle(w1699) -> ("CYCLE"=w1703:dbl)  [unwired: 2 out]
                    n970 = Unbundle(w1701) -> ("T-RISE mins"=w1700:dbl)  [unwired: 4 out]
                    n971 = Greater Or Equal?(x=w1703, y=w1702) -> (x >= y?=w1704:bool)
                    n972 = case shown="True" w1704 {
                      tunnel: w1700 -> [w1707 _]
                      tunnel: w1699 -> [w1706 _]
                      tunnel: w1698 -> [w1705 _]
                      frame True {
                        n973 = stacked-sequence {
                          tunnel: w1707 -> [w1710 _]
                          tunnel: w1706 -> [_ w1715]
                          tunnel: w1705 -> [w1708 _]
                          frame #0 {
                            n974 = Build Array("T-RISE") -> (w1712:string[])
                            n975 = Build Array(w1710) -> (w1711:dbl[])
                            n976 = TDMS Write(0:w1708, 5:"TEST PASS", 7:w1712, 9:w1711) -> (15:w1714:errorcluster)  [unwired: 2 in, 3 out]
                            n977 = local write "data file error"(w1714) -> ()
                          }
                          frame #1 {
                            n978 = Bundle(cluster=w1715, "STATUS"="T-RISE PASS") -> (w1717:T4)  [unwired: 2 in]
                            n979 = local write "LAB04-2 (RESULT)"(TRUE) -> ()
                            n980 = local write "LAB04-2 (DISP)"(w1717) -> ()
                          }
                        }
                      }
                      frame False {
                      }
                    }
                  }
                }
              }
              frame #8 {
                # "LAB05-1"
                n981 = Equal?(x=w1719, y=2) -> (x = y?=w1723:bool)
                n982 = local read "LAB05-1 (DISP)"() -> (w1725:T4)
                n983 = Unbundle(w1725) -> ("STATUS"=w1726:string)  [unwired: 2 out]
                n984 = Equal?(x=w1726, y="RUN") -> (x = y?=w1722:bool)
                n985 = And(x=w1722, y=w1723) -> (x .and. y?=w1721:bool)
                n986 = case shown="True" w1721 {
                  tunnel: w1725 -> [_ w1729]
                  tunnel: w1720 -> [_ w1732]
                  frame False {
                  }
                  frame True {
                    n987 = local read "LAB05-1 (SET)"() -> (w1731:T5)
                    n988 = local read "LAB05-1 (TDMS)"() -> (w1728:refnum<k34>)
                    n989 = Unbundle(w1729) -> ("CYCLE"=w1733:dbl)  [unwired: 2 out]
                    n990 = Unbundle(w1731) -> ("T-RISE mins"=w1730:dbl)  [unwired: 4 out]
                    n991 = Greater Or Equal?(x=w1733, y=w1732) -> (x >= y?=w1734:bool)
                    n992 = case shown="True" w1734 {
                      tunnel: w1730 -> [w1737 _]
                      tunnel: w1729 -> [w1736 _]
                      tunnel: w1728 -> [w1735 _]
                      frame True {
                        n993 = stacked-sequence {
                          tunnel: w1737 -> [w1740 _]
                          tunnel: w1736 -> [_ w1745]
                          tunnel: w1735 -> [w1738 _]
                          frame #0 {
                            n994 = Build Array("T-RISE") -> (w1742:string[])
                            n995 = Build Array(w1740) -> (w1741:dbl[])
                            n996 = TDMS Write(0:w1738, 5:"TEST PASS", 7:w1742, 9:w1741) -> (15:w1744:errorcluster)  [unwired: 2 in, 3 out]
                            n997 = local write "data file error"(w1744) -> ()
                          }
                          frame #1 {
                            n998 = Bundle(cluster=w1745, "STATUS"="T-RISE PASS") -> (w1747:T4)  [unwired: 2 in]
                            n999 = local write "LAB05-1 (RESULT)"(TRUE) -> ()
                            n1000 = local write "LAB05-1 (DISP)"(w1747) -> ()
                          }
                        }
                      }
                      frame False {
                      }
                    }
                  }
                }
              }
              frame #9 {
                # "LAB05-2"
                n1001 = Equal?(x=w1749, y=2) -> (x = y?=w1753:bool)
                n1002 = local read "LAB05-2 (DISP)"() -> (w1755:T4)
                n1003 = Unbundle(w1755) -> ("STATUS"=w1756:string)  [unwired: 2 out]
                n1004 = Equal?(x=w1756, y="RUN") -> (x = y?=w1752:bool)
                n1005 = And(x=w1752, y=w1753) -> (x .and. y?=w1751:bool)
                n1006 = case shown="True" w1751 {
                  tunnel: w1755 -> [_ w1759]
                  tunnel: w1750 -> [_ w1762]
                  frame False {
                  }
                  frame True {
                    n1007 = local read "LAB05-2 (SET)"() -> (w1761:T5)
                    n1008 = local read "LAB05-2 (TDMS)"() -> (w1758:refnum<k34>)
                    n1009 = Unbundle(w1759) -> ("CYCLE"=w1763:dbl)  [unwired: 2 out]
                    n1010 = Unbundle(w1761) -> ("T-RISE mins"=w1760:dbl)  [unwired: 4 out]
                    n1011 = Greater Or Equal?(x=w1763, y=w1762) -> (x >= y?=w1764:bool)
                    n1012 = case shown="True" w1764 {
                      tunnel: w1760 -> [w1767 _]
                      tunnel: w1759 -> [w1766 _]
                      tunnel: w1758 -> [w1765 _]
                      frame True {
                        n1013 = stacked-sequence {
                          tunnel: w1767 -> [w1770 _]
                          tunnel: w1766 -> [_ w1775]
                          tunnel: w1765 -> [w1768 _]
                          frame #0 {
                            n1014 = Build Array("T-RISE") -> (w1772:string[])
                            n1015 = Build Array(w1770) -> (w1771:dbl[])
                            n1016 = TDMS Write(0:w1768, 5:"TEST PASS", 7:w1772, 9:w1771) -> (15:w1774:errorcluster)  [unwired: 2 in, 3 out]
                            n1017 = local write "data file error"(w1774) -> ()
                          }
                          frame #1 {
                            n1018 = Bundle(cluster=w1775, "STATUS"="T-RISE PASS") -> (w1777:T4)  [unwired: 2 in]
                            n1019 = local write "LAB05-2 (RESULT)"(TRUE) -> ()
                            n1020 = local write "LAB05-2 (DISP)"(w1777) -> ()
                          }
                        }
                      }
                      frame False {
                      }
                    }
                  }
                }
              }
            }
          }
          frame #6 {
            # "disable functions"
            n1021 = stacked-sequence {
              tunnel: w1788 -> [w1798 _ w1848]
              tunnel: w1787 -> [w1797 _ w1847]
              tunnel: w1786 -> [w1796 _ w1846]
              tunnel: w1785 -> [w1795 _ w1845]
              tunnel: w1784 -> [w1794 _ w1844]
              tunnel: w1783 -> [_ w1818 w1843]
              tunnel: w1782 -> [_ w1817 w1842]
              tunnel: w1781 -> [_ w1816 w1841]
              tunnel: w1780 -> [_ w1815 w1840]
              tunnel: w1779 -> [_ w1814 w1839]
              frame #0 {
                n1022 = Select(t=2, s=w1795, f=0) -> (s? t:f=w1790:i32)
                n1023 = Select(t=2, s=w1796, f=0) -> (s? t:f=w1791:i32)
                n1024 = Select(t=2, s=w1794, f=0) -> (s? t:f=w1789:i32)
                n1025 = Select(t=2, s=w1798, f=0) -> (s? t:f=w1793:i32)
                n1026 = Select(t=2, s=w1797, f=0) -> (s? t:f=w1792:i32)
                n1027 = property on="LAB02-2 SELECT" class="RadioBtnsControl (strict)"("DisabledEnum"=w1790) -> ()  [unwired: 2 in, 2 out]
                n1028 = property on="LAB02-1 SELECT" class="RadioBtnsControl (strict)"("DisabledEnum"=w1791) -> ()  [unwired: 2 in, 2 out]
                n1029 = property on="LAB03-1 SELECT" class="RadioBtnsControl (strict)"("DisabledEnum"=w1789) -> ()  [unwired: 2 in, 2 out]
                n1030 = property on="LAB01-1 SELECT" class="RadioBtnsControl (strict)"("DisabledEnum"=w1793) -> ()  [unwired: 2 in, 2 out]
                n1031 = property on="LAB01-2 SELECT" class="RadioBtnsControl (strict)"("DisabledEnum"=w1792) -> ()  [unwired: 2 in, 2 out]
                n1032 = property on="LAB01-2 (RESULT)" class="Bool (strict)"("DisabledEnum"=w1792) -> ()  [unwired: 2 in, 2 out]
                n1033 = property on="LAB02-1 (RESULT)" class="Bool (strict)"("DisabledEnum"=w1791) -> ()  [unwired: 2 in, 2 out]
                n1034 = property on="LAB01-1 (RESULT)" class="Bool (strict)"("DisabledEnum"=w1793) -> ()  [unwired: 2 in, 2 out]
                n1035 = property on="LAB02-2 (RESULT)" class="Bool (strict)"("DisabledEnum"=w1790) -> ()  [unwired: 2 in, 2 out]
                n1036 = property on="LAB03-1 (RESULT)" class="Bool (strict)"("DisabledEnum"=w1789) -> ()  [unwired: 2 in, 2 out]
              }
              frame #1 {
                n1037 = Select(t=2, s=w1814, f=0) -> (s? t:f=w1809:i32)
                n1038 = Select(t=2, s=w1815, f=0) -> (s? t:f=w1810:i32)
                n1039 = Select(t=2, s=w1818, f=0) -> (s? t:f=w1813:i32)
                n1040 = Select(t=2, s=w1817, f=0) -> (s? t:f=w1812:i32)
                n1041 = Select(t=2, s=w1816, f=0) -> (s? t:f=w1811:i32)
                n1042 = property on="LAB05-2 SELECT" class="RadioBtnsControl (strict)"("DisabledEnum"=w1809) -> ()  [unwired: 2 in, 2 out]
                n1043 = property on="LAB05-1 SELECT" class="RadioBtnsControl (strict)"("DisabledEnum"=w1810) -> ()  [unwired: 2 in, 2 out]
                n1044 = property on="LAB03-2 SELECT" class="RadioBtnsControl (strict)"("DisabledEnum"=w1813) -> ()  [unwired: 2 in, 2 out]
                n1045 = property on="LAB04-1 SELECT" class="RadioBtnsControl (strict)"("DisabledEnum"=w1812) -> ()  [unwired: 2 in, 2 out]
                n1046 = property on="LAB04-2 SELECT" class="RadioBtnsControl (strict)"("DisabledEnum"=w1811) -> ()  [unwired: 2 in, 2 out]
                n1047 = property on="LAB03-2 (RESULT)" class="Bool (strict)"("DisabledEnum"=w1813) -> ()  [unwired: 2 in, 2 out]
                n1048 = property on="LAB05-2 (RESULT)" class="Bool (strict)"("DisabledEnum"=w1809) -> ()  [unwired: 2 in, 2 out]
                n1049 = property on="LAB05-1 (RESULT)" class="Bool (strict)"("DisabledEnum"=w1810) -> ()  [unwired: 2 in, 2 out]
                n1050 = property on="LAB04-2 (RESULT)" class="Bool (strict)"("DisabledEnum"=w1811) -> ()  [unwired: 2 in, 2 out]
                n1051 = property on="LAB04-1 (RESULT)" class="Bool (strict)"("DisabledEnum"=w1812) -> ()  [unwired: 2 in, 2 out]
              }
              frame #2 {
                # "disable calibrate if any test running"
                n1052 = Or(x=w1840, y=w1839) -> (x .or. y?=w1833:bool)
                n1053 = Or(x=w1842, y=w1841) -> (x .or. y?=w1835:bool)
                n1054 = Or(x=w1846, y=w1845) -> (x .or. y?=w1837:bool)
                n1055 = Or(x=w1844, y=w1843) -> (x .or. y?=w1836:bool)
                n1056 = Or(x=w1848, y=w1847) -> (x .or. y?=w1838:bool)
                n1057 = Or(x=w1836, y=w1835) -> (x .or. y?=w1834:bool)
                n1058 = Or(x=w1838, y=w1837) -> (x .or. y?=w1832:bool)
                n1059 = Or(x=w1834, y=w1833) -> (x .or. y?=w1831:bool)
                n1060 = Or(x=w1832, y=w1831) -> (x .or. y?=w1830:bool)
                n1061 = case shown="False" w1830 {
                  tunnel: [0 2] -> w1829
                  frame False {
                  }
                  frame True {
                  }
                }
                n1062 = property on="CALIBRATE" class="Bool (strict)"("DisabledEnum"=w1829) -> ()  [unwired: 2 in, 2 out]
              }
            }
          }
          frame #7 {
            # "end test & close test files"
            n1063 = stacked-sequence {
              tunnel: w1859 -> [w1861 _ _ _ _ _ _ _ _ _]
              tunnel: w1860 -> [_ w1874 _ _ _ _ _ _ _ _]
              tunnel: w1858 -> [_ _ w1887 _ _ _ _ _ _ _]
              tunnel: w1857 -> [_ _ _ w1900 _ _ _ _ _ _]
              tunnel: w1856 -> [_ _ _ _ w1913 _ _ _ _ _]
              tunnel: w1855 -> [_ _ _ _ _ w1926 _ _ _ _]
              tunnel: w1854 -> [_ _ _ _ _ _ w1939 _ _ _]
              tunnel: w1853 -> [_ _ _ _ _ _ _ w1952 _ _]
              tunnel: w1852 -> [_ _ _ _ _ _ _ _ w1965 _]
              tunnel: w1851 -> [_ _ _ _ _ _ _ _ _ w1978]
              frame #0 {
                # "LAB01-1"
                n1064 = case shown="True" w1861 {
                  frame False {
                  }
                  frame True {
                    n1065 = local read "LAB01-1 (DISP)"() -> (w1864:T4)
                    n1066 = local read "LAB01-1 (TDMS)"() -> (w1863:refnum<k34>)
                    n1067 = Unbundle(w1864) -> ("STATUS"=w1862:string)  [unwired: 2 out]
                    n1068 = Not Equal?(x=w1862, y="RUN") -> (x != y?=w1865:bool)
                    n1069 = case shown="True" w1865 {
                      tunnel: w1864 -> [_ w1868]
                      tunnel: w1863 -> [_ w1867]
                      frame False {
                      }
                      frame True {
                        n1070 = stacked-sequence {
                          tunnel: w1868 -> [w1870 _]
                          tunnel: w1867 -> [_ w1872]
                          frame #0 {
                            (unwired) "END"
                            n1071 = Bundle(cluster=w1870) -> (w1869:T4)  [unwired: 3 in]
                            n1072 = local write "LAB01-1 (DISP)"(w1869) -> ()
                            n1073 = local write "LAB01-1RUN"(FALSE) -> ()
                          }
                          frame #1 {
                            n1074 = TDMS Close(11:w1872) -> (0:w1873:errorcluster)  [unwired: 1 in, 1 out]
                            n1075 = local write "data file error"(w1873) -> ()
                          }
                        }
                      }
                    }
                  }
                }
              }
              frame #1 {
                # "LAB01-2"
                n1076 = case shown="True" w1874 {
                  frame False {
                  }
                  frame True {
                    n1077 = local read "LAB01-2 (DISP)"() -> (w1876:T4)
                    n1078 = local read "LAB01-2 (TDMS)"() -> (w1875:refnum<k34>)
                    n1079 = Unbundle(w1876) -> ("STATUS"=w1877:string)  [unwired: 2 out]
                    n1080 = Not Equal?(x=w1877, y="RUN") -> (x != y?=w1878:bool)
                    n1081 = case shown="True" w1878 {
                      tunnel: w1876 -> [_ w1881]
                      tunnel: w1875 -> [_ w1880]
                      frame False {
                      }
                      frame True {
                        n1082 = stacked-sequence {
                          tunnel: w1881 -> [w1883 _]
                          tunnel: w1880 -> [_ w1885]
                          frame #0 {
                            (unwired) "END"
                            n1083 = Bundle(cluster=w1883) -> (w1884:T4)  [unwired: 3 in]
                            n1084 = local write "LAB01-2 RUN"(FALSE) -> ()
                            n1085 = local write "LAB01-2 (DISP)"(w1884) -> ()
                          }
                          frame #1 {
                            n1086 = TDMS Close(11:w1885) -> (0:w1886:errorcluster)  [unwired: 1 in, 1 out]
                            n1087 = local write "data file error"(w1886) -> ()
                          }
                        }
                      }
                    }
                  }
                }
              }
              frame #2 {
                # "LAB02-1"
                n1088 = case shown="True" w1887 {
                  frame False {
                  }
                  frame True {
                    n1089 = local read "LAB02-1 (DISP)"() -> (w1889:T4)
                    n1090 = local read "LAB02-1 (TDMS)"() -> (w1888:refnum<k34>)
                    n1091 = Unbundle(w1889) -> ("STATUS"=w1890:string)  [unwired: 2 out]
                    n1092 = Not Equal?(x=w1890, y="RUN") -> (x != y?=w1891:bool)
                    n1093 = case shown="True" w1891 {
                      tunnel: w1889 -> [_ w1894]
                      tunnel: w1888 -> [_ w1893]
                      frame False {
                      }
                      frame True {
                        n1094 = stacked-sequence {
                          tunnel: w1894 -> [w1896 _]
                          tunnel: w1893 -> [_ w1898]
                          frame #0 {
                            (unwired) "END"
                            n1095 = Bundle(cluster=w1896) -> (w1897:T4)  [unwired: 3 in]
                            n1096 = local write "LAB02-1 RUN"(FALSE) -> ()
                            n1097 = local write "LAB02-1 (DISP)"(w1897) -> ()
                          }
                          frame #1 {
                            n1098 = TDMS Close(11:w1898) -> (0:w1899:errorcluster)  [unwired: 1 in, 1 out]
                            n1099 = local write "data file error"(w1899) -> ()
                          }
                        }
                      }
                    }
                  }
                }
              }
              frame #3 {
                # "LAB02-2"
                n1100 = case shown="True" w1900 {
                  frame False {
                  }
                  frame True {
                    n1101 = local read "LAB02-2 (DISP)"() -> (w1902:T4)
                    n1102 = local read "LAB02-2 (TDMS)"() -> (w1901:refnum<k34>)
                    n1103 = Unbundle(w1902) -> ("STATUS"=w1903:string)  [unwired: 2 out]
                    n1104 = Not Equal?(x=w1903, y="RUN") -> (x != y?=w1904:bool)
                    n1105 = case shown="True" w1904 {
                      tunnel: w1902 -> [_ w1907]
                      tunnel: w1901 -> [_ w1906]
                      frame False {
                      }
                      frame True {
                        n1106 = stacked-sequence {
                          tunnel: w1907 -> [w1909 _]
                          tunnel: w1906 -> [_ w1911]
                          frame #0 {
                            (unwired) "END"
                            n1107 = Bundle(cluster=w1909) -> (w1910:T4)  [unwired: 3 in]
                            n1108 = local write "LAB02-2 RUN"(FALSE) -> ()
                            n1109 = local write "LAB02-2 (DISP)"(w1910) -> ()
                          }
                          frame #1 {
                            n1110 = TDMS Close(11:w1911) -> (0:w1912:errorcluster)  [unwired: 1 in, 1 out]
                            n1111 = local write "data file error"(w1912) -> ()
                          }
                        }
                      }
                    }
                  }
                }
              }
              frame #4 {
                # "LAB03-1"
                n1112 = case shown="True" w1913 {
                  frame False {
                  }
                  frame True {
                    n1113 = local read "LAB03-1 (DISP)"() -> (w1915:T4)
                    n1114 = local read "LAB03-1 (TDMS)"() -> (w1914:refnum<k34>)
                    n1115 = Unbundle(w1915) -> ("STATUS"=w1916:string)  [unwired: 2 out]
                    n1116 = Not Equal?(x=w1916, y="RUN") -> (x != y?=w1917:bool)
                    n1117 = case shown="True" w1917 {
                      tunnel: w1915 -> [_ w1920]
                      tunnel: w1914 -> [_ w1919]
                      frame False {
                      }
                      frame True {
                        n1118 = stacked-sequence {
                          tunnel: w1920 -> [w1922 _]
                          tunnel: w1919 -> [_ w1924]
                          frame #0 {
                            (unwired) "END"
                            n1119 = Bundle(cluster=w1922) -> (w1923:T4)  [unwired: 3 in]
                            n1120 = local write "LAB03-1 RUN"(FALSE) -> ()
                            n1121 = local write "LAB03-1 (DISP)"(w1923) -> ()
                          }
                          frame #1 {
                            n1122 = TDMS Close(11:w1924) -> (0:w1925:errorcluster)  [unwired: 1 in, 1 out]
                            n1123 = local write "data file error"(w1925) -> ()
                          }
                        }
                      }
                    }
                  }
                }
              }
              frame #5 {
                # "LAB03-2"
                n1124 = case shown="True" w1926 {
                  frame False {
                  }
                  frame True {
                    n1125 = local read "LAB03-2 (DISP)"() -> (w1928:T4)
                    n1126 = local read "LAB03-2 (TDMS)"() -> (w1927:refnum<k34>)
                    n1127 = Unbundle(w1928) -> ("STATUS"=w1929:string)  [unwired: 2 out]
                    n1128 = Not Equal?(x=w1929, y="RUN") -> (x != y?=w1930:bool)
                    n1129 = case shown="True" w1930 {
                      tunnel: w1928 -> [_ w1933]
                      tunnel: w1927 -> [_ w1932]
                      frame False {
                      }
                      frame True {
                        n1130 = stacked-sequence {
                          tunnel: w1933 -> [w1935 _]
                          tunnel: w1932 -> [_ w1937]
                          frame #0 {
                            (unwired) "END"
                            n1131 = Bundle(cluster=w1935) -> (w1936:T4)  [unwired: 3 in]
                            n1132 = local write "LAB03-2 RUN"(FALSE) -> ()
                            n1133 = local write "LAB03-2 (DISP)"(w1936) -> ()
                          }
                          frame #1 {
                            n1134 = TDMS Close(11:w1937) -> (0:w1938:errorcluster)  [unwired: 1 in, 1 out]
                            n1135 = local write "data file error"(w1938) -> ()
                          }
                        }
                      }
                    }
                  }
                }
              }
              frame #6 {
                # "LAB04-1"
                n1136 = case shown="True" w1939 {
                  frame False {
                  }
                  frame True {
                    n1137 = local read "LAB04-1 (DISP)"() -> (w1941:T4)
                    n1138 = local read "LAB04-1 (TDMS)"() -> (w1940:refnum<k34>)
                    n1139 = Unbundle(w1941) -> ("STATUS"=w1942:string)  [unwired: 2 out]
                    n1140 = Not Equal?(x=w1942, y="RUN") -> (x != y?=w1943:bool)
                    n1141 = case shown="True" w1943 {
                      tunnel: w1941 -> [_ w1946]
                      tunnel: w1940 -> [_ w1945]
                      frame False {
                      }
                      frame True {
                        n1142 = stacked-sequence {
                          tunnel: w1946 -> [w1948 _]
                          tunnel: w1945 -> [_ w1950]
                          frame #0 {
                            (unwired) "END"
                            n1143 = Bundle(cluster=w1948) -> (w1949:T4)  [unwired: 3 in]
                            n1144 = local write "LAB04-1 RUN"(FALSE) -> ()
                            n1145 = local write "LAB04-1 (DISP)"(w1949) -> ()
                          }
                          frame #1 {
                            n1146 = TDMS Close(11:w1950) -> (0:w1951:errorcluster)  [unwired: 1 in, 1 out]
                            n1147 = local write "data file error"(w1951) -> ()
                          }
                        }
                      }
                    }
                  }
                }
              }
              frame #7 {
                # "LAB04-2"
                n1148 = case shown="True" w1952 {
                  frame False {
                  }
                  frame True {
                    n1149 = local read "LAB04-2 (DISP)"() -> (w1954:T4)
                    n1150 = local read "LAB04-2 (TDMS)"() -> (w1953:refnum<k34>)
                    n1151 = Unbundle(w1954) -> ("STATUS"=w1955:string)  [unwired: 2 out]
                    n1152 = Not Equal?(x=w1955, y="RUN") -> (x != y?=w1956:bool)
                    n1153 = case shown="True" w1956 {
                      tunnel: w1954 -> [_ w1959]
                      tunnel: w1953 -> [_ w1958]
                      frame False {
                      }
                      frame True {
                        n1154 = stacked-sequence {
                          tunnel: w1959 -> [w1961 _]
                          tunnel: w1958 -> [_ w1963]
                          frame #0 {
                            (unwired) "END"
                            n1155 = Bundle(cluster=w1961) -> (w1962:T4)  [unwired: 3 in]
                            n1156 = local write "LAB04-2 RUN"(FALSE) -> ()
                            n1157 = local write "LAB04-2 (DISP)"(w1962) -> ()
                          }
                          frame #1 {
                            n1158 = TDMS Close(11:w1963) -> (0:w1964:errorcluster)  [unwired: 1 in, 1 out]
                            n1159 = local write "data file error"(w1964) -> ()
                          }
                        }
                      }
                    }
                  }
                }
              }
              frame #8 {
                # "LAB05-1"
                n1160 = case shown="True" w1965 {
                  frame False {
                  }
                  frame True {
                    n1161 = local read "LAB05-1 (DISP)"() -> (w1967:T4)
                    n1162 = local read "LAB05-1 (TDMS)"() -> (w1966:refnum<k34>)
                    n1163 = Unbundle(w1967) -> ("STATUS"=w1968:string)  [unwired: 2 out]
                    n1164 = Not Equal?(x=w1968, y="RUN") -> (x != y?=w1969:bool)
                    n1165 = case shown="True" w1969 {
                      tunnel: w1967 -> [_ w1972]
                      tunnel: w1966 -> [_ w1971]
                      frame False {
                      }
                      frame True {
                        n1166 = stacked-sequence {
                          tunnel: w1972 -> [w1974 _]
                          tunnel: w1971 -> [_ w1976]
                          frame #0 {
                            (unwired) "END"
                            n1167 = Bundle(cluster=w1974) -> (w1975:T4)  [unwired: 3 in]
                            n1168 = local write "LAB05-1 RUN"(FALSE) -> ()
                            n1169 = local write "LAB05-1 (DISP)"(w1975) -> ()
                          }
                          frame #1 {
                            n1170 = TDMS Close(11:w1976) -> (0:w1977:errorcluster)  [unwired: 1 in, 1 out]
                            n1171 = local write "data file error"(w1977) -> ()
                          }
                        }
                      }
                    }
                  }
                }
              }
              frame #9 {
                # "LAB05-2"
                n1172 = case shown="True" w1978 {
                  frame False {
                  }
                  frame True {
                    n1173 = local read "LAB05-2 (DISP)"() -> (w1980:T4)
                    n1174 = local read "LAB05-2 (TDMS)"() -> (w1979:refnum<k34>)
                    n1175 = Unbundle(w1980) -> ("STATUS"=w1981:string)  [unwired: 2 out]
                    n1176 = Not Equal?(x=w1981, y="RUN") -> (x != y?=w1982:bool)
                    n1177 = case shown="True" w1982 {
                      tunnel: w1980 -> [_ w1985]
                      tunnel: w1979 -> [_ w1984]
                      frame False {
                      }
                      frame True {
                        n1178 = stacked-sequence {
                          tunnel: w1985 -> [w1987 _]
                          tunnel: w1984 -> [_ w1989]
                          frame #0 {
                            (unwired) "END"
                            n1179 = Bundle(cluster=w1987) -> (w1988:T4)  [unwired: 3 in]
                            n1180 = local write "LAB05-2 RUN"(FALSE) -> ()
                            n1181 = local write "LAB05-2 (DISP)"(w1988) -> ()
                          }
                          frame #1 {
                            n1182 = TDMS Close(11:w1989) -> (0:w1990:errorcluster)  [unwired: 1 in, 1 out]
                            n1183 = local write "data file error"(w1990) -> ()
                          }
                        }
                      }
                    }
                  }
                }
              }
            }
          }
          frame #8 {
            # "drive jigs"
            n1184 = stacked-sequence {
              frame #0 {
                # "jig on"
                n1185 = local read "jig cycle"() -> (w1991:dbl)
                n1186 = Equal?(x=w1991, y=0) -> (x = y?=w1993:bool)
                n1187 = case shown="True" w1993 {
                  frame False {
                  }
                  frame True {
                    n1188 = local read "LAB01-1RUN"() -> (w1994:bool)
                    n1189 = local read "LAB01-2 RUN"() -> (w1995:bool)
                    n1190 = local read "LAB03-1 RUN"() -> (w2001:bool)
                    n1191 = local read "LAB03-2 RUN"() -> (w2000:bool)
                    n1192 = local read "LAB02-1 RUN"() -> (w2003:bool)
                    n1193 = local read "LAB02-2 RUN"() -> (w2002:bool)
                    n1194 = local read "LAB04-1 RUN"() -> (w1999:bool)
                    n1195 = local read "LAB04-2 RUN"() -> (w1998:bool)
                    n1196 = local read "LAB05-1 RUN"() -> (w1997:bool)
                    n1197 = local read "LAB05-2 RUN"() -> (w1996:bool)
                    n1198 = local write "LAB05-1 (JIG)"(w1997) -> ()
                    n1199 = local write "LAB05-2 (JIG)"(w1996) -> ()
                    n1200 = local write "LAB04-2 (JIG)"(w1998) -> ()
                    n1201 = local write "LAB02-1 (JIG)"(w2003) -> ()
                    n1202 = local write "LAB03-1 (JIG)"(w2001) -> ()
                    n1203 = local write "LAB04-1 (JIG)"(w1999) -> ()
                    n1204 = local write "LAB03-2 (JIG)"(w2000) -> ()
                    n1205 = local write "LAB02-2 (JIG)"(w2002) -> ()
                    n1206 = local write "LAB01-1 (JIG)"(w1994) -> ()
                    n1207 = local write "LAB01-2 (JIG)"(w1995) -> ()
                  }
                }
              }
              frame #1 {
                # "jig off"
                n1208 = local read "jig cycle"() -> (w2006:dbl)
                n1209 = local read "on loops"() -> (w2005:dbl)
                n1210 = Equal?(x=w2006, y=w2005) -> (x = y?=w2004:bool)
                n1211 = case shown="True" w2004 {
                  frame False {
                  }
                  frame True {
                    w2057 = FALSE
                    w2058 = TRUE
                    w2056 = 2
                    n1212 = local read "LAB05-2 SELECT"() -> (w2047:T3)
                    n1213 = local read "LAB04-2 SELECT"() -> (w2049:T3)
                    n1214 = local read "LAB04-1 SELECT"() -> (w2050:T3)
                    n1215 = local read "LAB05-1 SELECT"() -> (w2048:T3)
                    n1216 = local read "LAB03-2 SELECT"() -> (w2051:T3)
                    n1217 = local read "LAB02-1 SELECT"() -> (w2054:T3)
                    n1218 = local read "LAB03-1 SELECT"() -> (w2052:T3)
                    n1219 = local read "LAB02-2 SELECT"() -> (w2053:T3)
                    n1220 = local read "LAB01-2 SELECT"() -> (w2055:T3)
                    n1221 = local read "LAB05-1 RUN"() -> (w2017:bool)
                    n1222 = local read "LAB05-2 RUN"() -> (w2016:bool)
                    n1223 = local read "LAB04-2 RUN"() -> (w2018:bool)
                    n1224 = local read "LAB04-1 RUN"() -> (w2019:bool)
                    n1225 = local read "LAB01-2 RUN"() -> (w2024:bool)
                    n1226 = local read "LAB03-2 RUN"() -> (w2020:bool)
                    n1227 = local read "LAB01-1RUN"() -> (w2035:bool)
                    n1228 = local read "LAB01-1 SELECT"() -> (w2059:T3)
                    n1229 = local read "LAB03-1 RUN"() -> (w2021:bool)
                    n1230 = local read "LAB02-1 RUN"() -> (w2023:bool)
                    n1231 = local read "LAB02-2 RUN"() -> (w2022:bool)
                    n1232 = Equal?(x=w2056, y=w2052) -> (x = y?=w2030:bool)
                    n1233 = Equal?(x=w2056, y=w2051) -> (x = y?=w2029:bool)
                    n1234 = Equal?(x=w2056, y=w2050) -> (x = y?=w2028:bool)
                    n1235 = Equal?(x=w2056, y=w2049) -> (x = y?=w2027:bool)
                    n1236 = Equal?(x=w2056, y=w2048) -> (x = y?=w2026:bool)
                    n1237 = Equal?(x=w2056, y=w2047) -> (x = y?=w2025:bool)
                    n1238 = Equal?(x=w2056, y=w2059) -> (x = y?=w2036:bool)
                    n1239 = Equal?(x=w2056, y=w2054) -> (x = y?=w2032:bool)
                    n1240 = Equal?(x=w2056, y=w2053) -> (x = y?=w2031:bool)
                    n1241 = Equal?(x=w2056, y=w2055) -> (x = y?=w2033:bool)
                    n1242 = And(x=w2027, y=w2018) -> (x .and. y?=w2009:bool)
                    n1243 = And(x=w2030, y=w2021) -> (x .and. y?=w2012:bool)
                    n1244 = And(x=w2028, y=w2019) -> (x .and. y?=w2010:bool)
                    n1245 = And(x=w2025, y=w2016) -> (x .and. y?=w2007:bool)
                    n1246 = And(x=w2031, y=w2022) -> (x .and. y?=w2013:bool)
                    n1247 = And(x=w2029, y=w2020) -> (x .and. y?=w2011:bool)
                    n1248 = And(x=w2026, y=w2017) -> (x .and. y?=w2008:bool)
                    n1249 = And(x=w2033, y=w2024) -> (x .and. y?=w2015:bool)
                    n1250 = And(x=w2036, y=w2035) -> (x .and. y?=w2034:bool)
                    n1251 = And(x=w2032, y=w2023) -> (x .and. y?=w2014:bool)
                    n1252 = Select(t=w2058, s=w2034, f=w2057) -> (s? t:f=w2037:bool)
                    n1253 = Select(t=w2058, s=w2015, f=w2057) -> (s? t:f=w2038:bool)
                    n1254 = Select(t=w2058, s=w2014, f=w2057) -> (s? t:f=w2039:bool)
                    n1255 = Select(t=w2058, s=w2013, f=w2057) -> (s? t:f=w2040:bool)
                    n1256 = Select(t=w2058, s=w2012, f=w2057) -> (s? t:f=w2041:bool)
                    n1257 = Select(t=w2058, s=w2011, f=w2057) -> (s? t:f=w2042:bool)
                    n1258 = Select(t=w2058, s=w2010, f=w2057) -> (s? t:f=w2043:bool)
                    n1259 = Select(t=w2058, s=w2009, f=w2057) -> (s? t:f=w2044:bool)
                    n1260 = Select(t=w2058, s=w2008, f=w2057) -> (s? t:f=w2045:bool)
                    n1261 = Select(t=w2058, s=w2007, f=w2057) -> (s? t:f=w2046:bool)
                    n1262 = local write "LAB03-2 (JIG)"(w2042) -> ()
                    n1263 = local write "LAB02-1 (JIG)"(w2039) -> ()
                    n1264 = local write "LAB02-2 (JIG)"(w2040) -> ()
                    n1265 = local write "LAB01-2 (JIG)"(w2038) -> ()
                    n1266 = local write "LAB03-1 (JIG)"(w2041) -> ()
                    n1267 = local write "LAB01-1 (JIG)"(w2037) -> ()
                    n1268 = local write "LAB05-2 (JIG)"(w2046) -> ()
                    n1269 = local write "LAB04-1 (JIG)"(w2043) -> ()
                    n1270 = local write "LAB05-1 (JIG)"(w2045) -> ()
                    n1271 = local write "LAB04-2 (JIG)"(w2044) -> ()
                  }
                }
              }
            }
          }
          frame #9 {
            # "drive digital output"
            n1272 = local read "LAB05-2 (O/I)"() -> (w2065:bool)
            n1273 = local read "LAB05-2 (JIG)"() -> (w2064:bool)
            n1274 = local read "LAB05-1 (O/I)"() -> (w2067:bool)
            n1275 = local read "LAB05-1 (JIG)"() -> (w2066:bool)
            n1276 = local read "LAB04-2 (O/I)"() -> (w2069:bool)
            n1277 = local read "LAB04-2 (JIG)"() -> (w2068:bool)
            n1278 = local read "LAB03-1 (O/I)"() -> (w2074:bool)
            n1279 = local read "LAB04-1 (O/I)"() -> (w2070:bool)
            n1280 = local read "LAB04-1 (JIG)"() -> (w2063:bool)
            n1281 = local read "LAB02-1 (O/I)"() -> (w2078:bool)
            n1282 = local read "LAB02-2 (O/I)"() -> (w2076:bool)
            n1283 = local read "LAB03-2 (O/I)"() -> (w2072:bool)
            n1284 = local read "LAB03-2 (JIG)"() -> (w2071:bool)
            n1285 = local read "LAB02-1 (JIG)"() -> (w2077:bool)
            n1286 = local read "LAB02-2 (JIG)"() -> (w2075:bool)
            n1287 = local read "LAB03-1 (JIG)"() -> (w2073:bool)
            n1288 = local read "LAB01-2 (O/I)"() -> (w2080:bool)
            n1289 = local read "LAB01-2 (JIG)"() -> (w2079:bool)
            n1290 = local read "LAB01-1 (O/I)"() -> (w2082:bool)
            n1291 = local read "LAB01-1 (JIG)"() -> (w2081:bool)
            n1292 = Build Array(w2069, w2068, w2067, w2066, w2065, w2064) -> (w2060:bool[])
            n1293 = Build Array(w2075, w2074, w2073, w2072, w2071, w2070, w2063) -> (w2061:bool[])
            n1294 = Build Array(w2082, w2081, w2080, w2079, w2078, w2077, w2076) -> (w2062:bool[])
            n1295 = call "sub vi - Drive Relays All v6.vi"("Array #2"=w2060, "Array #1"=w2061, "Array #0"=w2062) -> ()  [unwired: 8 in, 1 out]
          }
          frame #10 {
            # "get temperature values"
            n1296 = stacked-sequence {
              frame #0 {
                n1297 = local read "jig cycle"() -> (w2083:dbl)
                n1298 = local read "on loops"() -> (w2086:dbl)
                n1299 = local read "jig cycle"() -> (w2088:dbl)
                n1300 = Add(x=w2086, y=2) -> (x+y=w2087:dbl)
                n1301 = Equal?(x=w2088, y=0) -> (x = y?=w2089:bool)
                n1302 = Equal?(x=w2083, y=w2087) -> (x = y?=w2084:bool)
                n1303 = case shown="True" w2089 {
                  frame False {
                  }
                  frame True {
                    w2101 = FALSE
                    w2102 = TRUE
                    n1304 = local write "TEMP update"(TRUE) -> ()
                    n1305 = call "sub vi - GET ALL TEMP v3.vi"("LA01-EN"=w2102, "LA02-EN"=w2102, "LA03-EN"=w2102, "LA04-EN"=w2101, "LA05-EN"=w2101, "Gen Cal Value"=1.0) -> ("LA01 TEMP"=w2100:T15, "LA02 TEMP"=w2098:T15, "LA03 TEMP"=w2097:T15)  [unwired: 4 in, 3 out]
                    n1306 = local write "LAB03 TEMP"(w2097) -> ()
                    n1307 = local write "LAB02 TEMP"(w2098) -> ()
                    n1308 = local write "LAB01 TEMP"(w2100) -> ()
                  }
                }
                n1309 = case shown="True" w2084 {
                  frame False {
                  }
                  frame True {
                    w2094 = TRUE
                    w2095 = FALSE
                    n1310 = local write "TEMP update"(TRUE) -> ()
                    n1311 = call "sub vi - GET ALL TEMP v3.vi"("LA01-EN"=w2095, "LA02-EN"=w2095, "LA03-EN"=w2095, "LA04-EN"=w2094, "LA05-EN"=w2094, "Gen Cal Value"=1.0) -> ("LA04 TEMP"=w2092:T15, "LA05 TEMP"=w2091:T15)  [unwired: 4 in, 4 out]
                    n1312 = local write "LAB04 TEMP"(w2092) -> ()
                    n1313 = local write "LAB05 TEMP"(w2091) -> ()
                  }
                }
              }
              frame #1 {
                n1314 = local read "LAB01 (CAL)"() -> (w2120:T6)
                n1315 = local read "LAB01 TEMP"() -> (w2121:T9)
                n1316 = Unbundle By Name(w2121) -> ("T1 Live"=w2111:dbl, "T1 Neut"=w2110:dbl, "T2 Live"=w2109:dbl, "T2 Neut"=w2108:dbl)  [unwired: 2 out]
                n1317 = Unbundle By Name(w2120) -> ("1 (TL) cal"=w2107:dbl, "1 (TN) cal"=w2106:dbl, "2 (TL) cal"=w2105:dbl, "2 (TN) cal"=w2104:dbl)  [unwired: 6 out]
                n1318 = Multiply(x=w2111, y=w2107) -> (x*y=w2117:dbl)
                n1319 = Multiply(x=w2110, y=w2106) -> (x*y=w2116:dbl)
                n1320 = Multiply(x=w2109, y=w2105) -> (x*y=w2113:dbl)
                n1321 = Multiply(x=w2108, y=w2104) -> (x*y=w2112:dbl)
                n1322 = local read "LAB01-2 (SIG)"() -> (w2115:T2)
                n1323 = local read "LAB01-1 (SIG)"() -> (w2119:T2)
                n1324 = Bundle By Name(cluster=w2119, "Tmp Live"=w2117, "Tmp Neut"=w2116) -> (w2118:T2)
                n1325 = Bundle By Name(cluster=w2115, "Tmp Live"=w2113, "Tmp Neut"=w2112) -> (w2114:T2)
                n1326 = local write "LAB01-1 (SIG)"(w2118) -> ()
                n1327 = local write "LAB01-2 (SIG)"(w2114) -> ()
              }
              frame #2 {
                n1328 = local read "LAB02 (CAL)"() -> (w2138:T7)
                n1329 = local read "LAB02 TEMP"() -> (w2139:T9)
                n1330 = Unbundle By Name(w2139) -> ("T1 Live"=w2129:dbl, "T1 Neut"=w2128:dbl, "T2 Live"=w2127:dbl, "T2 Neut"=w2126:dbl)  [unwired: 2 out]
                n1331 = Unbundle By Name(w2138) -> ("1 (TL) cal"=w2125:dbl, "1 (TN) cal"=w2124:dbl, "2 (TL) cal"=w2123:dbl, "2 (TN) cal"=w2122:dbl)  [unwired: 6 out]
                n1332 = Multiply(x=w2129, y=w2125) -> (x*y=w2135:dbl)
                n1333 = Multiply(x=w2128, y=w2124) -> (x*y=w2134:dbl)
                n1334 = Multiply(x=w2127, y=w2123) -> (x*y=w2131:dbl)
                n1335 = Multiply(x=w2126, y=w2122) -> (x*y=w2130:dbl)
                n1336 = local read "LAB02-2 (SIG)"() -> (w2133:T2)
                n1337 = local read "LAB02-1 (SIG)"() -> (w2137:T2)
                n1338 = Bundle By Name(cluster=w2137, "Tmp Live"=w2135, "Tmp Neut"=w2134) -> (w2136:T2)
                n1339 = Bundle By Name(cluster=w2133, "Tmp Live"=w2131, "Tmp Neut"=w2130) -> (w2132:T2)
                n1340 = local write "LAB02-1 (SIG)"(w2136) -> ()
                n1341 = local write "LAB02-2 (SIG)"(w2132) -> ()
              }
              frame #3 {
                n1342 = local read "LAB03 (CAL)"() -> (w2156:T6)
                n1343 = local read "LAB03 TEMP"() -> (w2157:T9)
                n1344 = Unbundle By Name(w2157) -> ("T1 Live"=w2147:dbl, "T1 Neut"=w2146:dbl, "T2 Live"=w2145:dbl, "T2 Neut"=w2144:dbl)  [unwired: 2 out]
                n1345 = Unbundle By Name(w2156) -> ("1 (TL) cal"=w2143:dbl, "1 (TN) cal"=w2142:dbl, "2 (TL) cal"=w2141:dbl, "2 (TN) cal"=w2140:dbl)  [unwired: 6 out]
                n1346 = Multiply(x=w2147, y=w2143) -> (x*y=w2153:dbl)
                n1347 = Multiply(x=w2146, y=w2142) -> (x*y=w2152:dbl)
                n1348 = Multiply(x=w2145, y=w2141) -> (x*y=w2149:dbl)
                n1349 = Multiply(x=w2144, y=w2140) -> (x*y=w2148:dbl)
                n1350 = local read "LAB03-2 (SIG)"() -> (w2151:T2)
                n1351 = local read "LAB03-1 (SIG)"() -> (w2155:T2)
                n1352 = Bundle By Name(cluster=w2155, "Tmp Live"=w2153, "Tmp Neut"=w2152) -> (w2154:T2)
                n1353 = Bundle By Name(cluster=w2151, "Tmp Live"=w2149, "Tmp Neut"=w2148) -> (w2150:T2)
                n1354 = local write "LAB03-1 (SIG)"(w2154) -> ()
                n1355 = local write "LAB03-2 (SIG)"(w2150) -> ()
              }
              frame #4 {
                n1356 = local read "LAB04 (CAL)"() -> (w2174:T6)
                n1357 = local read "LAB04 TEMP"() -> (w2175:T9)
                n1358 = Unbundle By Name(w2175) -> ("T1 Live"=w2165:dbl, "T1 Neut"=w2164:dbl, "T2 Live"=w2163:dbl, "T2 Neut"=w2162:dbl)  [unwired: 2 out]
                n1359 = Unbundle By Name(w2174) -> ("1 (TL) cal"=w2161:dbl, "1 (TN) cal"=w2160:dbl, "2 (TL) cal"=w2159:dbl, "2 (TN) cal"=w2158:dbl)  [unwired: 6 out]
                n1360 = Multiply(x=w2165, y=w2161) -> (x*y=w2171:dbl)
                n1361 = Multiply(x=w2164, y=w2160) -> (x*y=w2170:dbl)
                n1362 = Multiply(x=w2163, y=w2159) -> (x*y=w2167:dbl)
                n1363 = Multiply(x=w2162, y=w2158) -> (x*y=w2166:dbl)
                n1364 = local read "LAB04-2 (SIG)"() -> (w2169:T2)
                n1365 = local read "LAB04-1 (SIG)"() -> (w2173:T2)
                n1366 = Bundle By Name(cluster=w2173, "Tmp Live"=w2171, "Tmp Neut"=w2170) -> (w2172:T2)
                n1367 = Bundle By Name(cluster=w2169, "Tmp Live"=w2167, "Tmp Neut"=w2166) -> (w2168:T2)
                n1368 = local write "LAB04-1 (SIG)"(w2172) -> ()
                n1369 = local write "LAB04-2 (SIG)"(w2168) -> ()
              }
              frame #5 {
                n1370 = local read "LAB05 (CAL)"() -> (w2192:T6)
                n1371 = local read "LAB05 TEMP"() -> (w2193:T9)
                n1372 = Unbundle By Name(w2193) -> ("T1 Live"=w2183:dbl, "T1 Neut"=w2182:dbl, "T2 Live"=w2181:dbl, "T2 Neut"=w2180:dbl)  [unwired: 2 out]
                n1373 = Unbundle By Name(w2192) -> ("1 (TL) cal"=w2179:dbl, "1 (TN) cal"=w2178:dbl, "2 (TL) cal"=w2177:dbl, "2 (TN) cal"=w2176:dbl)  [unwired: 6 out]
                n1374 = Multiply(x=w2183, y=w2179) -> (x*y=w2189:dbl)
                n1375 = Multiply(x=w2182, y=w2178) -> (x*y=w2188:dbl)
                n1376 = Multiply(x=w2181, y=w2177) -> (x*y=w2185:dbl)
                n1377 = Multiply(x=w2180, y=w2176) -> (x*y=w2184:dbl)
                n1378 = local read "LAB05-2 (SIG)"() -> (w2187:T2)
                n1379 = local read "LAB05-1 (SIG)"() -> (w2191:T2)
                n1380 = Bundle By Name(cluster=w2191, "Tmp Live"=w2189, "Tmp Neut"=w2188) -> (w2190:T2)
                n1381 = Bundle By Name(cluster=w2187, "Tmp Live"=w2185, "Tmp Neut"=w2184) -> (w2186:T2)
                n1382 = local write "LAB05-1 (SIG)"(w2190) -> ()
                n1383 = local write "LAB05-2 (SIG)"(w2186) -> ()
              }
            }
          }
          frame #11 {
            # "get analog values"
            n1384 = local read "on loops"() -> (w2200:dbl)
            n1385 = local read "jig cycle"() -> (w2197:dbl)
            n1386 = Add(x=w2200, y=1) -> (x+y=w2198:dbl)
            n1387 = Equal?(x=w2197, y=1) -> (x = y?=w2195:bool)
            n1388 = Equal?(x=w2197, y=w2198) -> (x = y?=w2196:bool)
            n1389 = Or(x=w2195, y=w2196) -> (x .or. y?=w2194:bool)
            n1390 = case shown="True" w2194 {
              frame False {
              }
              frame True {
                n1391 = call "sub vi - Read Analog All v8.vi"() -> ("Analog loop time"=w2208:dbl, "array GRAPH"=w2207:dynamicdata[], "LAB01"=w2206:T16, "LAB02"=w2205:T17, "LAB03"=w2204:T18, "LAB04"=w2203:T19, "array ERROR"=w2209:errorcluster[], "LAB05"=w2202:T20)  [unwired: 8 in]
                n1392 = stacked-sequence {
                  tunnel: w2209 -> [w2212 _ _ _ _ _]
                  tunnel: w2208 -> [w2211 _ _ _ _ _]
                  tunnel: w2207 -> [w2210 _ _ _ _ _]
                  tunnel: w2206 -> [_ w2257 _ _ _ _]
                  tunnel: w2205 -> [_ _ w2258 _ _ _]
                  tunnel: w2204 -> [_ _ _ w2282 _ _]
                  tunnel: w2203 -> [_ _ _ _ w2306 _]
                  tunnel: w2202 -> [_ _ _ _ _ w2330]
                  frame #0 {
                    n1393 = local write "AI update"(TRUE) -> ()
                    n1394 = Index Array(array=w2210, index=6) -> (element=→"LAB04-1 (GRAPH)":dynamicdata)
                    n1395 = Index Array(array=w2210, index=7) -> (element=→"LAB04-2 (GRAPH)":dynamicdata)
                    n1396 = Index Array(array=w2210, index=9) -> (element=→"LAB05-2 (GRAPH)":dynamicdata)
                    n1397 = Index Array(array=w2210, index=8) -> (element=→"LAB05-1 (GRAPH)":dynamicdata)
                    n1398 = Index Array(array=w2210, index=5) -> (element=→"LAB03-2 (GRAPH)":dynamicdata)
                    n1399 = Index Array(array=w2210, index=0) -> (element=→"LAB01-1 (GRAPH)":dynamicdata)
                    n1400 = Index Array(array=w2210, index=1) -> (element=→"LAB01-2 (GRAPH)":dynamicdata)
                    n1401 = Index Array(array=w2210, index=2) -> (element=→"LAB02-1 (GRAPH)":dynamicdata)
                    n1402 = Index Array(array=w2210, index=3) -> (element=→"LAB02-2 (GRAPH)":dynamicdata)
                    n1403 = Index Array(array=w2210, index=4) -> (element=→"LAB03-1 (GRAPH)":dynamicdata)
                    "AI loop time" <- w2211
                    "Analog Error Array" <- w2212
                  }
                  frame #1 {
                    n1404 = local read "LAB01 (CAL)"() -> (w2256:T6)
                    n1405 = Unbundle By Name(w2257) -> ("LAB01-1 (A)"=w2255:dbl, "LAB01-1 (V)"=w2254:dbl, "LAB01-1 (PF)"=w2253:dbl, "LAB01-2 (A)"=w2252:dbl, "LAB01-2 (V)"=w2251:dbl, "LAB01-2 (PF)"=w2250:dbl)
                    n1406 = Unbundle By Name(w2256) -> ("1  (A) cal"=w2249:dbl, "1 (V) cal"=w2248:dbl, "1 (PF) cal"=w2247:dbl, "2 (A) cal"=w2246:dbl, "2 (V) cal"=w2245:dbl, "2 (PF) cal"=w2244:dbl)  [unwired: 4 out]
                    n1407 = Multiply(x=w2255, y=w2249) -> (x*y=w2242:dbl)
                    n1408 = Multiply(x=w2254, y=w2248) -> (x*y=w2241:dbl)
                    n1409 = Multiply(x=w2253, y=w2247) -> (x*y=w2240:dbl)
                    n1410 = Multiply(x=w2252, y=w2246) -> (x*y=w2236:dbl)
                    n1411 = local read "LAB01-1 (SIG)"() -> (w2243:T2)
                    n1412 = Multiply(x=w2251, y=w2245) -> (x*y=w2235:dbl)
                    n1413 = Multiply(x=w2250, y=w2244) -> (x*y=w2234:dbl)
                    n1414 = local read "LAB01-2 (SIG)"() -> (w2238:T2)
                    n1415 = Bundle By Name(cluster=w2243, "AMPS"=w2242, "VOLTS"=w2241, "PF"=w2240) -> (w2239:T2)
                    n1416 = Bundle By Name(cluster=w2238, "AMPS"=w2236, "VOLTS"=w2235, "PF"=w2234) -> (w2237:T2)
                    n1417 = local write "LAB01-2 (SIG)"(w2237) -> ()
                    n1418 = local write "LAB01-1 (SIG)"(w2239) -> ()
                  }
                  frame #2 {
                    n1419 = local read "LAB02 (CAL)"() -> (w2281:T7)
                    n1420 = Unbundle By Name(w2258) -> ("LAB02-1 (A)"=w2280:dbl, "LAB02-1 (V)"=w2279:dbl, "LAB02-1 (PF)"=w2278:dbl, "LAB02-2 (A)"=w2277:dbl, "LAB02-2 (V)"=w2276:dbl, "LAB02-2 (PF)"=w2275:dbl)
                    n1421 = Unbundle By Name(w2281) -> ("1 (A) cal"=w2274:dbl, "1 (V) cal"=w2273:dbl, "1 (PF) cal"=w2272:dbl, "2 (A) cal"=w2271:dbl, "2 (V) cal"=w2270:dbl, "2 (PF) cal"=w2269:dbl)  [unwired: 4 out]
                    n1422 = Multiply(x=w2280, y=w2274) -> (x*y=w2267:dbl)
                    n1423 = Multiply(x=w2279, y=w2273) -> (x*y=w2266:dbl)
                    n1424 = Multiply(x=w2278, y=w2272) -> (x*y=w2265:dbl)
                    n1425 = Multiply(x=w2277, y=w2271) -> (x*y=w2261:dbl)
                    n1426 = local read "LAB02-1 (SIG)"() -> (w2268:T2)
                    n1427 = Multiply(x=w2276, y=w2270) -> (x*y=w2260:dbl)
                    n1428 = Multiply(x=w2275, y=w2269) -> (x*y=w2259:dbl)
                    n1429 = local read "LAB02-2 (SIG)"() -> (w2263:T2)
                    n1430 = Bundle By Name(cluster=w2268, "AMPS"=w2267, "VOLTS"=w2266, "PF"=w2265) -> (w2264:T2)
                    n1431 = Bundle By Name(cluster=w2263, "AMPS"=w2261, "VOLTS"=w2260, "PF"=w2259) -> (w2262:T2)
                    n1432 = local write "LAB02-2 (SIG)"(w2262) -> ()
                    n1433 = local write "LAB02-1 (SIG)"(w2264) -> ()
                  }
                  frame #3 {
                    n1434 = local read "LAB03 (CAL)"() -> (w2305:T6)
                    n1435 = Unbundle By Name(w2282) -> ("LAB03-1 (A)"=w2304:dbl, "LAB03-1 (V)"=w2303:dbl, "LAB03-1 (PF)"=w2302:dbl, "LAB03-2 (A)"=w2301:dbl, "LAB03-2 (V)"=w2300:dbl, "LAB03-2 (PF)"=w2299:dbl)
                    n1436 = Unbundle By Name(w2305) -> ("1  (A) cal"=w2298:dbl, "1 (V) cal"=w2297:dbl, "1 (PF) cal"=w2296:dbl, "2 (A) cal"=w2295:dbl, "2 (V) cal"=w2294:dbl, "2 (PF) cal"=w2293:dbl)  [unwired: 4 out]
                    n1437 = Multiply(x=w2304, y=w2298) -> (x*y=w2291:dbl)
                    n1438 = Multiply(x=w2303, y=w2297) -> (x*y=w2290:dbl)
                    n1439 = Multiply(x=w2302, y=w2296) -> (x*y=w2289:dbl)
                    n1440 = Multiply(x=w2301, y=w2295) -> (x*y=w2285:dbl)
                    n1441 = local read "LAB03-1 (SIG)"() -> (w2292:T2)
                    n1442 = Multiply(x=w2300, y=w2294) -> (x*y=w2284:dbl)
                    n1443 = Multiply(x=w2299, y=w2293) -> (x*y=w2283:dbl)
                    n1444 = local read "LAB03-1 (SIG)"() -> (w2287:T2)
                    n1445 = Bundle By Name(cluster=w2292, "AMPS"=w2291, "VOLTS"=w2290, "PF"=w2289) -> (w2288:T2)
                    n1446 = Bundle By Name(cluster=w2287, "AMPS"=w2285, "VOLTS"=w2284, "PF"=w2283) -> (w2286:T2)
                    n1447 = local write "LAB03-1 (SIG)"(w2286) -> ()
                    n1448 = local write "LAB03-1 (SIG)"(w2288) -> ()
                  }
                  frame #4 {
                    n1449 = local read "LAB04 (CAL)"() -> (w2329:T6)
                    n1450 = Unbundle By Name(w2306) -> ("LAB04-1 (A)"=w2328:dbl, "LAB04-1 (V)"=w2327:dbl, "LAB04-1 (PF)"=w2326:dbl, "LAB04-2 (A)"=w2325:dbl, "LAB04-2 (V)"=w2324:dbl, "LAB04-2 (PF)"=w2323:dbl)
                    n1451 = Unbundle By Name(w2329) -> ("1  (A) cal"=w2322:dbl, "1 (V) cal"=w2321:dbl, "1 (PF) cal"=w2320:dbl, "2 (A) cal"=w2319:dbl, "2 (V) cal"=w2318:dbl, "2 (PF) cal"=w2317:dbl)  [unwired: 4 out]
                    n1452 = Multiply(x=w2328, y=w2322) -> (x*y=w2315:dbl)
                    n1453 = Multiply(x=w2327, y=w2321) -> (x*y=w2314:dbl)
                    n1454 = Multiply(x=w2326, y=w2320) -> (x*y=w2313:dbl)
                    n1455 = Multiply(x=w2325, y=w2319) -> (x*y=w2309:dbl)
                    n1456 = local read "LAB04-1 (SIG)"() -> (w2316:T2)
                    n1457 = Multiply(x=w2324, y=w2318) -> (x*y=w2308:dbl)
                    n1458 = Multiply(x=w2323, y=w2317) -> (x*y=w2307:dbl)
                    n1459 = local read "LAB04-2 (SIG)"() -> (w2311:T2)
                    n1460 = Bundle By Name(cluster=w2316, "AMPS"=w2315, "VOLTS"=w2314, "PF"=w2313) -> (w2312:T2)
                    n1461 = Bundle By Name(cluster=w2311, "AMPS"=w2309, "VOLTS"=w2308, "PF"=w2307) -> (w2310:T2)
                    n1462 = local write "LAB04-2 (SIG)"(w2310) -> ()
                    n1463 = local write "LAB04-1 (SIG)"(w2312) -> ()
                  }
                  frame #5 {
                    n1464 = local read "LAB05 (CAL)"() -> (w2353:T6)
                    n1465 = Unbundle By Name(w2330) -> ("LAB05-1 (A)"=w2352:dbl, "LAB05-1 (V)"=w2351:dbl, "LAB05-1 (PF)"=w2350:dbl, "LAB05-2 (A)"=w2349:dbl, "LAB05-2 (V)"=w2348:dbl, "LAB05-2 (PF)"=w2347:dbl)
                    n1466 = Unbundle By Name(w2353) -> ("1  (A) cal"=w2346:dbl, "1 (V) cal"=w2345:dbl, "1 (PF) cal"=w2344:dbl, "2 (A) cal"=w2343:dbl, "2 (V) cal"=w2342:dbl, "2 (PF) cal"=w2341:dbl)  [unwired: 4 out]
                    n1467 = Multiply(x=w2352, y=w2346) -> (x*y=w2339:dbl)
                    n1468 = Multiply(x=w2351, y=w2345) -> (x*y=w2338:dbl)
                    n1469 = Multiply(x=w2350, y=w2344) -> (x*y=w2337:dbl)
                    n1470 = Multiply(x=w2349, y=w2343) -> (x*y=w2333:dbl)
                    n1471 = local read "LAB05-1 (SIG)"() -> (w2340:T2)
                    n1472 = Multiply(x=w2348, y=w2342) -> (x*y=w2332:dbl)
                    n1473 = Multiply(x=w2347, y=w2341) -> (x*y=w2331:dbl)
                    n1474 = local read "LAB05-2 (SIG)"() -> (w2335:T2)
                    n1475 = Bundle By Name(cluster=w2340, "AMPS"=w2339, "VOLTS"=w2338, "PF"=w2337) -> (w2336:T2)
                    n1476 = Bundle By Name(cluster=w2335, "AMPS"=w2333, "VOLTS"=w2332, "PF"=w2331) -> (w2334:T2)
                    n1477 = local write "LAB05-2 (SIG)"(w2334) -> ()
                    n1478 = local write "LAB05-1 (SIG)"(w2336) -> ()
                  }
                }
              }
            }
          }
          frame #12 {
            # "save test data to file"
            n1479 = local read "on loops"() -> (w2370:dbl)
            n1480 = local read "jig cycle"() -> (w2367:dbl)
            n1481 = Add(x=w2370, y=2) -> (x+y=w2368:dbl)
            n1482 = Equal?(x=w2367, y=1) -> (x = y?=w2365:bool)
            n1483 = Equal?(x=w2367, y=w2368) -> (x = y?=w2366:bool)
            n1484 = Or(x=w2365, y=w2366) -> (x .or. y?=w2364:bool)
            n1485 = case shown="True" w2364 {
              tunnel: w2363 -> [_ w2381]
              tunnel: w2362 -> [_ w2380]
              tunnel: w2361 -> [_ w2379]
              tunnel: w2360 -> [_ w2378]
              tunnel: w2359 -> [_ w2377]
              tunnel: w2358 -> [_ w2376]
              tunnel: w2357 -> [_ w2375]
              tunnel: w2356 -> [_ w2374]
              tunnel: w2355 -> [_ w2373]
              tunnel: w2354 -> [_ w2372]
              frame False {
              }
              frame True {
                n1486 = stacked-sequence {
                  tunnel: w2381 -> [w2382 _ _ _ _ _ _ _ _ _]
                  tunnel: w2380 -> [_ w2427 _ _ _ _ _ _ _ _]
                  tunnel: w2379 -> [_ _ w2472 _ _ _ _ _ _ _]
                  tunnel: w2378 -> [_ _ _ w2517 _ _ _ _ _ _]
                  tunnel: w2377 -> [_ _ _ _ w2562 _ _ _ _ _]
                  tunnel: w2376 -> [_ _ _ _ _ w2607 _ _ _ _]
                  tunnel: w2375 -> [_ _ _ _ _ _ w2652 _ _ _]
                  tunnel: w2374 -> [_ _ _ _ _ _ _ w2697 _ _]
                  tunnel: w2373 -> [_ _ _ _ _ _ _ _ w2742 _]
                  tunnel: w2372 -> [_ _ _ _ _ _ _ _ _ w2787]
                  frame #0 {
                    # "LAB01-1"
                    n1487 = case shown="True" w2382 {
                      frame False {
                      }
                      frame True {
                        n1488 = local read "LAB01-1 (DISP)"() -> (w2424:T4)
                        n1489 = local read "LAB01-1 (SIG)"() -> (w2425:T2)
                        n1490 = local read "LAB01-1 (TDMS)"() -> (w2426:refnum<k34>)
                        n1491 = Build Array("TEMP Neut") -> (w2390:string[])
                        n1492 = Build Array("CYCLE") -> (w2385:string[])
                        n1493 = Build Array("TEMP Live") -> (w2395:string[])
                        n1494 = Build Array("PF") -> (w2400:string[])
                        n1495 = Build Array("AMPS") -> (w2421:string[])
                        n1496 = Build Array("VOLTS") -> (w2412:string[])
                        n1497 = Unbundle(w2425) -> ("AMPS"=w2420:dbl, "VOLTS"=w2409:dbl, "PF"=w2408:dbl, "Tmp Live"=w2407:dbl, "Tmp Neut"=w2410:dbl)
                        n1498 = Unbundle(w2424) -> ("CYCLE"=w2405:dbl)  [unwired: 2 out]
                        n1499 = Build Array(w2409) -> (w2406:dbl[])
                        n1500 = Build Array(w2408) -> (w2399:dbl[])
                        n1501 = Build Array(w2407) -> (w2394:dbl[])
                        n1502 = Build Array(w2410) -> (w2389:dbl[])
                        n1503 = Build Array(w2420) -> (w2419:dbl[])
                        n1504 = Build Array(w2405) -> (w2384:dbl[])
                        n1505 = TDMS Write(0:w2426, 5:"LAB01-1 TEST VALUES", 7:w2421, 9:w2419) -> (4:w2414:refnum<k34>, 6:w2413:string, 15:w2401:errorcluster)  [unwired: 2 in, 1 out]
                        n1506 = TDMS Write(0:w2414, 5:w2413, 7:w2412, 9:w2406, 11:w2401) -> (4:w2404:refnum<k34>, 6:w2403:string, 15:w2402:errorcluster)  [unwired: 1 in, 1 out]
                        n1507 = TDMS Write(0:w2404, 5:w2403, 7:w2400, 9:w2399, 11:w2402) -> (4:w2398:refnum<k34>, 6:w2397:string, 15:w2396:errorcluster)  [unwired: 1 in, 1 out]
                        n1508 = TDMS Write(0:w2398, 5:w2397, 7:w2395, 9:w2394, 11:w2396) -> (4:w2393:refnum<k34>, 6:w2392:string, 15:w2391:errorcluster)  [unwired: 1 in, 1 out]
                        n1509 = TDMS Write(0:w2393, 5:w2392, 7:w2390, 9:w2389, 11:w2391) -> (4:w2388:refnum<k34>, 6:w2387:string, 15:w2386:errorcluster)  [unwired: 1 in, 1 out]
                        n1510 = TDMS Write(0:w2388, 5:w2387, 7:w2385, 9:w2384, 11:w2386) -> (15:w2383:errorcluster)  [unwired: 1 in, 3 out]
                        n1511 = local write "data file error"(w2383) -> ()
                      }
                    }
                  }
                  frame #1 {
                    # "LAB01-2"
                    n1512 = case shown="True" w2427 {
                      frame False {
                      }
                      frame True {
                        n1513 = local read "LAB01-2 (DISP)"() -> (w2469:T4)
                        n1514 = local read "LAB01-2 (SIG)"() -> (w2470:T2)
                        n1515 = local read "LAB01-2 (TDMS)"() -> (w2471:refnum<k34>)
                        n1516 = Build Array("TEMP Neut") -> (w2435:string[])
                        n1517 = Build Array("CYCLE") -> (w2430:string[])
                        n1518 = Build Array("TEMP Live") -> (w2440:string[])
                        n1519 = Build Array("PF") -> (w2445:string[])
                        n1520 = Build Array("AMPS") -> (w2466:string[])
                        n1521 = Build Array("VOLTS") -> (w2457:string[])
                        n1522 = Unbundle(w2470) -> ("AMPS"=w2465:dbl, "VOLTS"=w2454:dbl, "PF"=w2453:dbl, "Tmp Live"=w2452:dbl, "Tmp Neut"=w2455:dbl)
                        n1523 = Unbundle(w2469) -> ("CYCLE"=w2450:dbl)  [unwired: 2 out]
                        n1524 = Build Array(w2454) -> (w2451:dbl[])
                        n1525 = Build Array(w2453) -> (w2444:dbl[])
                        n1526 = Build Array(w2452) -> (w2439:dbl[])
                        n1527 = Build Array(w2455) -> (w2434:dbl[])
                        n1528 = Build Array(w2465) -> (w2464:dbl[])
                        n1529 = Build Array(w2450) -> (w2429:dbl[])
                        n1530 = TDMS Write(0:w2471, 5:"LAB01-2 TEST VALUES", 7:w2466, 9:w2464) -> (4:w2459:refnum<k34>, 6:w2458:string, 15:w2446:errorcluster)  [unwired: 2 in, 1 out]
                        n1531 = TDMS Write(0:w2459, 5:w2458, 7:w2457, 9:w2451, 11:w2446) -> (4:w2449:refnum<k34>, 6:w2448:string, 15:w2447:errorcluster)  [unwired: 1 in, 1 out]
                        n1532 = TDMS Write(0:w2449, 5:w2448, 7:w2445, 9:w2444, 11:w2447) -> (4:w2443:refnum<k34>, 6:w2442:string, 15:w2441:errorcluster)  [unwired: 1 in, 1 out]
                        n1533 = TDMS Write(0:w2443, 5:w2442, 7:w2440, 9:w2439, 11:w2441) -> (4:w2438:refnum<k34>, 6:w2437:string, 15:w2436:errorcluster)  [unwired: 1 in, 1 out]
                        n1534 = TDMS Write(0:w2438, 5:w2437, 7:w2435, 9:w2434, 11:w2436) -> (4:w2433:refnum<k34>, 6:w2432:string, 15:w2431:errorcluster)  [unwired: 1 in, 1 out]
                        n1535 = TDMS Write(0:w2433, 5:w2432, 7:w2430, 9:w2429, 11:w2431) -> (15:w2428:errorcluster)  [unwired: 1 in, 3 out]
                        n1536 = local write "data file error"(w2428) -> ()
                      }
                    }
                  }
                  frame #2 {
                    # "LAB02-1"
                    n1537 = case shown="True" w2472 {
                      frame False {
                      }
                      frame True {
                        n1538 = local read "LAB02-1 (DISP)"() -> (w2514:T4)
                        n1539 = local read "LAB02-1 (SIG)"() -> (w2515:T2)
                        n1540 = local read "LAB02-1 (TDMS)"() -> (w2516:refnum<k34>)
                        n1541 = Build Array("TEMP Neut") -> (w2480:string[])
                        n1542 = Build Array("CYCLE") -> (w2475:string[])
                        n1543 = Build Array("TEMP Live") -> (w2485:string[])
                        n1544 = Build Array("PF") -> (w2490:string[])
                        n1545 = Build Array("AMPS") -> (w2511:string[])
                        n1546 = Build Array("VOLTS") -> (w2502:string[])
                        n1547 = Unbundle(w2515) -> ("AMPS"=w2510:dbl, "VOLTS"=w2499:dbl, "PF"=w2498:dbl, "Tmp Live"=w2497:dbl, "Tmp Neut"=w2500:dbl)
                        n1548 = Unbundle(w2514) -> ("CYCLE"=w2495:dbl)  [unwired: 2 out]
                        n1549 = Build Array(w2499) -> (w2496:dbl[])
                        n1550 = Build Array(w2498) -> (w2489:dbl[])
                        n1551 = Build Array(w2497) -> (w2484:dbl[])
                        n1552 = Build Array(w2500) -> (w2479:dbl[])
                        n1553 = Build Array(w2510) -> (w2509:dbl[])
                        n1554 = Build Array(w2495) -> (w2474:dbl[])
                        n1555 = TDMS Write(0:w2516, 5:"LAB02-1 TEST VALUES", 7:w2511, 9:w2509) -> (4:w2504:refnum<k34>, 6:w2503:string, 15:w2491:errorcluster)  [unwired: 2 in, 1 out]
                        n1556 = TDMS Write(0:w2504, 5:w2503, 7:w2502, 9:w2496, 11:w2491) -> (4:w2494:refnum<k34>, 6:w2493:string, 15:w2492:errorcluster)  [unwired: 1 in, 1 out]
                        n1557 = TDMS Write(0:w2494, 5:w2493, 7:w2490, 9:w2489, 11:w2492) -> (4:w2488:refnum<k34>, 6:w2487:string, 15:w2486:errorcluster)  [unwired: 1 in, 1 out]
                        n1558 = TDMS Write(0:w2488, 5:w2487, 7:w2485, 9:w2484, 11:w2486) -> (4:w2483:refnum<k34>, 6:w2482:string, 15:w2481:errorcluster)  [unwired: 1 in, 1 out]
                        n1559 = TDMS Write(0:w2483, 5:w2482, 7:w2480, 9:w2479, 11:w2481) -> (4:w2478:refnum<k34>, 6:w2477:string, 15:w2476:errorcluster)  [unwired: 1 in, 1 out]
                        n1560 = TDMS Write(0:w2478, 5:w2477, 7:w2475, 9:w2474, 11:w2476) -> (15:w2473:errorcluster)  [unwired: 1 in, 3 out]
                        n1561 = local write "data file error"(w2473) -> ()
                      }
                    }
                  }
                  frame #3 {
                    # "LAB02-2"
                    n1562 = case shown="True" w2517 {
                      frame False {
                      }
                      frame True {
                        n1563 = local read "LAB02-2 (DISP)"() -> (w2559:T4)
                        n1564 = local read "LAB02-2 (SIG)"() -> (w2560:T2)
                        n1565 = local read "LAB02-2 (TDMS)"() -> (w2561:refnum<k34>)
                        n1566 = Build Array("TEMP Neut") -> (w2525:string[])
                        n1567 = Build Array("CYCLE") -> (w2520:string[])
                        n1568 = Build Array("TEMP Live") -> (w2530:string[])
                        n1569 = Build Array("PF") -> (w2535:string[])
                        n1570 = Build Array("AMPS") -> (w2556:string[])
                        n1571 = Build Array("VOLTS") -> (w2547:string[])
                        n1572 = Unbundle(w2560) -> ("AMPS"=w2555:dbl, "VOLTS"=w2544:dbl, "PF"=w2543:dbl, "Tmp Live"=w2542:dbl, "Tmp Neut"=w2545:dbl)
                        n1573 = Unbundle(w2559) -> ("CYCLE"=w2540:dbl)  [unwired: 2 out]
                        n1574 = Build Array(w2544) -> (w2541:dbl[])
                        n1575 = Build Array(w2543) -> (w2534:dbl[])
                        n1576 = Build Array(w2542) -> (w2529:dbl[])
                        n1577 = Build Array(w2545) -> (w2524:dbl[])
                        n1578 = Build Array(w2555) -> (w2554:dbl[])
                        n1579 = Build Array(w2540) -> (w2519:dbl[])
                        n1580 = TDMS Write(0:w2561, 5:"LAB02-2 TEST VALUES", 7:w2556, 9:w2554) -> (4:w2549:refnum<k34>, 6:w2548:string, 15:w2536:errorcluster)  [unwired: 2 in, 1 out]
                        n1581 = TDMS Write(0:w2549, 5:w2548, 7:w2547, 9:w2541, 11:w2536) -> (4:w2539:refnum<k34>, 6:w2538:string, 15:w2537:errorcluster)  [unwired: 1 in, 1 out]
                        n1582 = TDMS Write(0:w2539, 5:w2538, 7:w2535, 9:w2534, 11:w2537) -> (4:w2533:refnum<k34>, 6:w2532:string, 15:w2531:errorcluster)  [unwired: 1 in, 1 out]
                        n1583 = TDMS Write(0:w2533, 5:w2532, 7:w2530, 9:w2529, 11:w2531) -> (4:w2528:refnum<k34>, 6:w2527:string, 15:w2526:errorcluster)  [unwired: 1 in, 1 out]
                        n1584 = TDMS Write(0:w2528, 5:w2527, 7:w2525, 9:w2524, 11:w2526) -> (4:w2523:refnum<k34>, 6:w2522:string, 15:w2521:errorcluster)  [unwired: 1 in, 1 out]
                        n1585 = TDMS Write(0:w2523, 5:w2522, 7:w2520, 9:w2519, 11:w2521) -> (15:w2518:errorcluster)  [unwired: 1 in, 3 out]
                        n1586 = local write "data file error"(w2518) -> ()
                      }
                    }
                  }
                  frame #4 {
                    # "LAB03-1"
                    n1587 = case shown="True" w2562 {
                      frame False {
                      }
                      frame True {
                        n1588 = local read "LAB03-1 (DISP)"() -> (w2604:T4)
                        n1589 = local read "LAB03-1 (SIG)"() -> (w2605:T2)
                        n1590 = local read "LAB03-1 (TDMS)"() -> (w2606:refnum<k34>)
                        n1591 = Build Array("TEMP Neut") -> (w2570:string[])
                        n1592 = Build Array("CYCLE") -> (w2565:string[])
                        n1593 = Build Array("TEMP Live") -> (w2575:string[])
                        n1594 = Build Array("PF") -> (w2580:string[])
                        n1595 = Build Array("AMPS") -> (w2601:string[])
                        n1596 = Build Array("VOLTS") -> (w2592:string[])
                        n1597 = Unbundle(w2605) -> ("AMPS"=w2600:dbl, "VOLTS"=w2589:dbl, "PF"=w2588:dbl, "Tmp Live"=w2587:dbl, "Tmp Neut"=w2590:dbl)
                        n1598 = Unbundle(w2604) -> ("CYCLE"=w2585:dbl)  [unwired: 2 out]
                        n1599 = Build Array(w2589) -> (w2586:dbl[])
                        n1600 = Build Array(w2588) -> (w2579:dbl[])
                        n1601 = Build Array(w2587) -> (w2574:dbl[])
                        n1602 = Build Array(w2590) -> (w2569:dbl[])
                        n1603 = Build Array(w2600) -> (w2599:dbl[])
                        n1604 = Build Array(w2585) -> (w2564:dbl[])
                        n1605 = TDMS Write(0:w2606, 5:"LAB03-1 TEST VALUES", 7:w2601, 9:w2599) -> (4:w2594:refnum<k34>, 6:w2593:string, 15:w2581:errorcluster)  [unwired: 2 in, 1 out]
                        n1606 = TDMS Write(0:w2594, 5:w2593, 7:w2592, 9:w2586, 11:w2581) -> (4:w2584:refnum<k34>, 6:w2583:string, 15:w2582:errorcluster)  [unwired: 1 in, 1 out]
                        n1607 = TDMS Write(0:w2584, 5:w2583, 7:w2580, 9:w2579, 11:w2582) -> (4:w2578:refnum<k34>, 6:w2577:string, 15:w2576:errorcluster)  [unwired: 1 in, 1 out]
                        n1608 = TDMS Write(0:w2578, 5:w2577, 7:w2575, 9:w2574, 11:w2576) -> (4:w2573:refnum<k34>, 6:w2572:string, 15:w2571:errorcluster)  [unwired: 1 in, 1 out]
                        n1609 = TDMS Write(0:w2573, 5:w2572, 7:w2570, 9:w2569, 11:w2571) -> (4:w2568:refnum<k34>, 6:w2567:string, 15:w2566:errorcluster)  [unwired: 1 in, 1 out]
                        n1610 = TDMS Write(0:w2568, 5:w2567, 7:w2565, 9:w2564, 11:w2566) -> (15:w2563:errorcluster)  [unwired: 1 in, 3 out]
                        n1611 = local write "data file error"(w2563) -> ()
                      }
                    }
                  }
                  frame #5 {
                    # "LAB03-2"
                    n1612 = case shown="True" w2607 {
                      frame False {
                      }
                      frame True {
                        n1613 = local read "LAB03-2 (DISP)"() -> (w2649:T4)
                        n1614 = local read "LAB03-2 (SIG)"() -> (w2650:T2)
                        n1615 = local read "LAB03-2 (TDMS)"() -> (w2651:refnum<k34>)
                        n1616 = Build Array("TEMP Neut") -> (w2615:string[])
                        n1617 = Build Array("CYCLE") -> (w2610:string[])
                        n1618 = Build Array("TEMP Live") -> (w2620:string[])
                        n1619 = Build Array("PF") -> (w2625:string[])
                        n1620 = Build Array("AMPS") -> (w2646:string[])
                        n1621 = Build Array("VOLTS") -> (w2637:string[])
                        n1622 = Unbundle(w2650) -> ("AMPS"=w2645:dbl, "VOLTS"=w2634:dbl, "PF"=w2633:dbl, "Tmp Live"=w2632:dbl, "Tmp Neut"=w2635:dbl)
                        n1623 = Unbundle(w2649) -> ("CYCLE"=w2630:dbl)  [unwired: 2 out]
                        n1624 = Build Array(w2634) -> (w2631:dbl[])
                        n1625 = Build Array(w2633) -> (w2624:dbl[])
                        n1626 = Build Array(w2632) -> (w2619:dbl[])
                        n1627 = Build Array(w2635) -> (w2614:dbl[])
                        n1628 = Build Array(w2645) -> (w2644:dbl[])
                        n1629 = Build Array(w2630) -> (w2609:dbl[])
                        n1630 = TDMS Write(0:w2651, 5:"LAB03-2 TEST VALUES", 7:w2646, 9:w2644) -> (4:w2639:refnum<k34>, 6:w2638:string, 15:w2626:errorcluster)  [unwired: 2 in, 1 out]
                        n1631 = TDMS Write(0:w2639, 5:w2638, 7:w2637, 9:w2631, 11:w2626) -> (4:w2629:refnum<k34>, 6:w2628:string, 15:w2627:errorcluster)  [unwired: 1 in, 1 out]
                        n1632 = TDMS Write(0:w2629, 5:w2628, 7:w2625, 9:w2624, 11:w2627) -> (4:w2623:refnum<k34>, 6:w2622:string, 15:w2621:errorcluster)  [unwired: 1 in, 1 out]
                        n1633 = TDMS Write(0:w2623, 5:w2622, 7:w2620, 9:w2619, 11:w2621) -> (4:w2618:refnum<k34>, 6:w2617:string, 15:w2616:errorcluster)  [unwired: 1 in, 1 out]
                        n1634 = TDMS Write(0:w2618, 5:w2617, 7:w2615, 9:w2614, 11:w2616) -> (4:w2613:refnum<k34>, 6:w2612:string, 15:w2611:errorcluster)  [unwired: 1 in, 1 out]
                        n1635 = TDMS Write(0:w2613, 5:w2612, 7:w2610, 9:w2609, 11:w2611) -> (15:w2608:errorcluster)  [unwired: 1 in, 3 out]
                        n1636 = local write "data file error"(w2608) -> ()
                      }
                    }
                  }
                  frame #6 {
                    # "LAB04-1"
                    n1637 = case shown="True" w2652 {
                      frame False {
                      }
                      frame True {
                        n1638 = local read "LAB04-1 (DISP)"() -> (w2694:T4)
                        n1639 = local read "LAB04-1 (SIG)"() -> (w2695:T2)
                        n1640 = local read "LAB04-1 (TDMS)"() -> (w2696:refnum<k34>)
                        n1641 = Build Array("TEMP Neut") -> (w2660:string[])
                        n1642 = Build Array("CYCLE") -> (w2655:string[])
                        n1643 = Build Array("TEMP Live") -> (w2665:string[])
                        n1644 = Build Array("PF") -> (w2670:string[])
                        n1645 = Build Array("AMPS") -> (w2691:string[])
                        n1646 = Build Array("VOLTS") -> (w2682:string[])
                        n1647 = Unbundle(w2695) -> ("AMPS"=w2690:dbl, "VOLTS"=w2679:dbl, "PF"=w2678:dbl, "Tmp Live"=w2677:dbl, "Tmp Neut"=w2680:dbl)
                        n1648 = Unbundle(w2694) -> ("CYCLE"=w2675:dbl)  [unwired: 2 out]
                        n1649 = Build Array(w2679) -> (w2676:dbl[])
                        n1650 = Build Array(w2678) -> (w2669:dbl[])
                        n1651 = Build Array(w2677) -> (w2664:dbl[])
                        n1652 = Build Array(w2680) -> (w2659:dbl[])
                        n1653 = Build Array(w2690) -> (w2689:dbl[])
                        n1654 = Build Array(w2675) -> (w2654:dbl[])
                        n1655 = TDMS Write(0:w2696, 5:"LAB04-1 TEST VALUES", 7:w2691, 9:w2689) -> (4:w2684:refnum<k34>, 6:w2683:string, 15:w2671:errorcluster)  [unwired: 2 in, 1 out]
                        n1656 = TDMS Write(0:w2684, 5:w2683, 7:w2682, 9:w2676, 11:w2671) -> (4:w2674:refnum<k34>, 6:w2673:string, 15:w2672:errorcluster)  [unwired: 1 in, 1 out]
                        n1657 = TDMS Write(0:w2674, 5:w2673, 7:w2670, 9:w2669, 11:w2672) -> (4:w2668:refnum<k34>, 6:w2667:string, 15:w2666:errorcluster)  [unwired: 1 in, 1 out]
                        n1658 = TDMS Write(0:w2668, 5:w2667, 7:w2665, 9:w2664, 11:w2666) -> (4:w2663:refnum<k34>, 6:w2662:string, 15:w2661:errorcluster)  [unwired: 1 in, 1 out]
                        n1659 = TDMS Write(0:w2663, 5:w2662, 7:w2660, 9:w2659, 11:w2661) -> (4:w2658:refnum<k34>, 6:w2657:string, 15:w2656:errorcluster)  [unwired: 1 in, 1 out]
                        n1660 = TDMS Write(0:w2658, 5:w2657, 7:w2655, 9:w2654, 11:w2656) -> (15:w2653:errorcluster)  [unwired: 1 in, 3 out]
                        n1661 = local write "data file error"(w2653) -> ()
                      }
                    }
                  }
                  frame #7 {
                    # "LAB04-2"
                    n1662 = case shown="True" w2697 {
                      frame False {
                      }
                      frame True {
                        n1663 = local read "LAB04-2 (DISP)"() -> (w2739:T4)
                        n1664 = local read "LAB04-2 (SIG)"() -> (w2740:T2)
                        n1665 = local read "LAB04-2 (TDMS)"() -> (w2741:refnum<k34>)
                        n1666 = Build Array("TEMP Neut") -> (w2705:string[])
                        n1667 = Build Array("CYCLE") -> (w2700:string[])
                        n1668 = Build Array("TEMP Live") -> (w2710:string[])
                        n1669 = Build Array("PF") -> (w2715:string[])
                        n1670 = Build Array("AMPS") -> (w2736:string[])
                        n1671 = Build Array("VOLTS") -> (w2727:string[])
                        n1672 = Unbundle(w2740) -> ("AMPS"=w2735:dbl, "VOLTS"=w2724:dbl, "PF"=w2723:dbl, "Tmp Live"=w2722:dbl, "Tmp Neut"=w2725:dbl)
                        n1673 = Unbundle(w2739) -> ("CYCLE"=w2720:dbl)  [unwired: 2 out]
                        n1674 = Build Array(w2724) -> (w2721:dbl[])
                        n1675 = Build Array(w2723) -> (w2714:dbl[])
                        n1676 = Build Array(w2722) -> (w2709:dbl[])
                        n1677 = Build Array(w2725) -> (w2704:dbl[])
                        n1678 = Build Array(w2735) -> (w2734:dbl[])
                        n1679 = Build Array(w2720) -> (w2699:dbl[])
                        n1680 = TDMS Write(0:w2741, 5:"LAB04-2 TEST VALUES", 7:w2736, 9:w2734) -> (4:w2729:refnum<k34>, 6:w2728:string, 15:w2716:errorcluster)  [unwired: 2 in, 1 out]
                        n1681 = TDMS Write(0:w2729, 5:w2728, 7:w2727, 9:w2721, 11:w2716) -> (4:w2719:refnum<k34>, 6:w2718:string, 15:w2717:errorcluster)  [unwired: 1 in, 1 out]
                        n1682 = TDMS Write(0:w2719, 5:w2718, 7:w2715, 9:w2714, 11:w2717) -> (4:w2713:refnum<k34>, 6:w2712:string, 15:w2711:errorcluster)  [unwired: 1 in, 1 out]
                        n1683 = TDMS Write(0:w2713, 5:w2712, 7:w2710, 9:w2709, 11:w2711) -> (4:w2708:refnum<k34>, 6:w2707:string, 15:w2706:errorcluster)  [unwired: 1 in, 1 out]
                        n1684 = TDMS Write(0:w2708, 5:w2707, 7:w2705, 9:w2704, 11:w2706) -> (4:w2703:refnum<k34>, 6:w2702:string, 15:w2701:errorcluster)  [unwired: 1 in, 1 out]
                        n1685 = TDMS Write(0:w2703, 5:w2702, 7:w2700, 9:w2699, 11:w2701) -> (15:w2698:errorcluster)  [unwired: 1 in, 3 out]
                        n1686 = local write "data file error"(w2698) -> ()
                      }
                    }
                  }
                  frame #8 {
                    # "LAB05-1"
                    n1687 = case shown="True" w2742 {
                      frame False {
                      }
                      frame True {
                        n1688 = local read "LAB05-1 (DISP)"() -> (w2784:T4)
                        n1689 = local read "LAB05-1 (SIG)"() -> (w2785:T2)
                        n1690 = local read "LAB05-1 (TDMS)"() -> (w2786:refnum<k34>)
                        n1691 = Build Array("TEMP Neut") -> (w2750:string[])
                        n1692 = Build Array("CYCLE") -> (w2745:string[])
                        n1693 = Build Array("TEMP Live") -> (w2755:string[])
                        n1694 = Build Array("PF") -> (w2760:string[])
                        n1695 = Build Array("AMPS") -> (w2781:string[])
                        n1696 = Build Array("VOLTS") -> (w2772:string[])
                        n1697 = Unbundle(w2785) -> ("AMPS"=w2780:dbl, "VOLTS"=w2769:dbl, "PF"=w2768:dbl, "Tmp Live"=w2767:dbl, "Tmp Neut"=w2770:dbl)
                        n1698 = Unbundle(w2784) -> ("CYCLE"=w2765:dbl)  [unwired: 2 out]
                        n1699 = Build Array(w2769) -> (w2766:dbl[])
                        n1700 = Build Array(w2768) -> (w2759:dbl[])
                        n1701 = Build Array(w2767) -> (w2754:dbl[])
                        n1702 = Build Array(w2770) -> (w2749:dbl[])
                        n1703 = Build Array(w2780) -> (w2779:dbl[])
                        n1704 = Build Array(w2765) -> (w2744:dbl[])
                        n1705 = TDMS Write(0:w2786, 5:"LAB05-1 TEST VALUES", 7:w2781, 9:w2779) -> (4:w2774:refnum<k34>, 6:w2773:string, 15:w2761:errorcluster)  [unwired: 2 in, 1 out]
                        n1706 = TDMS Write(0:w2774, 5:w2773, 7:w2772, 9:w2766, 11:w2761) -> (4:w2764:refnum<k34>, 6:w2763:string, 15:w2762:errorcluster)  [unwired: 1 in, 1 out]
                        n1707 = TDMS Write(0:w2764, 5:w2763, 7:w2760, 9:w2759, 11:w2762) -> (4:w2758:refnum<k34>, 6:w2757:string, 15:w2756:errorcluster)  [unwired: 1 in, 1 out]
                        n1708 = TDMS Write(0:w2758, 5:w2757, 7:w2755, 9:w2754, 11:w2756) -> (4:w2753:refnum<k34>, 6:w2752:string, 15:w2751:errorcluster)  [unwired: 1 in, 1 out]
                        n1709 = TDMS Write(0:w2753, 5:w2752, 7:w2750, 9:w2749, 11:w2751) -> (4:w2748:refnum<k34>, 6:w2747:string, 15:w2746:errorcluster)  [unwired: 1 in, 1 out]
                        n1710 = TDMS Write(0:w2748, 5:w2747, 7:w2745, 9:w2744, 11:w2746) -> (15:w2743:errorcluster)  [unwired: 1 in, 3 out]
                        n1711 = local write "data file error"(w2743) -> ()
                      }
                    }
                  }
                  frame #9 {
                    # "LAB05-2"
                    n1712 = case shown="True" w2787 {
                      frame False {
                      }
                      frame True {
                        n1713 = local read "LAB05-2 (DISP)"() -> (w2829:T4)
                        n1714 = local read "LAB05-2 (SIG)"() -> (w2830:T2)
                        n1715 = local read "LAB05-2 (TDMS)"() -> (w2831:refnum<k34>)
                        n1716 = Build Array("TEMP Neut") -> (w2795:string[])
                        n1717 = Build Array("CYCLE") -> (w2790:string[])
                        n1718 = Build Array("TEMP Live") -> (w2800:string[])
                        n1719 = Build Array("PF") -> (w2805:string[])
                        n1720 = Build Array("AMPS") -> (w2826:string[])
                        n1721 = Build Array("VOLTS") -> (w2817:string[])
                        n1722 = Unbundle(w2830) -> ("AMPS"=w2825:dbl, "VOLTS"=w2814:dbl, "PF"=w2813:dbl, "Tmp Live"=w2812:dbl, "Tmp Neut"=w2815:dbl)
                        n1723 = Unbundle(w2829) -> ("CYCLE"=w2810:dbl)  [unwired: 2 out]
                        n1724 = Build Array(w2814) -> (w2811:dbl[])
                        n1725 = Build Array(w2813) -> (w2804:dbl[])
                        n1726 = Build Array(w2812) -> (w2799:dbl[])
                        n1727 = Build Array(w2815) -> (w2794:dbl[])
                        n1728 = Build Array(w2825) -> (w2824:dbl[])
                        n1729 = Build Array(w2810) -> (w2789:dbl[])
                        n1730 = TDMS Write(0:w2831, 5:"LAB05-2 TEST VALUES", 7:w2826, 9:w2824) -> (4:w2819:refnum<k34>, 6:w2818:string, 15:w2806:errorcluster)  [unwired: 2 in, 1 out]
                        n1731 = TDMS Write(0:w2819, 5:w2818, 7:w2817, 9:w2811, 11:w2806) -> (4:w2809:refnum<k34>, 6:w2808:string, 15:w2807:errorcluster)  [unwired: 1 in, 1 out]
                        n1732 = TDMS Write(0:w2809, 5:w2808, 7:w2805, 9:w2804, 11:w2807) -> (4:w2803:refnum<k34>, 6:w2802:string, 15:w2801:errorcluster)  [unwired: 1 in, 1 out]
                        n1733 = TDMS Write(0:w2803, 5:w2802, 7:w2800, 9:w2799, 11:w2801) -> (4:w2798:refnum<k34>, 6:w2797:string, 15:w2796:errorcluster)  [unwired: 1 in, 1 out]
                        n1734 = TDMS Write(0:w2798, 5:w2797, 7:w2795, 9:w2794, 11:w2796) -> (4:w2793:refnum<k34>, 6:w2792:string, 15:w2791:errorcluster)  [unwired: 1 in, 1 out]
                        n1735 = TDMS Write(0:w2793, 5:w2792, 7:w2790, 9:w2789, 11:w2791) -> (15:w2788:errorcluster)  [unwired: 1 in, 3 out]
                        n1736 = local write "data file error"(w2788) -> ()
                      }
                    }
                  }
                }
              }
            }
          }
          frame #13 {
            # "check for amps fail"
            # "check for cycle test & temperature rise fail conditions"
            n1737 = local read "on loops"() -> (w2857:dbl)
            n1738 = local read "jig cycle"() -> (w2854:dbl)
            n1739 = local read "jig cycle"() -> (w2859:dbl)
            n1740 = Add(x=w2857, y=3.0) -> (x+y=w2855:dbl)
            n1741 = Equal?(x=w2854, y=w2855) -> (x = y?=w2850:bool)
            n1742 = Equal?(x=w2859, y=1.0) -> (x = y?=w2852:bool)
            n1743 = stacked-sequence {
              tunnel: w2853 -> [w2862 _ _ _ _ _ _ _ _ _]
              tunnel: w2852 -> [w2863 w2882 w2901 w2920 w2939 w2958 w2977 w2996 w3015 w3034]
              tunnel: w2851 -> [w2860 _ _ _ _ _ _ _ _ _]
              tunnel: w2850 -> [w2861 w2881 w2900 w2919 w2938 w2957 w2976 w2995 w3014 w3033]
              tunnel: w2849 -> [_ w2880 _ _ _ _ _ _ _ _]
              tunnel: w2848 -> [_ w2879 _ _ _ _ _ _ _ _]
              tunnel: w2847 -> [_ _ w2899 _ _ _ _ _ _ _]
              tunnel: w2846 -> [_ _ w2898 _ _ _ _ _ _ _]
              tunnel: w2845 -> [_ _ _ w2918 _ _ _ _ _ _]
              tunnel: w2844 -> [_ _ _ w2917 _ _ _ _ _ _]
              tunnel: w2843 -> [_ _ _ _ w2937 _ _ _ _ _]
              tunnel: w2842 -> [_ _ _ _ w2936 _ _ _ _ _]
              tunnel: w2841 -> [_ _ _ _ _ w2956 _ _ _ _]
              tunnel: w2840 -> [_ _ _ _ _ w2955 _ _ _ _]
              tunnel: w2839 -> [_ _ _ _ _ _ w2975 _ _ _]
              tunnel: w2838 -> [_ _ _ _ _ _ w2974 _ _ _]
              tunnel: w2837 -> [_ _ _ _ _ _ _ w2994 _ _]
              tunnel: w2836 -> [_ _ _ _ _ _ _ w2993 _ _]
              tunnel: w2835 -> [_ _ _ _ _ _ _ _ w3013 _]
              tunnel: w2834 -> [_ _ _ _ _ _ _ _ w3012 _]
              tunnel: w2833 -> [_ _ _ _ _ _ _ _ _ w3032]
              tunnel: w2832 -> [_ _ _ _ _ _ _ _ _ w3031]
              frame #0 {
                # "LAB01-1"
                n1744 = case shown="True" w2860 {
                  tunnel: w2863 -> [_ w2875]
                  tunnel: w2862 -> [_ w2872]
                  tunnel: w2861 -> [_ w2871]
                  frame False {
                  }
                  frame True {
                    n1745 = local read "LAB01-1 (TEMP START)"() -> (w2877:cluster{"TL":dbl, "TN":dbl})
                    n1746 = local read "LAB01-1 (RESULT)"() -> (w2864:bool)
                    n1747 = local read "LAB01-1 (FAIL)"() -> (w2868:cluster{"LO":dbl, "HI":dbl})
                    n1748 = local read "LAB01-1 (TDMS)"() -> (w2876:refnum<k34>)
                    n1749 = local read "LAB01-1 (SET)"() -> (w2873:T5)
                    n1750 = local read "LAB01-1 (DISP)"() -> (w2874:T4)
                    n1751 = local read "LAB01-1 (SIG)"() -> (w2878:T2)
                    n1752 = Bundle("LAB01-1 (FAIL)"=w2868, "LAB01-1 (SIG)"=w2878, "LAB01-1 (TEMP START)"=w2877, "LAB01-1 (DISP)"=w2874, "LAB01-1 (SET)"=w2873, "LAB01-1 (TDMS)"=w2876) -> (w2866:T21)  [unwired: 1 in]
                    n1753 = call "sub vi - cycle&temp fail v5.vi"("Amps Lo?"=w2875, "Input Cluster"=w2866, "SELECT"=w2872, "Amps Hi?"=w2871, "Result In"=w2864) -> ("(FAIL) out"=w2867:cluster{"FAIL LO":dbl, "FAIL HI":dbl}, "(DISP) out"=w2870:T4, "Result Out"=w2865:bool, "file error"=w2869:errorcluster)  [unwired: 11 in]
                    n1754 = local write "LAB01-1 (FAIL)"(w2867) -> ()
                    n1755 = local write "LAB01-1 (DISP)"(w2870) -> ()
                    n1756 = local write "LAB01-1 (RESULT)"(w2865) -> ()
                    n1757 = local write "data file error"(w2869) -> ()
                  }
                }
              }
              frame #1 {
                # "LAB01-2"
                n1758 = case shown="True" w2880 {
                  tunnel: w2882 -> [_ w2894]
                  tunnel: w2879 -> [_ w2891]
                  tunnel: w2881 -> [_ w2890]
                  frame False {
                  }
                  frame True {
                    n1759 = local read "LAB01-2 (TEMP START)"() -> (w2896:cluster{"TL":dbl, "TN":dbl})
                    n1760 = local read "LAB01-2 (FAIL)"() -> (w2887:cluster{"LO":dbl, "HI":dbl})
                    n1761 = local read "LAB01-2 (TDMS)"() -> (w2895:refnum<k34>)
                    n1762 = local read "LAB01-2(SET)"() -> (w2892:T5)
                    n1763 = local read "LAB01-2 (DISP)"() -> (w2893:T4)
                    n1764 = local read "LAB01-2 (RESULT)"() -> (w2883:bool)
                    n1765 = local read "LAB01-2 (SIG)"() -> (w2897:T2)
                    n1766 = Bundle("LAB01-2 (FAIL)"=w2887, "LAB01-2 (SIG)"=w2897, "LAB01-2 (TEMP START)"=w2896, "LAB01-2 (DISP)"=w2893, "LAB01-2(SET)"=w2892, "LAB01-2 (TDMS)"=w2895) -> (w2885:T22)  [unwired: 1 in]
                    n1767 = call "sub vi - cycle&temp fail v5.vi"("Amps Lo?"=w2894, "Input Cluster"=w2885, "SELECT"=w2891, "Amps Hi?"=w2890, "Result In"=w2883) -> ("(FAIL) out"=w2886:cluster{"FAIL LO":dbl, "FAIL HI":dbl}, "(DISP) out"=w2889:T4, "Result Out"=w2884:bool, "file error"=w2888:errorcluster)  [unwired: 11 in]
                    n1768 = local write "LAB01-2 (FAIL)"(w2886) -> ()
                    n1769 = local write "LAB01-2 (DISP)"(w2889) -> ()
                    n1770 = local write "LAB01-2 (RESULT)"(w2884) -> ()
                    n1771 = local write "data file error"(w2888) -> ()
                  }
                }
              }
              frame #2 {
                # "LAB02-1"
                n1772 = case shown="True" w2899 {
                  tunnel: w2901 -> [_ w2913]
                  tunnel: w2898 -> [_ w2910]
                  tunnel: w2900 -> [_ w2909]
                  frame False {
                  }
                  frame True {
                    n1773 = local read "LAB02-1 (TEMP START)"() -> (w2915:cluster{"TL":dbl, "TN":dbl})
                    n1774 = local read "LAB02-1 (FAIL)"() -> (w2906:cluster{"LO":dbl, "HI":dbl})
                    n1775 = local read "LAB02-1 (TDMS)"() -> (w2914:refnum<k34>)
                    n1776 = local read "LAB02-1 (SET)"() -> (w2911:T5)
                    n1777 = local read "LAB02-1 (DISP)"() -> (w2912:T4)
                    n1778 = local read "LAB02-1 (SIG)"() -> (w2916:T2)
                    n1779 = local read "LAB02-1 (RESULT)"() -> (w2902:bool)
                    n1780 = Bundle("LAB02-1 (FAIL)"=w2906, "LAB02-1 (SIG)"=w2916, "LAB02-1 (TEMP START)"=w2915, "LAB02-1 (DISP)"=w2912, "LAB02-1 (SET)"=w2911, "LAB02-1 (TDMS)"=w2914) -> (w2904:T23)  [unwired: 1 in]
                    n1781 = call "sub vi - cycle&temp fail v5.vi"("Amps Lo?"=w2913, "Input Cluster"=w2904, "SELECT"=w2910, "Amps Hi?"=w2909, "Result In"=w2902) -> ("(FAIL) out"=w2905:cluster{"FAIL LO":dbl, "FAIL HI":dbl}, "(DISP) out"=w2908:T4, "Result Out"=w2903:bool, "file error"=w2907:errorcluster)  [unwired: 11 in]
                    n1782 = local write "LAB02-1 (FAIL)"(w2905) -> ()
                    n1783 = local write "LAB02-1 (DISP)"(w2908) -> ()
                    n1784 = local write "LAB02-1 (RESULT)"(w2903) -> ()
                    n1785 = local write "data file error"(w2907) -> ()
                  }
                }
              }
              frame #3 {
                # "LAB02-2"
                n1786 = case shown="True" w2918 {
                  tunnel: w2920 -> [_ w2932]
                  tunnel: w2917 -> [_ w2929]
                  tunnel: w2919 -> [_ w2928]
                  frame False {
                  }
                  frame True {
                    n1787 = local read "LAB02-2 (TEMP START)"() -> (w2934:cluster{"TL":dbl, "TN":dbl})
                    n1788 = local read "LAB02-2 (FAIL)"() -> (w2925:cluster{"LO":dbl, "HI":dbl})
                    n1789 = local read "LAB02-2 (TDMS)"() -> (w2933:refnum<k34>)
                    n1790 = local read "LAB02-2 (SET)"() -> (w2930:T5)
                    n1791 = local read "LAB02-2 (DISP)"() -> (w2931:T4)
                    n1792 = local read "LAB02-2 (SIG)"() -> (w2935:T2)
                    n1793 = local read "LAB02-2 (RESULT)"() -> (w2921:bool)
                    n1794 = Bundle("LAB02-2 (FAIL)"=w2925, "LAB02-2 (SIG)"=w2935, "LAB02-2 (TEMP START)"=w2934, "LAB02-2 (DISP)"=w2931, "LAB02-2 (SET)"=w2930, "LAB02-2 (TDMS)"=w2933) -> (w2923:T24)  [unwired: 1 in]
                    n1795 = call "sub vi - cycle&temp fail v5.vi"("Amps Lo?"=w2932, "Input Cluster"=w2923, "SELECT"=w2929, "Amps Hi?"=w2928, "Result In"=w2921) -> ("(FAIL) out"=w2924:cluster{"FAIL LO":dbl, "FAIL HI":dbl}, "(DISP) out"=w2927:T4, "Result Out"=w2922:bool, "file error"=w2926:errorcluster)  [unwired: 11 in]
                    n1796 = local write "LAB02-2 (FAIL)"(w2924) -> ()
                    n1797 = local write "LAB02-2 (DISP)"(w2927) -> ()
                    n1798 = local write "LAB02-2 (RESULT)"(w2922) -> ()
                    n1799 = local write "data file error"(w2926) -> ()
                  }
                }
              }
              frame #4 {
                # "LAB03-1"
                n1800 = case shown="True" w2937 {
                  tunnel: w2939 -> [_ w2951]
                  tunnel: w2936 -> [_ w2948]
                  tunnel: w2938 -> [_ w2947]
                  frame False {
                  }
                  frame True {
                    n1801 = local read "LAB03-1 (TEMP START)"() -> (w2953:cluster{"TL":dbl, "TN":dbl})
                    n1802 = local read "LAB03-1 (FAIL)"() -> (w2944:cluster{"LO":dbl, "HI":dbl})
                    n1803 = local read "LAB03-1 (TDMS)"() -> (w2952:refnum<k34>)
                    n1804 = local read "LAB03-1 (SET)"() -> (w2949:T5)
                    n1805 = local read "LAB03-1 (DISP)"() -> (w2950:T4)
                    n1806 = local read "LAB03-1 (SIG)"() -> (w2954:T2)
                    n1807 = local read "LAB03-1 (RESULT)"() -> (w2940:bool)
                    n1808 = Bundle("LAB03-1 (FAIL)"=w2944, "LAB03-1 (SIG)"=w2954, "LAB03-1 (TEMP START)"=w2953, "LAB03-1 (DISP)"=w2950, "LAB03-1 (SET)"=w2949, "LAB03-1 (TDMS)"=w2952) -> (w2942:T25)  [unwired: 1 in]
                    n1809 = call "sub vi - cycle&temp fail v5.vi"("Amps Lo?"=w2951, "Input Cluster"=w2942, "SELECT"=w2948, "Amps Hi?"=w2947, "Result In"=w2940) -> ("(FAIL) out"=w2943:cluster{"FAIL LO":dbl, "FAIL HI":dbl}, "(DISP) out"=w2946:T4, "Result Out"=w2941:bool, "file error"=w2945:errorcluster)  [unwired: 11 in]
                    n1810 = local write "LAB03-1 (FAIL)"(w2943) -> ()
                    n1811 = local write "LAB03-1 (DISP)"(w2946) -> ()
                    n1812 = local write "LAB03-1 (RESULT)"(w2941) -> ()
                    n1813 = local write "data file error"(w2945) -> ()
                  }
                }
              }
              frame #5 {
                # "LAB03-2"
                n1814 = case shown="True" w2956 {
                  tunnel: w2958 -> [_ w2970]
                  tunnel: w2955 -> [_ w2967]
                  tunnel: w2957 -> [_ w2966]
                  frame False {
                  }
                  frame True {
                    n1815 = local read "LAB03-2 (TEMP START)"() -> (w2972:cluster{"TL":dbl, "TN":dbl})
                    n1816 = local read "LAB03-2 (FAIL)"() -> (w2963:cluster{"LO":dbl, "HI":dbl})
                    n1817 = local read "LAB03-2 (TDMS)"() -> (w2971:refnum<k34>)
                    n1818 = local read "LAB03-2 (SET)"() -> (w2968:T5)
                    n1819 = local read "LAB03-2 (DISP)"() -> (w2969:T4)
                    n1820 = local read "LAB03-2 (RESULT)"() -> (w2959:bool)
                    n1821 = local read "LAB03-2 (SIG)"() -> (w2973:T2)
                    n1822 = Bundle("LAB03-2 (FAIL)"=w2963, "LAB03-2 (SIG)"=w2973, "LAB03-2 (TEMP START)"=w2972, "LAB03-2 (DISP)"=w2969, "LAB03-2 (SET)"=w2968, "LAB03-2 (TDMS)"=w2971) -> (w2961:T26)  [unwired: 1 in]
                    n1823 = call "sub vi - cycle&temp fail v5.vi"("Amps Lo?"=w2970, "Input Cluster"=w2961, "SELECT"=w2967, "Amps Hi?"=w2966, "Result In"=w2959) -> ("(FAIL) out"=w2962:cluster{"FAIL LO":dbl, "FAIL HI":dbl}, "(DISP) out"=w2965:T4, "Result Out"=w2960:bool, "file error"=w2964:errorcluster)  [unwired: 11 in]
                    n1824 = local write "LAB03-2 (FAIL)"(w2962) -> ()
                    n1825 = local write "LAB03-2 (DISP)"(w2965) -> ()
                    n1826 = local write "LAB03-2 (RESULT)"(w2960) -> ()
                    n1827 = local write "data file error"(w2964) -> ()
                  }
                }
              }
              frame #6 {
                # "LAB04-1"
                n1828 = case shown="True" w2975 {
                  tunnel: w2977 -> [_ w2989]
                  tunnel: w2974 -> [_ w2986]
                  tunnel: w2976 -> [_ w2985]
                  frame False {
                  }
                  frame True {
                    n1829 = local read "LAB04-1 (TEMP START)"() -> (w2991:cluster{"TL":dbl, "TN":dbl})
                    n1830 = local read "LAB04-1 (FAIL)"() -> (w2982:cluster{"LO":dbl, "HI":dbl})
                    n1831 = local read "LAB04-1 (TDMS)"() -> (w2990:refnum<k34>)
                    n1832 = local read "LAB04-1 (SET)"() -> (w2987:T5)
                    n1833 = local read "LAB04-1 (DISP)"() -> (w2988:T4)
                    n1834 = local read "LAB04-1 (SIG)"() -> (w2992:T2)
                    n1835 = local read "LAB04-1 (RESULT)"() -> (w2978:bool)
                    n1836 = Bundle("LAB04-1 (FAIL)"=w2982, "LAB04-1 (SIG)"=w2992, "LAB04-1 (TEMP START)"=w2991, "LAB04-1 (DISP)"=w2988, "LAB04-1 (SET)"=w2987, "LAB04-1 (TDMS)"=w2990) -> (w2980:T27)  [unwired: 1 in]
                    n1837 = call "sub vi - cycle&temp fail v5.vi"("Amps Lo?"=w2989, "Input Cluster"=w2980, "SELECT"=w2986, "Amps Hi?"=w2985, "Result In"=w2978) -> ("(FAIL) out"=w2981:cluster{"FAIL LO":dbl, "FAIL HI":dbl}, "(DISP) out"=w2984:T4, "Result Out"=w2979:bool, "file error"=w2983:errorcluster)  [unwired: 11 in]
                    n1838 = local write "LAB04-1 (FAIL)"(w2981) -> ()
                    n1839 = local write "LAB04-1 (DISP)"(w2984) -> ()
                    n1840 = local write "LAB04-1 (RESULT)"(w2979) -> ()
                    n1841 = local write "data file error"(w2983) -> ()
                  }
                }
              }
              frame #7 {
                # "LAB04-2"
                n1842 = case shown="True" w2994 {
                  tunnel: w2996 -> [_ w3008]
                  tunnel: w2993 -> [_ w3005]
                  tunnel: w2995 -> [_ w3004]
                  frame False {
                  }
                  frame True {
                    n1843 = local read "LAB04-2 (TEMP START)"() -> (w3010:cluster{"TL":dbl, "TN":dbl})
                    n1844 = local read "LAB04-2 (FAIL)"() -> (w3001:cluster{"LO":dbl, "HI":dbl})
                    n1845 = local read "LAB04-2 (TDMS)"() -> (w3009:refnum<k34>)
                    n1846 = local read "LAB04-2 (SET)"() -> (w3006:T5)
                    n1847 = local read "LAB04-2 (DISP)"() -> (w3007:T4)
                    n1848 = local read "LAB04-2 (SIG)"() -> (w3011:T2)
                    n1849 = local read "LAB04-2 (RESULT)"() -> (w2997:bool)
                    n1850 = Bundle("LAB04-2 (FAIL)"=w3001, "LAB04-2 (SIG)"=w3011, "LAB04-2 (TEMP START)"=w3010, "LAB04-2 (DISP)"=w3007, "LAB04-2 (SET)"=w3006, "LAB04-2 (TDMS)"=w3009) -> (w2999:T28)  [unwired: 1 in]
                    n1851 = call "sub vi - cycle&temp fail v5.vi"("Amps Lo?"=w3008, "Input Cluster"=w2999, "SELECT"=w3005, "Amps Hi?"=w3004, "Result In"=w2997) -> ("(FAIL) out"=w3000:cluster{"FAIL LO":dbl, "FAIL HI":dbl}, "(DISP) out"=w3003:T4, "Result Out"=w2998:bool, "file error"=w3002:errorcluster)  [unwired: 11 in]
                    n1852 = local write "LAB04-2 (FAIL)"(w3000) -> ()
                    n1853 = local write "LAB04-2 (DISP)"(w3003) -> ()
                    n1854 = local write "LAB04-2 (RESULT)"(w2998) -> ()
                    n1855 = local write "data file error"(w3002) -> ()
                  }
                }
              }
              frame #8 {
                # "LAB05-1"
                n1856 = case shown="True" w3013 {
                  tunnel: w3015 -> [_ w3027]
                  tunnel: w3012 -> [_ w3024]
                  tunnel: w3014 -> [_ w3023]
                  frame False {
                  }
                  frame True {
                    n1857 = local read "LAB05-1 (TEMP START)"() -> (w3029:cluster{"TL":dbl, "TN":dbl})
                    n1858 = local read "LAB05-1 (FAIL)"() -> (w3020:cluster{"LO":dbl, "HI":dbl})
                    n1859 = local read "LAB05-1 (TDMS)"() -> (w3028:refnum<k34>)
                    n1860 = local read "LAB05-1 (SET)"() -> (w3025:T5)
                    n1861 = local read "LAB05-1 (DISP)"() -> (w3026:T4)
                    n1862 = local read "LAB05-1 (SIG)"() -> (w3030:T2)
                    n1863 = local read "LAB05-1 (RESULT)"() -> (w3016:bool)
                    n1864 = Bundle("LAB05-1 (FAIL)"=w3020, "LAB05-1 (SIG)"=w3030, "LAB05-1 (TEMP START)"=w3029, "LAB05-1 (DISP)"=w3026, "LAB05-1 (SET)"=w3025, "LAB05-1 (TDMS)"=w3028) -> (w3018:T29)  [unwired: 1 in]
                    n1865 = call "sub vi - cycle&temp fail v5.vi"("Amps Lo?"=w3027, "Input Cluster"=w3018, "SELECT"=w3024, "Amps Hi?"=w3023, "Result In"=w3016) -> ("(FAIL) out"=w3019:cluster{"FAIL LO":dbl, "FAIL HI":dbl}, "(DISP) out"=w3022:T4, "Result Out"=w3017:bool, "file error"=w3021:errorcluster)  [unwired: 11 in]
                    n1866 = local write "LAB05-1 (FAIL)"(w3019) -> ()
                    n1867 = local write "LAB05-1 (DISP)"(w3022) -> ()
                    n1868 = local write "LAB05-1 (RESULT)"(w3017) -> ()
                    n1869 = local write "data file error"(w3021) -> ()
                  }
                }
              }
              frame #9 {
                # "LAB05-2"
                n1870 = case shown="True" w3032 {
                  tunnel: w3034 -> [_ w3046]
                  tunnel: w3031 -> [_ w3043]
                  tunnel: w3033 -> [_ w3042]
                  frame False {
                  }
                  frame True {
                    n1871 = local read "LAB05-2 (TEMP START)"() -> (w3048:cluster{"TL":dbl, "TN":dbl})
                    n1872 = local read "LAB05-2 (FAIL)"() -> (w3039:cluster{"LO":dbl, "HI":dbl})
                    n1873 = local read "LAB05-2 (TDMS)"() -> (w3047:refnum<k34>)
                    n1874 = local read "LAB05-2 (SET)"() -> (w3044:T5)
                    n1875 = local read "LAB05-2 (DISP)"() -> (w3045:T4)
                    n1876 = local read "LAB05-2 (SIG)"() -> (w3049:T2)
                    n1877 = local read "LAB05-2 (RESULT)"() -> (w3035:bool)
                    n1878 = Bundle("LAB05-2 (FAIL)"=w3039, "LAB05-2 (SIG)"=w3049, "LAB05-2 (TEMP START)"=w3048, "LAB05-2 (DISP)"=w3045, "LAB05-2 (SET)"=w3044, "LAB05-2 (TDMS)"=w3047) -> (w3037:T30)  [unwired: 1 in]
                    n1879 = call "sub vi - cycle&temp fail v5.vi"("Amps Lo?"=w3046, "Input Cluster"=w3037, "SELECT"=w3043, "Amps Hi?"=w3042, "Result In"=w3035) -> ("(FAIL) out"=w3038:cluster{"FAIL LO":dbl, "FAIL HI":dbl}, "(DISP) out"=w3041:T4, "Result Out"=w3036:bool, "file error"=w3040:errorcluster)  [unwired: 11 in]
                    n1880 = local write "LAB05-2 (FAIL)"(w3038) -> ()
                    n1881 = local write "LAB05-2 (DISP)"(w3041) -> ()
                    n1882 = local write "LAB05-2 (RESULT)"(w3036) -> ()
                    n1883 = local write "data file error"(w3040) -> ()
                  }
                }
              }
            }
          }
          frame #14 {
            # "run calibration routine"
            n1884 = local read "CALIBRATE"() -> (w3050:bool)
            n1885 = case shown="True" w3050 {
              frame False {
              }
              frame True {
                n1886 = stacked-sequence {
                  seq-local: [w3051 _ _] -> [_ w3053 _]
                  frame #0 {
                    n1887 = call "CALIBRATION PASSWORD"() -> ("PASSWORD"=w3051:string)  [unwired: 17 in, 2 out]
                  }
                  frame #1 {
                    n1888 = Equal?(x=w3053, y="7777") -> (x = y?=w3052:bool)
                    n1889 = case shown="True" w3052 {
                      frame False {
                      }
                      frame True {
                        n1890 = stacked-sequence {
                          frame #0 {
                            n1891 = call "sub vi - calibration v1.vi"() -> ()  [unwired: 12 in]
                          }
                          frame #1 {
                            n1892 = call "sub vi - get calibration values v1.vi"() -> ("LAB01 (CAL)"=w3059:T6, "LAB02 (CAL)"=w3058:T7, "LAB03 (CAL)"=w3057:T6, "LAB04 (CAL)"=w3056:T6, "calibration file error out"=w3060:errorcluster, "LAB05 (CAL)"=w3055:T6)  [unwired: 10 in]
                            n1893 = local write "calibration file error out"(w3060) -> ()
                            n1894 = local write "LAB04 (CAL)"(w3056) -> ()
                            n1895 = local write "LAB05 (CAL)"(w3055) -> ()
                            n1896 = local write "LAB01 (CAL)"(w3059) -> ()
                            n1897 = local write "LAB02 (CAL)"(w3058) -> ()
                            n1898 = local write "LAB03 (CAL)"(w3057) -> ()
                          }
                        }
                      }
                    }
                  }
                  frame #2 {
                    n1899 = local write "CALIBRATE"(FALSE) -> ()
                  }
                }
              }
            }
          }
        }
        n1900 = node-c288() -> ()  [unwired: 1 in, 1 out]
        "loops" <- w36
      }
      n1901 = node-c288(w13) -> ()  [unwired: 1 out]
    }
  }
